vi "Strategy 5_Autotuning PID_With GUI.vi"() -> ()   [LabVIEW 2019]
doc: "This example demonstrates how to use the PID Design function to obtain PID parameters based on measured process."
uses:
  <vilib>/addons/control/pid/NI_PID_autopid.lvlib
  <vilib>/addons/control/pid/NI_PID_pid.lvlib
  <vilib>/ptbypt/NI_PtbyPt.lvlib
  <vilib>/DAQmx/create/channels.llb/DAQmx Create Channel (DO-Digital Output).vi
  <vilib>/DAQmx/write.llb/DAQmx Write (Digital 1D Bool 1Chan 1Samp).vi
  <vilib>/Instr/_visa.llb/VISA Configure Serial Port (Instr).vi
  <vilib>/addons/control/pid/autopid.llb/PID Autotuning Design (Cohen-Coon).vi
  <vilib>/addons/control/pid/autopid.llb/PID Autotuning Design (Ziegler-Nichols).vi
  <vilib>/addons/control/pid/autopid.llb/PID Autotuning Design (Chien-Hrones-Reswick).vi
  <vilib>/addons/control/pid/autopid.llb/PID Autotuning Design (Internal Model Control).vi
  <vilib>/addons/control/pid/pid.llb/PID Advanced (DBL).vi
  <vilib>/DAQmx/read.llb/DAQmx Read (Analog 1D DBL NChan 1Samp).vi
panel:
  out "Position Sensor Data 2":cluster{dbl, "x":sgl}[](graph)
  out "?":bool
  in  "Muscle Control":T1(tab)=enum."M-11"
  out "Tuned PID gains 12":T2={"proportional gain (Kc)"=1.9838195929127882, "integral time (Ti, min)"=0.01995856284686879, "derivative time (Td, min)"=0.0} {"derivative time (Td, min)" format="%#.6g"; "integral time (Ti, min)" format="%#.6g"; "proportional gain (Kc)" format="%#.6g"}
  in  "Accept gain 12":bool
  in  "Control 12":T3(tab)
  in  "Ziegler-Nichols speed 12":u16(ring) items=["Fast", "Normal", "Slow"]
  in  "Tuning specifications 12":u16(ring) items=["Regulator - 0 %", "Regulator -  20%", "Servo - 0%", "Servo - 20%"]
  in  "Multiplicative factor 12":dbl(slide)=1.0 scale=0.01..100.0
  in  "Type of controller 12":u16(ring)=2 items=["P", "PI", "PID"]
  in  "Stop 12":bool
  in  "PID Gains 12":T2={"proportional gain (Kc)"=0.1625, "integral time (Ti, min)"=1.25, "derivative time (Td, min)"=0.0} {"derivative time (Td, min)" format="%#.6g"; "integral time (Ti, min)" format="%#.6g"; "proportional gain (Kc)" format="%#.6g"}
  in  "Autotune 12":bool
  in  "Reinitialize 12":bool
  in  "Excitation 12":dbl=0.5 format="%.2f"
  in  "Automatic 12":bool=TRUE
  in  "MV: 12":dbl(slide)=20.39115328927357 scale=-100.0..100.0
  in  "Set Point 12":dbl(slide) scale=0.0..30.0
  out "PWM Output 12":bool
  out "Real time Data 12":dbl[][](graph)
  in  "Median sample length 21":i32=100
  in  "INLET 1 ON/OFF 3":bool=TRUE
  out "Tuned PID gains 11":T2={"proportional gain (Kc)"=1.9838195929127882, "integral time (Ti, min)"=0.01995856284686879, "derivative time (Td, min)"=0.0} {"derivative time (Td, min)" format="%#.6g"; "integral time (Ti, min)" format="%#.6g"; "proportional gain (Kc)" format="%#.6g"}
  in  "Accept gain 11":bool
  in  "Control 11":T3(tab)
  in  "Ziegler-Nichols speed 11":u16(ring) items=["Fast", "Normal", "Slow"]
  in  "Tuning specifications 11":u16(ring) items=["Regulator - 0 %", "Regulator -  20%", "Servo - 0%", "Servo - 20%"]
  in  "Multiplicative factor 11":dbl(slide)=1.0 scale=0.01..100.0
  in  "Type of controller 11":u16(ring)=2 items=["P", "PI", "PID"]
  in  "Excitation 11":dbl=0.5 format="%.2f"
  in  "Stop 11":bool
  in  "PID Gains 11":T2={"proportional gain (Kc)"=0.1625, "integral time (Ti, min)"=1.25, "derivative time (Td, min)"=0.0} {"derivative time (Td, min)" format="%#.6g"; "integral time (Ti, min)" format="%#.6g"; "proportional gain (Kc)" format="%#.6g"}
  in  "Autotune 11":bool
  in  "Reinitialize 11":bool
  in  "Automatic 11":bool=TRUE
  in  "MV: 11":dbl(slide)=20.39115328927357 scale=-100.0..100.0
  in  "Set Point 11":dbl(slide) scale=0.0..30.0
  out "PWM Output 11":bool
  out "Real time Data 11":dbl[][](graph)
  in  "Median sample length 20":i32=100
  in  "INLET 5 ON/OFF 3":bool=TRUE
  out "Tuned PID gains 10":T2={"proportional gain (Kc)"=1.9838195929127882, "integral time (Ti, min)"=0.01995856284686879, "derivative time (Td, min)"=0.0} {"derivative time (Td, min)" format="%#.6g"; "integral time (Ti, min)" format="%#.6g"; "proportional gain (Kc)" format="%#.6g"}
  in  "Accept gain 10":bool
  in  "Control 10":T3(tab)
  in  "Ziegler-Nichols speed 10":u16(ring) items=["Fast", "Normal", "Slow"]
  in  "Tuning specifications 10":u16(ring) items=["Regulator - 0 %", "Regulator -  20%", "Servo - 0%", "Servo - 20%"]
  in  "Multiplicative factor 10":dbl(slide)=1.0 scale=0.01..100.0
  in  "Type of controller 10":u16(ring)=2 items=["P", "PI", "PID"]
  in  "Stop 10":bool
  in  "PID Gains 10":T2={"proportional gain (Kc)"=0.1625, "integral time (Ti, min)"=1.25, "derivative time (Td, min)"=0.0} {"derivative time (Td, min)" format="%#.6g"; "integral time (Ti, min)" format="%#.6g"; "proportional gain (Kc)" format="%#.6g"}
  in  "Autotune 10":bool
  in  "Reinitialize 10":bool
  in  "Excitation 10":dbl=0.5 format="%.2f"
  in  "Automatic 10":bool=TRUE
  in  "MV: 10":dbl(slide)=20.39115328927357 scale=-100.0..100.0
  in  "Set Point 10":dbl(slide) scale=0.0..30.0
  out "PWM Output 10":bool
  out "Real time Data 10":dbl[][](graph)
  in  "Median sample length 19":i32=100
  in  "INLET 3 ON/OFF 3":bool=TRUE
  out "Tuned PID gains 9":T2={"proportional gain (Kc)"=1.9838195929127882, "integral time (Ti, min)"=0.01995856284686879, "derivative time (Td, min)"=0.0} {"derivative time (Td, min)" format="%#.6g"; "integral time (Ti, min)" format="%#.6g"; "proportional gain (Kc)" format="%#.6g"}
  in  "Accept gain 9":bool
  in  "Type of controller 9":u16(ring)=2 items=["P", "PI", "PID"]
  in  "Excitation 9":dbl=0.5 format="%.2f"
  in  "Control 9":T3(tab)
  in  "Ziegler-Nichols speed 9":u16(ring) items=["Fast", "Normal", "Slow"]
  in  "Tuning specifications 9":u16(ring) items=["Regulator - 0 %", "Regulator -  20%", "Servo - 0%", "Servo - 20%"]
  in  "Multiplicative factor 9":dbl(slide)=1.0 scale=0.01..100.0
  in  "Stop 9":bool
  in  "PID Gains 9":T2={"proportional gain (Kc)"=0.1625, "integral time (Ti, min)"=1.25, "derivative time (Td, min)"=0.0} {"derivative time (Td, min)" format="%#.6g"; "integral time (Ti, min)" format="%#.6g"; "proportional gain (Kc)" format="%#.6g"}
  in  "Autotune 9":bool
  in  "Reinitialize 9":bool
  in  "Automatic 9":bool=TRUE
  in  "MV: 9":dbl(slide)=20.39115328927357 scale=-100.0..100.0
  in  "Set Point 9":dbl(slide) scale=0.0..30.0
  out "PWM Output 9":bool
  out "Real time Data 9":dbl[][](graph)
  in  "Median sample length 18":i32=100
  in  "INLET 10 ON/OFF 2":bool=TRUE
  out "Tuned PID gains 8":T2={"proportional gain (Kc)"=1.9838195929127882, "integral time (Ti, min)"=0.01995856284686879, "derivative time (Td, min)"=0.0} {"derivative time (Td, min)" format="%#.6g"; "integral time (Ti, min)" format="%#.6g"; "proportional gain (Kc)" format="%#.6g"}
  in  "Accept gain 8":bool
  in  "Control 8":T3(tab)
  in  "Ziegler-Nichols speed 8":u16(ring) items=["Fast", "Normal", "Slow"]
  in  "Tuning specifications 8":u16(ring) items=["Regulator - 0 %", "Regulator -  20%", "Servo - 0%", "Servo - 20%"]
  in  "Multiplicative factor 8":dbl(slide)=1.0 scale=0.01..100.0
  in  "Type of controller 8":u16(ring)=2 items=["P", "PI", "PID"]
  in  "Stop 8":bool
  in  "PID Gains 8":T2={"proportional gain (Kc)"=0.1625, "integral time (Ti, min)"=1.25, "derivative time (Td, min)"=0.0} {"derivative time (Td, min)" format="%#.6g"; "integral time (Ti, min)" format="%#.6g"; "proportional gain (Kc)" format="%#.6g"}
  in  "Autotune 8":bool
  in  "Reinitialize 8":bool
  in  "Excitation 8":dbl=0.5 format="%.2f"
  in  "Automatic 8":bool=TRUE
  in  "MV: 8":dbl(slide)=20.39115328927357 scale=-100.0..100.0
  in  "Set Point 8":dbl(slide) scale=0.0..30.0
  out "PWM Output 8":bool
  out "Real time Data 8":dbl[][](graph)
  in  "Median sample length 17":i32=100
  in  "INLET 2 ON/OFF 2":bool=TRUE
  out "Tuned PID gains 7":T2={"proportional gain (Kc)"=1.9838195929127882, "integral time (Ti, min)"=0.01995856284686879, "derivative time (Td, min)"=0.0} {"derivative time (Td, min)" format="%#.6g"; "integral time (Ti, min)" format="%#.6g"; "proportional gain (Kc)" format="%#.6g"}
  in  "Accept gain 7":bool
  in  "Control 7":T3(tab)
  in  "Ziegler-Nichols speed 7":u16(ring) items=["Fast", "Normal", "Slow"]
  in  "Tuning specifications 7":u16(ring) items=["Regulator - 0 %", "Regulator -  20%", "Servo - 0%", "Servo - 20%"]
  in  "Multiplicative factor 7":dbl(slide)=1.0 scale=0.01..100.0
  in  "Type of controller 7":u16(ring)=2 items=["P", "PI", "PID"]
  in  "Stop 7":bool
  in  "PID Gains 7":T2={"proportional gain (Kc)"=0.1625, "integral time (Ti, min)"=1.25, "derivative time (Td, min)"=0.0} {"derivative time (Td, min)" format="%#.6g"; "integral time (Ti, min)" format="%#.6g"; "proportional gain (Kc)" format="%#.6g"}
  in  "Autotune 7":bool
  in  "Reinitialize 7":bool
  in  "Excitation 7":dbl=0.5 format="%.2f"
  in  "Automatic 7":bool=TRUE
  in  "MV: 7":dbl(slide)=20.39115328927357 scale=-100.0..100.0
  in  "Set Point 7":dbl(slide) scale=0.0..30.0
  out "PWM Output 7":bool
  out "Real time Data 7":dbl[][](graph)
  in  "Median sample length 16":i32=100
  in  "INLET 7 ON/OFF 2":bool=TRUE
  out "Tuned PID gains 6":T2={"proportional gain (Kc)"=1.9838195929127882, "integral time (Ti, min)"=0.01995856284686879, "derivative time (Td, min)"=0.0} {"derivative time (Td, min)" format="%#.6g"; "integral time (Ti, min)" format="%#.6g"; "proportional gain (Kc)" format="%#.6g"}
  in  "Accept gain 6":bool
  in  "Control 6":T3(tab)
  in  "Ziegler-Nichols speed 6":u16(ring) items=["Fast", "Normal", "Slow"]
  in  "Tuning specifications 6":u16(ring) items=["Regulator - 0 %", "Regulator -  20%", "Servo - 0%", "Servo - 20%"]
  in  "Multiplicative factor 6":dbl(slide)=1.0 scale=0.01..100.0
  in  "Type of controller 6":u16(ring)=2 items=["P", "PI", "PID"]
  in  "Stop 6":bool
  in  "PID Gains 6":T2={"proportional gain (Kc)"=0.1625, "integral time (Ti, min)"=1.25, "derivative time (Td, min)"=0.0} {"derivative time (Td, min)" format="%#.6g"; "integral time (Ti, min)" format="%#.6g"; "proportional gain (Kc)" format="%#.6g"}
  in  "Autotune 6":bool
  in  "Reinitialize 6":bool
  in  "Excitation 6":dbl=0.5 format="%.2f"
  in  "Automatic 6":bool=TRUE
  in  "MV: 6":dbl(slide)=20.39115328927357 scale=-100.0..100.0
  in  "Set Point 6":dbl(slide) scale=0.0..30.0
  out "PWM Output 6":bool
  out "Real time Data 6":dbl[][](graph)
  in  "Median sample length 15":i32=100
  in  "INLET 6 ON/OFF 2":bool=TRUE
  out "Tuned PID gains 5":T2={"proportional gain (Kc)"=1.9838195929127882, "integral time (Ti, min)"=0.01995856284686879, "derivative time (Td, min)"=0.0} {"derivative time (Td, min)" format="%#.6g"; "integral time (Ti, min)" format="%#.6g"; "proportional gain (Kc)" format="%#.6g"}
  in  "Accept gain 5":bool
  in  "Control 5":T3(tab)
  in  "Ziegler-Nichols speed 5":u16(ring) items=["Fast", "Normal", "Slow"]
  in  "Tuning specifications 5":u16(ring) items=["Regulator - 0 %", "Regulator -  20%", "Servo - 0%", "Servo - 20%"]
  in  "Multiplicative factor 5":dbl(slide)=1.0 scale=0.01..100.0
  in  "Type of controller 5":u16(ring)=2 items=["P", "PI", "PID"]
  in  "Stop 5":bool
  in  "PID Gains 5":T2={"proportional gain (Kc)"=0.1625, "integral time (Ti, min)"=1.25, "derivative time (Td, min)"=0.0} {"derivative time (Td, min)" format="%#.6g"; "integral time (Ti, min)" format="%#.6g"; "proportional gain (Kc)" format="%#.6g"}
  in  "Autotune 5":bool
  in  "Reinitialize 5":bool
  in  "Excitation 5":dbl=0.5 format="%.2f"
  in  "Automatic 5":bool=TRUE
  in  "MV: 5":dbl(slide)=20.39115328927357 scale=-100.0..100.0
  in  "Set Point 5":dbl(slide) scale=0.0..30.0
  out "PWM Output 5":bool
  out "Real time Data 5":dbl[][](graph)
  in  "Median sample length 14":i32=100
  in  "INLET 8 ON/OFF 2":bool=TRUE
  out "Tuned PID gains 4":T2={"proportional gain (Kc)"=1.9838195929127882, "integral time (Ti, min)"=0.01995856284686879, "derivative time (Td, min)"=0.0} {"derivative time (Td, min)" format="%#.6g"; "integral time (Ti, min)" format="%#.6g"; "proportional gain (Kc)" format="%#.6g"}
  in  "Accept gain 4":bool
  in  "Control 4":T3(tab)
  in  "Ziegler-Nichols speed 4":u16(ring) items=["Fast", "Normal", "Slow"]
  in  "Tuning specifications 4":u16(ring) items=["Regulator - 0 %", "Regulator -  20%", "Servo - 0%", "Servo - 20%"]
  in  "Multiplicative factor 4":dbl(slide)=1.0 scale=0.01..100.0
  in  "Type of controller 4":u16(ring)=2 items=["P", "PI", "PID"]
  in  "Stop 4":bool
  in  "PID Gains 4":T2={"proportional gain (Kc)"=0.1625, "integral time (Ti, min)"=1.25, "derivative time (Td, min)"=0.0} {"derivative time (Td, min)" format="%#.6g"; "integral time (Ti, min)" format="%#.6g"; "proportional gain (Kc)" format="%#.6g"}
  in  "Autotune 4":bool
  in  "Reinitialize 4":bool
  in  "Excitation 4":dbl=0.5 format="%.2f"
  in  "Automatic 4":bool=TRUE
  in  "MV: 4":dbl(slide)=20.39115328927357 scale=-100.0..100.0
  in  "Set Point 4":dbl(slide) scale=0.0..30.0
  out "PWM Output 4":bool
  out "Real time Data 4":dbl[][](graph)
  in  "Median sample length 9":i32=100
  in  "INLET 9 ON/OFF 2":bool=TRUE
  out "Tuned PID gains 3":T2={"proportional gain (Kc)"=1.9838195929127882, "integral time (Ti, min)"=0.01995856284686879, "derivative time (Td, min)"=0.0} {"derivative time (Td, min)" format="%#.6g"; "integral time (Ti, min)" format="%#.6g"; "proportional gain (Kc)" format="%#.6g"}
  in  "Accept gain 3":bool
  in  "Control 3":T3(tab)
  in  "Ziegler-Nichols speed 3":u16(ring) items=["Fast", "Normal", "Slow"]
  in  "Tuning specifications 3":u16(ring) items=["Regulator - 0 %", "Regulator -  20%", "Servo - 0%", "Servo - 20%"]
  in  "Multiplicative factor 3":dbl(slide)=1.0 scale=0.01..100.0
  in  "Type of controller 3":u16(ring)=2 items=["P", "PI", "PID"]
  in  "Stop 3":bool
  in  "PID Gains 3":T2={"proportional gain (Kc)"=0.1625, "integral time (Ti, min)"=1.25, "derivative time (Td, min)"=0.0} {"derivative time (Td, min)" format="%#.6g"; "integral time (Ti, min)" format="%#.6g"; "proportional gain (Kc)" format="%#.6g"}
  in  "Autotune 3":bool
  in  "Reinitialize 3":bool
  in  "Excitation 3":dbl=0.5 format="%.2f"
  in  "Automatic 3":bool=TRUE
  in  "MV: 3":dbl(slide)=20.39115328927357 scale=-100.0..100.0
  in  "Set Point 3":dbl(slide) scale=0.0..30.0
  out "PWM Output 3":bool
  out "Real time Data 3":dbl[][](graph)
  in  "Median sample length 13":i32=100
  in  "INLET 10 ON/OFF":bool=TRUE
  in  "INLET":bool=TRUE
  out "PWM Output":bool
  out "Real time Data":dbl[][](graph)
  in  "MV:":dbl(slide)=20.39115328927357 scale=-100.0..100.0
  in  "Set Point":dbl(slide) scale=0.0..30.0
  in  "Median sample length":i32=100
  in  "Excitation":dbl=0.5 format="%.2f"
  in  "Type of controller":u16(ring)=2 items=["P", "PI", "PID"]
  in  "Control":T3(tab)
  in  "Ziegler-Nichols speed":u16(ring) items=["Fast", "Normal", "Slow"]
  in  "Tuning specifications":u16(ring) items=["Regulator - 0 %", "Regulator -  20%", "Servo - 0%", "Servo - 20%"]
  in  "Multiplicative factor":dbl(slide)=1.0 scale=0.01..100.0
  in  "Automatic":bool=TRUE
  in  "Reinitialize":bool
  in  "Accept gain":bool
  out "Tuned PID gains":T2={"proportional gain (Kc)"=1.9838195929127882, "integral time (Ti, min)"=0.01995856284686879, "derivative time (Td, min)"=0.0} {"derivative time (Td, min)" format="%#.6g"; "integral time (Ti, min)" format="%#.6g"; "proportional gain (Kc)" format="%#.6g"}
  in  "Autotune":bool
  in  "PID Gains":T2={"proportional gain (Kc)"=0.1625, "integral time (Ti, min)"=1.25, "derivative time (Td, min)"=0.0} {"derivative time (Td, min)" format="%#.6g"; "integral time (Ti, min)" format="%#.6g"; "proportional gain (Kc)" format="%#.6g"}
  in  "Stop":bool
  out "Tuned PID gains 2":T2={"proportional gain (Kc)"=1.9838195929127882, "integral time (Ti, min)"=0.01995856284686879, "derivative time (Td, min)"=0.0} {"derivative time (Td, min)" format="%#.6g"; "integral time (Ti, min)" format="%#.6g"; "proportional gain (Kc)" format="%#.6g"}
  in  "Accept gain 2":bool
  in  "Control 2":T3(tab)
  in  "Ziegler-Nichols speed 2":u16(ring) items=["Fast", "Normal", "Slow"]
  in  "Tuning specifications 2":u16(ring) items=["Regulator - 0 %", "Regulator -  20%", "Servo - 0%", "Servo - 20%"]
  in  "Multiplicative factor 2":dbl(slide)=1.0 scale=0.01..100.0
  in  "Type of controller 2":u16(ring)=2 items=["P", "PI", "PID"]
  in  "Stop 2":bool
  in  "PID Gains 2":T2={"proportional gain (Kc)"=0.1625, "integral time (Ti, min)"=1.25, "derivative time (Td, min)"=0.0} {"derivative time (Td, min)" format="%#.6g"; "integral time (Ti, min)" format="%#.6g"; "proportional gain (Kc)" format="%#.6g"}
  in  "Autotune 2":bool
  in  "Reinitialize 2":bool
  in  "Excitation 2":dbl=0.5 format="%.2f"
  in  "Automatic 2":bool=TRUE
  in  "MV: 2":dbl(slide)=20.39115328927357 scale=-100.0..100.0
  in  "Set Point 2":dbl(slide) scale=0.0..30.0
  out "PWM Output 2":bool
  out "Real time Data 2":dbl[][](graph)
  in  "Median sample length 12":i32=100
  in  "INLET 12 ON/OFF":bool=TRUE
  in  "M-11":i32=5
  in  "M-12":i32=5
  in  "M-10":i32=5
  in  "M-9":i32=5
  in  "M-8":i32=5
  in  "M-6":i32=5
  in  "M-7":i32=5
  in  "M-2":i32=5
  in  "M-4":i32=5
  in  "M-3":i32=5
  in  "M-5":i32=5
  in  "M-1":i32=5
  out "Identified Plant Parameters":T4={"Plant Gain (K)"=1.7609511324977591, "Time Constant (T)"=1.9621978490901302, "Dead Time (L)"=0.22467425343567116}
  out "Control Output":dbl[](graph)
  out "Measurement":dbl[](graph)
  out "Stimulus operating point":dbl=20.314221540357543
  out "Response operating point":dbl=51.08345461694337
  out "Stimulus operating point 2":dbl=20.314221540357543
  out "Response operating point 2":dbl=51.08345461694337
  out "Identified Plant Parameters 2":T4={"Plant Gain (K)"=1.7609511324977591, "Time Constant (T)"=1.9621978490901302, "Dead Time (L)"=0.22467425343567116}
  out "Control Output 2":dbl[](graph)
  out "Measurement 2":dbl[](graph)
  out "Stimulus operating point 3":dbl=20.314221540357543
  out "Response operating point 3":dbl=51.08345461694337
  out "Identified Plant Parameters 3":T4={"Plant Gain (K)"=1.7609511324977591, "Time Constant (T)"=1.9621978490901302, "Dead Time (L)"=0.22467425343567116}
  out "Control Output 3":dbl[](graph)
  out "Measurement 3":dbl[](graph)
  out "Stimulus operating point 4":dbl=20.314221540357543
  out "Response operating point 4":dbl=51.08345461694337
  out "Identified Plant Parameters 4":T4={"Plant Gain (K)"=1.7609511324977591, "Time Constant (T)"=1.9621978490901302, "Dead Time (L)"=0.22467425343567116}
  out "Control Output 4":dbl[](graph)
  out "Measurement 4":dbl[](graph)
  out "Stimulus operating point 5":dbl=20.314221540357543
  out "Response operating point 5":dbl=51.08345461694337
  out "Identified Plant Parameters 5":T4={"Plant Gain (K)"=1.7609511324977591, "Time Constant (T)"=1.9621978490901302, "Dead Time (L)"=0.22467425343567116}
  out "Control Output 5":dbl[](graph)
  out "Measurement 5":dbl[](graph)
  out "Stimulus operating point 6":dbl=20.314221540357543
  out "Response operating point 6":dbl=51.08345461694337
  out "Identified Plant Parameters 6":T4={"Plant Gain (K)"=1.7609511324977591, "Time Constant (T)"=1.9621978490901302, "Dead Time (L)"=0.22467425343567116}
  out "Control Output 6":dbl[](graph)
  out "Measurement 6":dbl[](graph)
  out "Stimulus operating point 7":dbl=20.314221540357543
  out "Response operating point 7":dbl=51.08345461694337
  out "Identified Plant Parameters 7":T4={"Plant Gain (K)"=1.7609511324977591, "Time Constant (T)"=1.9621978490901302, "Dead Time (L)"=0.22467425343567116}
  out "Control Output 7":dbl[](graph)
  out "Measurement 7":dbl[](graph)
  out "Stimulus operating point 8":dbl=20.314221540357543
  out "Response operating point 8":dbl=51.08345461694337
  out "Identified Plant Parameters 8":T4={"Plant Gain (K)"=1.7609511324977591, "Time Constant (T)"=1.9621978490901302, "Dead Time (L)"=0.22467425343567116}
  out "Control Output 8":dbl[](graph)
  out "Measurement 8":dbl[](graph)
  out "Stimulus operating point 9":dbl=20.314221540357543
  out "Response operating point 9":dbl=51.08345461694337
  out "Identified Plant Parameters 9":T4={"Plant Gain (K)"=1.7609511324977591, "Time Constant (T)"=1.9621978490901302, "Dead Time (L)"=0.22467425343567116}
  out "Control Output 9":dbl[](graph)
  out "Measurement 9":dbl[](graph)
  out "Stimulus operating point 10":dbl=20.314221540357543
  out "Response operating point 10":dbl=51.08345461694337
  out "Identified Plant Parameters 10":T4={"Plant Gain (K)"=1.7609511324977591, "Time Constant (T)"=1.9621978490901302, "Dead Time (L)"=0.22467425343567116}
  out "Control Output 10":dbl[](graph)
  out "Measurement 10":dbl[](graph)
  out "Stimulus operating point 11":dbl=20.314221540357543
  out "Response operating point 11":dbl=51.08345461694337
  out "Identified Plant Parameters 11":T4={"Plant Gain (K)"=1.7609511324977591, "Time Constant (T)"=1.9621978490901302, "Dead Time (L)"=0.22467425343567116}
  out "Control Output 11":dbl[](graph)
  out "Measurement 11":dbl[](graph)
  out "Stimulus operating point 12":dbl=20.314221540357543
  out "Response operating point 12":dbl=51.08345461694337
  out "Identified Plant Parameters 12":T4={"Plant Gain (K)"=1.7609511324977591, "Time Constant (T)"=1.9621978490901302, "Dead Time (L)"=0.22467425343567116}
  out "Control Output 12":dbl[](graph)
  out "Measurement 12":dbl[](graph)
  in  "XYZAER":T5(array[cluster]) {"r" format="%1_6f"; "e" format="%1_6f"; "a" format="%1_6f"; "z" format="%1_6f"; "y" format="%1_6f"; "x" format="%1_6f"}
  out "Connected":bool
  out "Start Time Text":string
  out "Stop Time Text":string
  out "Elapsed Time Text":string
  out "HostFrameCount":u32
  out "Running":bool
  out "Loop Iter":i32
  out "PnoData":bool
  in  "stop":bool
  out "error out":errorcluster {"code" format="%.0x"}
  out "Position Sensor Data":cluster{dbl, "x":sgl}[](graph)
  out "Sensor Raw Value 2":i32
  in  "COM Port-Sensor 2":refnum<visa-resource-name>="COM5"
  in  "upper/lower infle":enum32{"Page 1", "Page 2"}(tab)
  out "Force in Kilograms":dbl(graph)
  out "Force in Newtons":dbl(graph)
  in  "lower/upper infle":enum32{"Page 1", "Page 2"}(tab)
  out "Force in Newtons 2":dbl(graph)
  out "Force in Kilograms 2":dbl(graph)
  in  "COM Port-Sensor 1":refnum<visa-resource-name>="COM4"
  out "Sensor Raw Value":i32
  in  "Tab Control":T6(tab)
  in  "Instructions":string="Overview: This example demonstrates how to use the PID Autotuning Design to obtain PID parameters based on setpoint and process variable collected in another loop.\nInstructions:\n1. Run the VI and wait until the process variable (PV) reaches near setpoint (SP).\n2.  In the PID Autotuning Design section, select the type of algorithm, type of controller and excitation amplitude for the 'open loop step response'. Then, click Autotune to start the process. Select the Identified Plant Parameter tab and see the results from the identification.\n3.  When the tuned PID gains do not change anymore, the identification is done and you have the option to accept by clicking Accept gain, which will transfer the new gain to PID Gains.\n4. Click the Autotune button again to go back to the automatic control state. You can try different options and repeat this process.\n5. Click Stop to stop the VI.\n"
  # "Pressure Alarm"
  # "Position Sensor Data"
  # "Force Sensor Data"
  # "PID Controller"
  # "PID Autotuning Design"
  # "No additional parameters"
  # "PID Controller"
  # "PID Autotuning Design"
  # "No additional parameters"
  # "PID Controller"
  # "PID Autotuning Design"
  # "No additional parameters"
  # "PID Controller"
  # "PID Autotuning Design"
  # "No additional parameters"
  # "PID Controller"
  # "PID Autotuning Design"
  # "No additional parameters"
  # "PID Controller"
  # "PID Autotuning Design"
  # "No additional parameters"
  # "PID Controller"
  # "PID Autotuning Design"
  # "No additional parameters"
  # "Muscle Control"
  # "PID Controller"
  # "PID Autotuning Design"
  # "No additional parameters"
  # "PID Controller"
  # "PID Autotuning Design"
  # "No additional parameters"
  # "PID Controller"
  # "PID Autotuning Design"
  # "No additional parameters"
  # "Muscle Control"
  # "PID Controller"
  # "PID Autotuning Design"
  # "No additional parameters"
  # "PID Controller"
  # "PID Autotuning Design"
  # "No additional parameters"
  # "Pressure Cut Off to trigger the alarm"
  # "M-11"
  # "M-12"
  # "M-10"
  # "M-9"
  # "M-8"
  # "M-6"
  # "M-7"
  # "M-2"
  # "M-4"
  # "M-3"
  # "M-5"
  # "M-1"
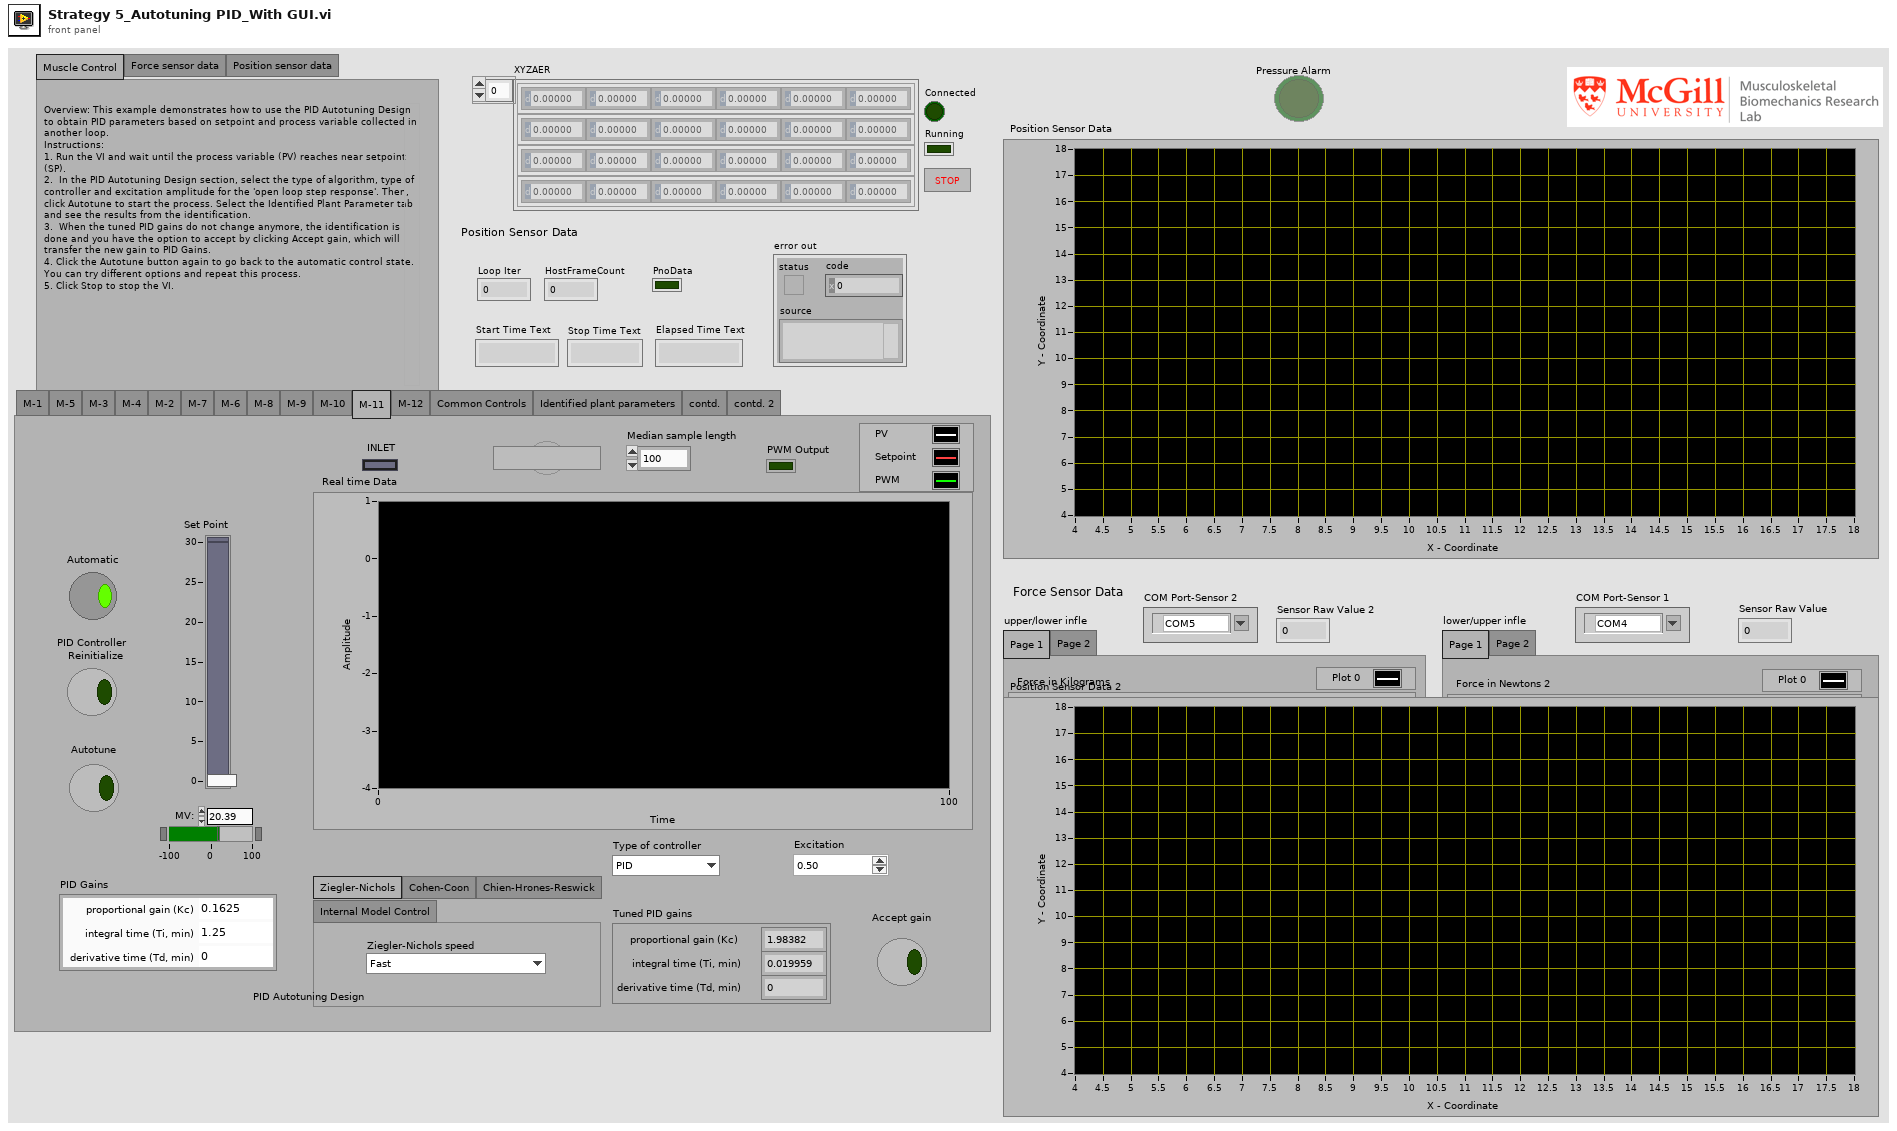
[diagram p1: front panel]
types:
  T1 = enum32{"M-1", "M-5", "M-3", "M-4", "M-2", "M-7", "M-6", "M-8", "M-9", "M-10", "M-11", "M-12", "Common Controls", "Identified plant parameters", "contd.", "contd. 2"}
  T2 = cluster{"proportional gain (Kc)":dbl, "integral time (Ti, min)":dbl, "derivative time (Td, min)":dbl}
  T3 = enum32{"Ziegler-Nichols", "Cohen-Coon", "Chien-Hrones-Reswick", "Internal Model Control"}
  T4 = cluster{"Plant Gain (K)":dbl, "Time Constant (T)":dbl, "Dead Time (L)":dbl}
  T5 = cluster{"x":sgl, "y":sgl, "z":sgl, "a":sgl, "e":sgl, "r":sgl}[]
  T6 = enum32{"Muscle Control", "Force sensor data", "Position sensor data"}
  T7 = cluster{"static gain":dbl, "lag (s)":dbl, "deadtime (s)":dbl, "load":dbl, "deadband":dbl, "sensor noise":dbl, "initial PV":dbl, "plant noise":dbl}
  T8 = cluster{"x":sgl, "y":sgl, "z":sgl, "a":sgl, "e":sgl, "r":sgl}
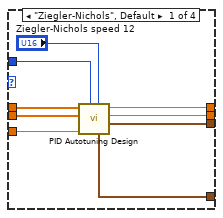
[diagram p2: hidden frame]
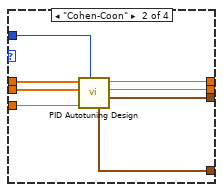
[diagram p3: hidden frame]
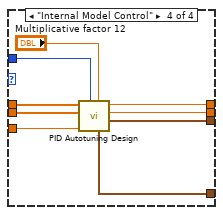
[diagram p4: hidden frame]
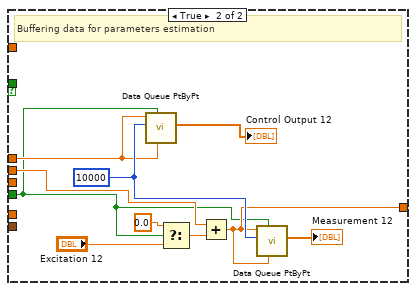
[diagram p6: hidden frame]
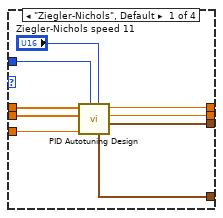
[diagram p7: hidden frame]
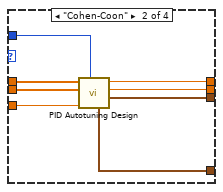
[diagram p8: hidden frame]
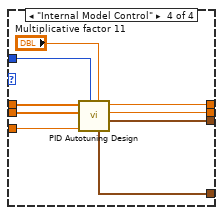
[diagram p9: hidden frame]
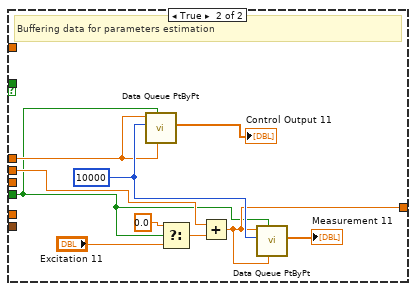
[diagram p11: hidden frame]
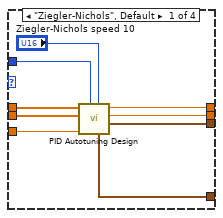
[diagram p12: hidden frame]
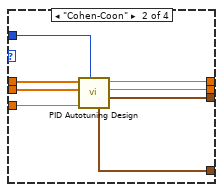
[diagram p13: hidden frame]
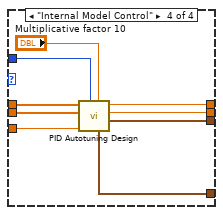
[diagram p14: hidden frame]
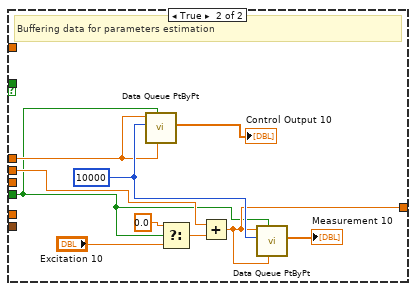
[diagram p16: hidden frame]
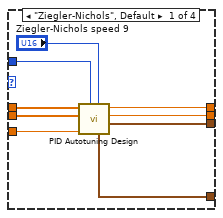
[diagram p17: hidden frame]
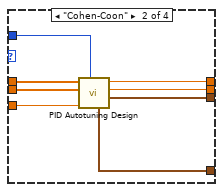
[diagram p18: hidden frame]
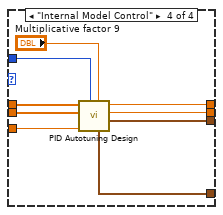
[diagram p19: hidden frame]
diagram:
  w37 = 0.0 ("output")
  w40 = FALSE ("Stop")
  w43 = 0.0 ("output")
  w46 = FALSE ("Stop")
  w49 = 0.0 ("output")
  w52 = FALSE ("Stop")
  w55 = 0.0 ("output")
  w58 = FALSE ("Stop")
  w61 = 0.0 ("output")
  w64 = FALSE ("Stop")
  w67 = 0.0 ("output")
  w70 = FALSE ("Stop")
  w73 = 0.0 ("output")
  w76 = FALSE ("Stop")
  w79 = 0.0 ("output")
  w82 = FALSE ("Stop")
  w85 = 0.0 ("output")
  w88 = FALSE ("Stop")
  w91 = 0.0 ("output")
  w94 = FALSE ("Stop")
  w97 = 0.0 ("output")
  w100 = FALSE ("Stop")
  w105 = 2400  # BufferFrameCount
  w139 = 0.0 ("output")
  w142 = FALSE ("Stop")
  # "Muscle-1 PID CONTROL LOOP (Auto Tuning)"
  # "Muscle-5 PID CONTROL LOOP (Auto Tuning)"
  # "Muscle-3 PID CONTROL LOOP (Auto Tuning)"
  # "Muscle-4 PID CONTROL LOOP (Auto Tuning)"
  # "Muscle-2 PID CONTROL LOOP (Auto Tuning)"
  # "Muscle-7 PID CONTROL LOOP (Auto Tuning)"
  # "Muscle-6 PID CONTROL LOOP (Auto Tuning)"
  # "Muscle-8 PID CONTROL LOOP (Auto Tuning)"
  # "Muscle-9 PID CONTROL LOOP (Auto Tuning)"
  # "Muscle-10 PID CONTROL LOOP (Auto Tuning)"
  # "Muscle-12 PID CONTROL LOOP (Auto Tuning)"
  # "Muscle-11 PID CONTROL LOOP (Auto Tuning)"
  # "FORCE SENSOR CONTROL LOOP"
  # "POSITION SENSOR CONTROL LOOP"
  # "Pressure Alarm"
  # "8. Close Tracker connection."
  # "3. Query Max num sensors supported by the tracker."
  # "4. Allocate raw buffer to hold 2400 frames of data."
  # "5. Start Continuous mode."
  # "7. Stop Continuous mode."
  # "6. Start the loop. Loop exits when Stop Button is hit."
  n1 = Obtain Queue(element data type=0.0) -> (queue out=w21:refnum<queue>)  [unwired: 4 in, 2 out]
  n2 = while {
    shift-left: 0.0 ("Plant Output") -> [w210]
    shift-right: [w205] -> _
    tunnel: w100 -> [_]
    shift-right: [w191] -> _
    shift-left: 0.01 -> [w189]
    shift-right: [w163] -> _
    shift-left: TRUE -> [w188]
    shift-right: [w165] -> _
    shift-left: w97 -> [w187]
    shift-right: [w190] -> _
    shift-left: w97 -> [w186]
    tunnel: [w160] -> w96
    tunnel: [w146] -> w33
    tunnel: w21 -> [w145]
    stop <- "Stop 2" stop-if-true
    w151 = 1 items=["one channel for each line", "one channel for all lines"] ("line grouping")
    w160 = 0.05 ("Sampling Time dt (s)")
    w169 = 1 items=["one channel for each line", "one channel for all lines"] ("line grouping")
    w177 = 0.5 ("x")
    w204 = T7 {"static gain"=2.5, "lag (s)"=2.5, "deadtime (s)"=0.01, "load"=0.0, "deadband"=0.0, "sensor noise"=0.0, "initial PV"=30.0, "plant noise"=0.0}  # Process parameters
    w206 = FALSE  # Integrator ?
    # "C."
    # "Inlet 11"
    # "Exhaust 12"
    # "B."
    # "A."
    # "A.Output to PWM Logic \nB. Simulated Plant\nC. Draw Chart"
    # "Main PID Loop Control"
    n3 = Multiply(x=w160, y=1000.0) -> (x*y=w203:dbl)
    n4 = Dequeue Element(queue=w145) -> (element=w144:dbl)  [unwired: 2 in, 3 out]
    n5 = Not(x="Autotune 2") -> (.not. x?=w207:bool)
    n6 = feedback #1() -> (w212:bool)  [unwired: 1 in]
    n7 = feedback-in #1("Autotune 2") -> ()
    n8 = Wait Until Next ms Multiple(millisecond multiple=w203) -> ()  [unwired: 1 out]
    n9 = Exclusive Or(1:w212, 2:"Autotune 2") -> (0:w211:bool)
    n10 = feedback #2() -> (w209:dbl)  [unwired: 1 in]
    n11 = Multiply(x=w144, y=-1000.0) -> (x*y=w193:dbl)
    n12 = call <vilib>:"Median PtByPt.vi"("sample length"="Median sample length 12", "x"=w193) -> ("median"=w192:dbl)  [unwired: 2 in, 1 out]
    n13 = Square(x=w192) -> (x^2=w200:dbl)
    n14 = Multiply(x=w192, y=-39.646) -> (x*y=w196:dbl)
    n15 = Multiply(x=w200, y=0.2324) -> (x*y=w197:dbl)
    n16 = Add(x=w196, y=w197) -> (x+y=w195:dbl)
    n17 = Add(x=1678.0, y=w195) -> (x+y=w158:dbl)
    n18 = case shown="False" "Autotune 2" {
      tunnel: w160 -> [w227 _]
      tunnel: [w216 w232] -> w165
      tunnel: w210 -> [_ w231]
      tunnel: "PID Gains 2" -> [w226 _]
      tunnel: "Reinitialize 2" -> [w223 _]
      tunnel: w211 -> [w225 w230]
      tunnel: w209 -> [_ w234]
      tunnel: w158 -> [w219 _]
      tunnel: "Set Point 2" -> [w218 _]
      frame False {
        # "This code is to have 'bumpless' transfer from autotuning"
        n19 = Not(x=w225) -> (.not. x?=w222:bool)
        n20 = And(x="Automatic 2", y=w222) -> (x .and. y?=w224:bool)
        n21 = call-poly <vilib>:"PID Advanced.vi"("setpoint"=w218, "auto? (T)"=w224, "manual control"="MV: 2", "process variable"=w219, "alpha"=10.0, "PID gains"=w226, "dt (s)"=w227, "reinitialize? (F)"=w223) -> ("output"=w216:dbl)  [unwired: 6 in, 1 out]
      }
      frame True {
        w237 = 10000 ("sample length")
        # "Buffering data for parameters estimation"
        n22 = call <vilib>:"Data Queue PtByPt.vi"("initial queue element"=w231, "initialize"=w230, "sample length"=w237, "input data point"=w231) -> ("Current Queue"=→"Control Output 2":dbl[])  [unwired: 3 in, 4 out]
        n23 = Select(t=0.0, s=w230, f="Excitation 2") -> (s? t:f=w235:dbl)
        n24 = Add(x=w234, y=w235) -> (x+y=w232:dbl)
        n25 = call <vilib>:"Data Queue PtByPt.vi"("initial queue element"=w232, "initialize"=w230, "sample length"=w237, "input data point"=w232) -> ("Current Queue"=→"Measurement 2":dbl[])  [unwired: 3 in, 4 out]
      }
    }
    n26 = feedback-in #2(w165, w207) -> ()
    n27 = Greater?(x=w158, y="M-12") -> (0:w146:bool)
    n28 = Add(x=w189, y=w177) -> (x+y=w178:dbl)
    n29 = Subtract(x=w189, y=w177) -> (x-y=w176:dbl)
    n30 = Equal?(x=w187, y=w165) -> (x = y?=w184:bool)
    n31 = Greater?(x=w165, y=w187) -> (0:w183:bool)
    n32 = Select(t=w188, s=w184, f=w183) -> (s? t:f=w163:bool)
    "PWM Output 2" <- w163
    n33 = call "Plant System.vi"("Integrator ?"=w206, "Plant Input"=w165, "dt (s)"=w160, "process parameters"=w204) -> ("Plant Output"=w205:dbl)  [unwired: 11 in]
    n34 = Increment(x="Set Point 2") -> (x+1=w182:dbl)
    n35 = Decrement(x="Set Point 2") -> (x-1=w181:dbl)
    n36 = Select(t=w178, s=w163, f=w176) -> (s? t:f=w191:dbl)
    n37 = Select(t=w182, s=w163, f=w181) -> (s? t:f=w180:dbl)
    n38 = Not(x=w163) -> (.not. x?=w162:bool)
    n39 = call-poly <vilib>:"DAQmx Create Virtual Channel.vi"("lines"=tag "cDAQ1Mod8/port0/line2", "line grouping"=w169) -> ("task out"=w171:refnum<k21>, "error out"=w170:errorcluster)  [unwired: 12 in]
    n40 = call-poly <vilib>:"DAQmx Create Virtual Channel.vi"("lines"=tag "cDAQ1Mod7/port0/line1", "line grouping"=w151) -> ("task out"=w153:refnum<k21>, "error out"=w152:errorcluster)  [unwired: 12 in]
    n41 = Build Array(w158, "Set Point 2", w180) -> (w179:dbl[])
    n42 = Initialize Array("INLET 12 ON/OFF", 1 ("dimension size")) -> (w148:bool[])
    n43 = Initialize Array(w162, 1 ("dimension size")) -> (w166:bool[])
    n44 = local write "MV: 2"(w165) -> ()
    n45 = Add(x=w186, y=w189) -> (x+y=w190:dbl)
    n46 = Build Array(w179) -> (→"Real time Data 2":dbl[][])
    n47 = call-poly <vilib>:"DAQmx Write.vi"("task/channels in"=w171, "auto start"=TRUE, "data"=w166, "error in"=w170) -> ("task out"=w173:refnum<k21>, "error out"=w174:errorcluster)  [unwired: 9 in, 1 out]
    n48 = call-poly <vilib>:"DAQmx Write.vi"("task/channels in"=w153, "auto start"=TRUE, "data"=w148, "error in"=w152) -> ("task out"=w155:refnum<k21>, "error out"=w156:errorcluster)  [unwired: 9 in, 1 out]
    n49 = call <vilib>:"DAQmx Clear Task.vi"("task in"=w173, "error in"=w174) -> ("error out"=w168:errorcluster)  [unwired: 13 in]
    n50 = call <vilib>:"DAQmx Clear Task.vi"("task in"=w155, "error in"=w156) -> ("error out"=w150:errorcluster)  [unwired: 13 in]
    n51 = call <vilib>:"Simple Error Handler.vi"("error in (no error)"=w168) -> ()  [unwired: 4 in, 5 out]
    n52 = call <vilib>:"Simple Error Handler.vi"("error in (no error)"=w150) -> ()  [unwired: 4 in, 5 out]
  }
  n53 = Obtain Queue(element data type=0.0) -> (queue out=w15:refnum<queue>)  [unwired: 4 in, 2 out]
  n54 = while {
    shift-left: 0.0 ("Plant Output") -> [w304]
    shift-right: [w299] -> _
    tunnel: w82 -> [_]
    shift-right: [w285] -> _
    shift-left: 0.01 -> [w283]
    shift-right: [w257] -> _
    shift-left: TRUE -> [w282]
    shift-right: [w259] -> _
    shift-left: w79 -> [w281]
    shift-right: [w284] -> _
    shift-left: w79 -> [w280]
    tunnel: [w254] -> w78
    tunnel: [w240] -> w30
    tunnel: w15 -> [w238]
    stop <- "Stop 5" stop-if-true
    w245 = 1 items=["one channel for each line", "one channel for all lines"] ("line grouping")
    w254 = 0.05 ("Sampling Time dt (s)")
    w263 = 1 items=["one channel for each line", "one channel for all lines"] ("line grouping")
    w271 = 0.5 ("x")
    w298 = T7 {"static gain"=2.5, "lag (s)"=2.5, "deadtime (s)"=0.01, "load"=0.0, "deadband"=0.0, "sensor noise"=0.0, "initial PV"=30.0, "plant noise"=0.0}  # Process parameters
    w300 = FALSE  # Integrator ?
    # "C."
    # "Inlet 11"
    # "Exhaust 8"
    # "B."
    # "A."
    # "A.Output to PWM Logic \nB. Simulated Plant\nC. Draw Chart"
    # "Main PID Loop Control"
    n55 = Dequeue Element(queue=w238) -> (element=w239:dbl)  [unwired: 2 in, 3 out]
    n56 = Multiply(x=w254, y=1000.0) -> (x*y=w297:dbl)
    n57 = Not(x="Autotune 5") -> (.not. x?=w301:bool)
    n58 = feedback #3() -> (w306:bool)  [unwired: 1 in]
    n59 = feedback-in #3("Autotune 5") -> ()
    n60 = Wait Until Next ms Multiple(millisecond multiple=w297) -> ()  [unwired: 1 out]
    n61 = Exclusive Or(1:w306, 2:"Autotune 5") -> (0:w305:bool)
    n62 = feedback #4() -> (w303:dbl)  [unwired: 1 in]
    n63 = Multiply(x=w239, y=-1000.0) -> (x*y=w287:dbl)
    n64 = call <vilib>:"Median PtByPt.vi"("sample length"="Median sample length 14", "x"=w287) -> ("median"=w286:dbl)  [unwired: 2 in, 1 out]
    n65 = Square(x=w286) -> (x^2=w294:dbl)
    n66 = Multiply(x=w286, y=16.572) -> (x*y=w290:dbl)
    n67 = Multiply(x=w294, y=-0.06) -> (x*y=w291:dbl)
    n68 = Add(x=w290, y=w291) -> (x+y=w289:dbl)
    n69 = Add(x=-1011.3, y=w289) -> (x+y=w252:dbl)
    n70 = case shown="False" "Autotune 5" {
      tunnel: w254 -> [w321 _]
      tunnel: [w310 w326] -> w259
      tunnel: w304 -> [_ w325]
      tunnel: "PID Gains 5" -> [w320 _]
      tunnel: "Reinitialize 5" -> [w317 _]
      tunnel: w305 -> [w319 w324]
      tunnel: w303 -> [_ w328]
      tunnel: w252 -> [w313 _]
      tunnel: "Set Point 5" -> [w312 _]
      frame False {
        # "This code is to have 'bumpless' transfer from autotuning"
        n71 = Not(x=w319) -> (.not. x?=w316:bool)
        n72 = And(x="Automatic 5", y=w316) -> (x .and. y?=w318:bool)
        n73 = call-poly <vilib>:"PID Advanced.vi"("setpoint"=w312, "auto? (T)"=w318, "manual control"="MV: 5", "process variable"=w313, "alpha"=10.0, "PID gains"=w320, "dt (s)"=w321, "reinitialize? (F)"=w317) -> ("output"=w310:dbl)  [unwired: 6 in, 1 out]
      }
      frame True {
        w331 = 10000 ("sample length")
        # "Buffering data for parameters estimation"
        n74 = call <vilib>:"Data Queue PtByPt.vi"("initial queue element"=w325, "initialize"=w324, "sample length"=w331, "input data point"=w325) -> ("Current Queue"=→"Control Output 5":dbl[])  [unwired: 3 in, 4 out]
        n75 = Select(t=0.0, s=w324, f="Excitation 5") -> (s? t:f=w329:dbl)
        n76 = Add(x=w328, y=w329) -> (x+y=w326:dbl)
        n77 = call <vilib>:"Data Queue PtByPt.vi"("initial queue element"=w326, "initialize"=w324, "sample length"=w331, "input data point"=w326) -> ("Current Queue"=→"Measurement 5":dbl[])  [unwired: 3 in, 4 out]
      }
    }
    n78 = feedback-in #4(w259, w301) -> ()
    n79 = Greater?(x=w252, y="M-8") -> (0:w240:bool)
    n80 = Add(x=w283, y=w271) -> (x+y=w272:dbl)
    n81 = Subtract(x=w283, y=w271) -> (x-y=w270:dbl)
    n82 = Equal?(x=w281, y=w259) -> (x = y?=w278:bool)
    n83 = Greater?(x=w259, y=w281) -> (0:w277:bool)
    n84 = Select(t=w282, s=w278, f=w277) -> (s? t:f=w257:bool)
    "PWM Output 5" <- w257
    n85 = call "Plant System.vi"("Integrator ?"=w300, "Plant Input"=w259, "dt (s)"=w254, "process parameters"=w298) -> ("Plant Output"=w299:dbl)  [unwired: 11 in]
    n86 = Increment(x="Set Point 5") -> (x+1=w276:dbl)
    n87 = Decrement(x="Set Point 5") -> (x-1=w275:dbl)
    n88 = Select(t=w272, s=w257, f=w270) -> (s? t:f=w285:dbl)
    n89 = Select(t=w276, s=w257, f=w275) -> (s? t:f=w274:dbl)
    n90 = Not(x=w257) -> (.not. x?=w256:bool)
    n91 = call-poly <vilib>:"DAQmx Create Virtual Channel.vi"("lines"=tag "cDAQ1Mod8/port0/line3", "line grouping"=w263) -> ("task out"=w265:refnum<k21>, "error out"=w264:errorcluster)  [unwired: 12 in]
    n92 = call-poly <vilib>:"DAQmx Create Virtual Channel.vi"("lines"=tag "cDAQ1Mod7/port0/line2", "line grouping"=w245) -> ("task out"=w247:refnum<k21>, "error out"=w246:errorcluster)  [unwired: 12 in]
    n93 = Build Array(w252, "Set Point 5", w274) -> (w273:dbl[])
    n94 = Initialize Array("INLET 8 ON/OFF 2", 1 ("dimension size")) -> (w242:bool[])
    n95 = Initialize Array(w256, 1 ("dimension size")) -> (w260:bool[])
    n96 = local write "MV: 5"(w259) -> ()
    n97 = Add(x=w280, y=w283) -> (x+y=w284:dbl)
    n98 = Build Array(w273) -> (→"Real time Data 5":dbl[][])
    n99 = call-poly <vilib>:"DAQmx Write.vi"("task/channels in"=w265, "auto start"=TRUE, "data"=w260, "error in"=w264) -> ("task out"=w267:refnum<k21>, "error out"=w268:errorcluster)  [unwired: 9 in, 1 out]
    n100 = call-poly <vilib>:"DAQmx Write.vi"("task/channels in"=w247, "auto start"=TRUE, "data"=w242, "error in"=w246) -> ("task out"=w249:refnum<k21>, "error out"=w250:errorcluster)  [unwired: 9 in, 1 out]
    n101 = call <vilib>:"DAQmx Clear Task.vi"("task in"=w267, "error in"=w268) -> ("error out"=w262:errorcluster)  [unwired: 13 in]
    n102 = call <vilib>:"DAQmx Clear Task.vi"("task in"=w249, "error in"=w250) -> ("error out"=w244:errorcluster)  [unwired: 13 in]
    n103 = call <vilib>:"Simple Error Handler.vi"("error in (no error)"=w262) -> ()  [unwired: 4 in, 5 out]
    n104 = call <vilib>:"Simple Error Handler.vi"("error in (no error)"=w244) -> ()  [unwired: 4 in, 5 out]
  }
  n105 = Obtain Queue(element data type=0.0) -> (queue out=w18:refnum<queue>)  [unwired: 4 in, 2 out]
  n106 = while {
    shift-left: 0.0 ("Plant Output") -> [w398]
    shift-right: [w393] -> _
    tunnel: w94 -> [_]
    shift-right: [w379] -> _
    shift-left: 0.01 -> [w377]
    shift-right: [w351] -> _
    shift-left: TRUE -> [w376]
    shift-right: [w353] -> _
    shift-left: w91 -> [w375]
    shift-right: [w378] -> _
    shift-left: w91 -> [w374]
    tunnel: [w348] -> w90
    tunnel: [w334] -> w32
    tunnel: w18 -> [w333]
    stop <- "Stop 3" stop-if-true
    w339 = 1 items=["one channel for each line", "one channel for all lines"] ("line grouping")
    w348 = 0.05 ("Sampling Time dt (s)")
    w357 = 1 items=["one channel for each line", "one channel for all lines"] ("line grouping")
    w365 = 0.5 ("x")
    w392 = T7 {"static gain"=2.5, "lag (s)"=2.5, "deadtime (s)"=0.01, "load"=0.0, "deadband"=0.0, "sensor noise"=0.0, "initial PV"=30.0, "plant noise"=0.0}  # Process parameters
    w394 = FALSE  # Integrator ?
    # "C."
    # "Inlet 11"
    # "Exhaust 10"
    # "B."
    # "A."
    # "A.Output to PWM Logic \nB. Simulated Plant\nC. Draw Chart"
    # "Main PID Loop Control"
    n107 = Multiply(x=w348, y=1000.0) -> (x*y=w391:dbl)
    n108 = Not(x="Autotune 3") -> (.not. x?=w395:bool)
    n109 = feedback #5() -> (w400:bool)  [unwired: 1 in]
    n110 = feedback-in #5("Autotune 3") -> ()
    n111 = Dequeue Element(queue=w333) -> (element=w332:dbl)  [unwired: 2 in, 3 out]
    n112 = Wait Until Next ms Multiple(millisecond multiple=w391) -> ()  [unwired: 1 out]
    n113 = Exclusive Or(1:w400, 2:"Autotune 3") -> (0:w399:bool)
    n114 = feedback #6() -> (w397:dbl)  [unwired: 1 in]
    n115 = Multiply(x=w332, y=-1000.0) -> (x*y=w381:dbl)
    n116 = call <vilib>:"Median PtByPt.vi"("sample length"="Median sample length 13", "x"=w381) -> ("median"=w380:dbl)  [unwired: 2 in, 1 out]
    n117 = Square(x=w380) -> (x^2=w388:dbl)
    n118 = Multiply(x=w380, y=16.572) -> (x*y=w384:dbl)
    n119 = Multiply(x=w388, y=-0.06) -> (x*y=w385:dbl)
    n120 = Add(x=w384, y=w385) -> (x+y=w383:dbl)
    n121 = Add(x=-1011.3, y=w383) -> (x+y=w346:dbl)
    n122 = case shown="False" "Autotune 3" {
      tunnel: w348 -> [w415 _]
      tunnel: [w404 w420] -> w353
      tunnel: w398 -> [_ w419]
      tunnel: "PID Gains 3" -> [w414 _]
      tunnel: "Reinitialize 3" -> [w411 _]
      tunnel: w399 -> [w413 w418]
      tunnel: w397 -> [_ w422]
      tunnel: w346 -> [w407 _]
      tunnel: "Set Point 3" -> [w406 _]
      frame False {
        # "This code is to have 'bumpless' transfer from autotuning"
        n123 = Not(x=w413) -> (.not. x?=w410:bool)
        n124 = And(x="Automatic 3", y=w410) -> (x .and. y?=w412:bool)
        n125 = call-poly <vilib>:"PID Advanced.vi"("setpoint"=w406, "auto? (T)"=w412, "manual control"="MV: 3", "process variable"=w407, "alpha"=10.0, "PID gains"=w414, "dt (s)"=w415, "reinitialize? (F)"=w411) -> ("output"=w404:dbl)  [unwired: 6 in, 1 out]
      }
      frame True {
        w425 = 10000 ("sample length")
        # "Buffering data for parameters estimation"
        n126 = call <vilib>:"Data Queue PtByPt.vi"("initial queue element"=w419, "initialize"=w418, "sample length"=w425, "input data point"=w419) -> ("Current Queue"=→"Control Output 3":dbl[])  [unwired: 3 in, 4 out]
        n127 = Select(t=0.0, s=w418, f="Excitation 3") -> (s? t:f=w423:dbl)
        n128 = Add(x=w422, y=w423) -> (x+y=w420:dbl)
        n129 = call <vilib>:"Data Queue PtByPt.vi"("initial queue element"=w420, "initialize"=w418, "sample length"=w425, "input data point"=w420) -> ("Current Queue"=→"Measurement 3":dbl[])  [unwired: 3 in, 4 out]
      }
    }
    n130 = feedback-in #6(w353, w395) -> ()
    n131 = Greater?(x=w346, y="M-10") -> (0:w334:bool)
    n132 = Add(x=w377, y=w365) -> (x+y=w366:dbl)
    n133 = Subtract(x=w377, y=w365) -> (x-y=w364:dbl)
    n134 = Equal?(x=w375, y=w353) -> (x = y?=w372:bool)
    n135 = Greater?(x=w353, y=w375) -> (0:w371:bool)
    n136 = Select(t=w376, s=w372, f=w371) -> (s? t:f=w351:bool)
    "PWM Output 3" <- w351
    n137 = call "Plant System.vi"("Integrator ?"=w394, "Plant Input"=w353, "dt (s)"=w348, "process parameters"=w392) -> ("Plant Output"=w393:dbl)  [unwired: 11 in]
    n138 = Increment(x="Set Point 3") -> (x+1=w370:dbl)
    n139 = Decrement(x="Set Point 3") -> (x-1=w369:dbl)
    n140 = Select(t=w366, s=w351, f=w364) -> (s? t:f=w379:dbl)
    n141 = Select(t=w370, s=w351, f=w369) -> (s? t:f=w368:dbl)
    n142 = Not(x=w351) -> (.not. x?=w350:bool)
    n143 = call-poly <vilib>:"DAQmx Create Virtual Channel.vi"("lines"=tag "cDAQ1Mod8/port0/line6", "line grouping"=w357) -> ("task out"=w359:refnum<k21>, "error out"=w358:errorcluster)  [unwired: 12 in]
    n144 = call-poly <vilib>:"DAQmx Create Virtual Channel.vi"("lines"=tag "cDAQ1Mod7/port0/line5", "line grouping"=w339) -> ("task out"=w341:refnum<k21>, "error out"=w340:errorcluster)  [unwired: 12 in]
    n145 = Build Array(w346, "Set Point 3", w368) -> (w367:dbl[])
    n146 = Initialize Array("INLET 10 ON/OFF", 1 ("dimension size")) -> (w336:bool[])
    n147 = Initialize Array(w350, 1 ("dimension size")) -> (w354:bool[])
    n148 = local write "MV: 3"(w353) -> ()
    n149 = Add(x=w374, y=w377) -> (x+y=w378:dbl)
    n150 = Build Array(w367) -> (→"Real time Data 3":dbl[][])
    n151 = call-poly <vilib>:"DAQmx Write.vi"("task/channels in"=w359, "auto start"=TRUE, "data"=w354, "error in"=w358) -> ("task out"=w361:refnum<k21>, "error out"=w362:errorcluster)  [unwired: 9 in, 1 out]
    n152 = call-poly <vilib>:"DAQmx Write.vi"("task/channels in"=w341, "auto start"=TRUE, "data"=w336, "error in"=w340) -> ("task out"=w343:refnum<k21>, "error out"=w344:errorcluster)  [unwired: 9 in, 1 out]
    n153 = call <vilib>:"DAQmx Clear Task.vi"("task in"=w361, "error in"=w362) -> ("error out"=w356:errorcluster)  [unwired: 13 in]
    n154 = call <vilib>:"DAQmx Clear Task.vi"("task in"=w343, "error in"=w344) -> ("error out"=w338:errorcluster)  [unwired: 13 in]
    n155 = call <vilib>:"Simple Error Handler.vi"("error in (no error)"=w356) -> ()  [unwired: 4 in, 5 out]
    n156 = call <vilib>:"Simple Error Handler.vi"("error in (no error)"=w338) -> ()  [unwired: 4 in, 5 out]
  }
  n157 = Obtain Queue(element data type=0.0) -> (queue out=w13:refnum<queue>)  [unwired: 4 in, 2 out]
  n158 = while {
    shift-left: 0.0 ("Plant Output") -> [w492]
    shift-right: [w487] -> _
    tunnel: w76 -> [_]
    shift-right: [w473] -> _
    shift-left: 0.01 -> [w471]
    shift-right: [w445] -> _
    shift-left: TRUE -> [w470]
    shift-right: [w447] -> _
    shift-left: w73 -> [w469]
    shift-right: [w472] -> _
    shift-left: w73 -> [w468]
    tunnel: [w442] -> w72
    tunnel: [w428] -> w29
    tunnel: w13 -> [w426]
    stop <- "Stop 6" stop-if-true
    w433 = 1 items=["one channel for each line", "one channel for all lines"] ("line grouping")
    w442 = 0.05 ("Sampling Time dt (s)")
    w451 = 1 items=["one channel for each line", "one channel for all lines"] ("line grouping")
    w459 = 0.5 ("x")
    w486 = T7 {"static gain"=2.5, "lag (s)"=2.5, "deadtime (s)"=0.01, "load"=0.0, "deadband"=0.0, "sensor noise"=0.0, "initial PV"=30.0, "plant noise"=0.0}  # Process parameters
    w488 = FALSE  # Integrator ?
    # "C."
    # "Inlet 11"
    # "Exhaust 6"
    # "B."
    # "A."
    # "A.Output to PWM Logic \nB. Simulated Plant\nC. Draw Chart"
    # "Main PID Loop Control"
    n159 = Dequeue Element(queue=w426) -> (element=w427:dbl)  [unwired: 2 in, 3 out]
    n160 = Multiply(x=w442, y=1000.0) -> (x*y=w485:dbl)
    n161 = Not(x="Autotune 6") -> (.not. x?=w489:bool)
    n162 = feedback #7() -> (w494:bool)  [unwired: 1 in]
    n163 = feedback-in #7("Autotune 6") -> ()
    n164 = Wait Until Next ms Multiple(millisecond multiple=w485) -> ()  [unwired: 1 out]
    n165 = Exclusive Or(1:w494, 2:"Autotune 6") -> (0:w493:bool)
    n166 = feedback #8() -> (w491:dbl)  [unwired: 1 in]
    n167 = Multiply(x=w427, y=-1000.0) -> (x*y=w475:dbl)
    n168 = call <vilib>:"Median PtByPt.vi"("sample length"="Median sample length 15", "x"=w475) -> ("median"=w474:dbl)  [unwired: 2 in, 1 out]
    n169 = Square(x=w474) -> (x^2=w482:dbl)
    n170 = Multiply(x=w474, y=16.572) -> (x*y=w478:dbl)
    n171 = Multiply(x=w482, y=-0.06) -> (x*y=w479:dbl)
    n172 = Add(x=w478, y=w479) -> (x+y=w477:dbl)
    n173 = Add(x=-1011.3, y=w477) -> (x+y=w440:dbl)
    n174 = case shown="False" "Autotune 6" {
      tunnel: w442 -> [w509 _]
      tunnel: [w498 w514] -> w447
      tunnel: w492 -> [_ w513]
      tunnel: "PID Gains 6" -> [w508 _]
      tunnel: "Reinitialize 6" -> [w505 _]
      tunnel: w493 -> [w507 w512]
      tunnel: w491 -> [_ w516]
      tunnel: w440 -> [w501 _]
      tunnel: "Set Point 6" -> [w500 _]
      frame False {
        # "This code is to have 'bumpless' transfer from autotuning"
        n175 = Not(x=w507) -> (.not. x?=w504:bool)
        n176 = And(x="Automatic 6", y=w504) -> (x .and. y?=w506:bool)
        n177 = call-poly <vilib>:"PID Advanced.vi"("setpoint"=w500, "auto? (T)"=w506, "manual control"="MV: 6", "process variable"=w501, "alpha"=10.0, "PID gains"=w508, "dt (s)"=w509, "reinitialize? (F)"=w505) -> ("output"=w498:dbl)  [unwired: 6 in, 1 out]
      }
      frame True {
        w519 = 10000 ("sample length")
        # "Buffering data for parameters estimation"
        n178 = call <vilib>:"Data Queue PtByPt.vi"("initial queue element"=w513, "initialize"=w512, "sample length"=w519, "input data point"=w513) -> ("Current Queue"=→"Control Output 6":dbl[])  [unwired: 3 in, 4 out]
        n179 = Select(t=0.0, s=w512, f="Excitation 6") -> (s? t:f=w517:dbl)
        n180 = Add(x=w516, y=w517) -> (x+y=w514:dbl)
        n181 = call <vilib>:"Data Queue PtByPt.vi"("initial queue element"=w514, "initialize"=w512, "sample length"=w519, "input data point"=w514) -> ("Current Queue"=→"Measurement 6":dbl[])  [unwired: 3 in, 4 out]
      }
    }
    n182 = feedback-in #8(w447, w489) -> ()
    n183 = Greater?(x=w440, y="M-6") -> (0:w428:bool)
    n184 = Add(x=w471, y=w459) -> (x+y=w460:dbl)
    n185 = Subtract(x=w471, y=w459) -> (x-y=w458:dbl)
    n186 = Equal?(x=w469, y=w447) -> (x = y?=w466:bool)
    n187 = Greater?(x=w447, y=w469) -> (0:w465:bool)
    n188 = Select(t=w470, s=w466, f=w465) -> (s? t:f=w445:bool)
    "PWM Output 6" <- w445
    n189 = call "Plant System.vi"("Integrator ?"=w488, "Plant Input"=w447, "dt (s)"=w442, "process parameters"=w486) -> ("Plant Output"=w487:dbl)  [unwired: 11 in]
    n190 = Increment(x="Set Point 6") -> (x+1=w464:dbl)
    n191 = Decrement(x="Set Point 6") -> (x-1=w463:dbl)
    n192 = Select(t=w460, s=w445, f=w458) -> (s? t:f=w473:dbl)
    n193 = Select(t=w464, s=w445, f=w463) -> (s? t:f=w462:dbl)
    n194 = Not(x=w445) -> (.not. x?=w444:bool)
    n195 = call-poly <vilib>:"DAQmx Create Virtual Channel.vi"("lines"=tag "cDAQ1Mod1/port0/line4", "line grouping"=w451) -> ("task out"=w453:refnum<k21>, "error out"=w452:errorcluster)  [unwired: 12 in]
    n196 = call-poly <vilib>:"DAQmx Create Virtual Channel.vi"("lines"=tag "cDAQ1Mod2/port0/line4", "line grouping"=w433) -> ("task out"=w435:refnum<k21>, "error out"=w434:errorcluster)  [unwired: 12 in]
    n197 = Build Array(w440, "Set Point 6", w462) -> (w461:dbl[])
    n198 = Initialize Array("INLET 6 ON/OFF 2", 1 ("dimension size")) -> (w430:bool[])
    n199 = Initialize Array(w444, 1 ("dimension size")) -> (w448:bool[])
    n200 = local write "MV: 6"(w447) -> ()
    n201 = Add(x=w468, y=w471) -> (x+y=w472:dbl)
    n202 = Build Array(w461) -> (→"Real time Data 6":dbl[][])
    n203 = call-poly <vilib>:"DAQmx Write.vi"("task/channels in"=w453, "auto start"=TRUE, "data"=w448, "error in"=w452) -> ("task out"=w455:refnum<k21>, "error out"=w456:errorcluster)  [unwired: 9 in, 1 out]
    n204 = call-poly <vilib>:"DAQmx Write.vi"("task/channels in"=w435, "auto start"=TRUE, "data"=w430, "error in"=w434) -> ("task out"=w437:refnum<k21>, "error out"=w438:errorcluster)  [unwired: 9 in, 1 out]
    n205 = call <vilib>:"DAQmx Clear Task.vi"("task in"=w455, "error in"=w456) -> ("error out"=w450:errorcluster)  [unwired: 13 in]
    n206 = call <vilib>:"DAQmx Clear Task.vi"("task in"=w437, "error in"=w438) -> ("error out"=w432:errorcluster)  [unwired: 13 in]
    n207 = call <vilib>:"Simple Error Handler.vi"("error in (no error)"=w450) -> ()  [unwired: 4 in, 5 out]
    n208 = call <vilib>:"Simple Error Handler.vi"("error in (no error)"=w432) -> ()  [unwired: 4 in, 5 out]
  }
  n209 = Obtain Queue(element data type=0.0) -> (queue out=w17:refnum<queue>)  [unwired: 4 in, 2 out]
  n210 = while {
    shift-left: 0.0 ("Plant Output") -> [w586]
    shift-right: [w581] -> _
    tunnel: w88 -> [_]
    shift-right: [w567] -> _
    shift-left: 0.01 -> [w565]
    shift-right: [w539] -> _
    shift-left: TRUE -> [w564]
    shift-right: [w541] -> _
    shift-left: w85 -> [w563]
    shift-right: [w566] -> _
    shift-left: w85 -> [w562]
    tunnel: [w536] -> w84
    tunnel: [w522] -> w31
    tunnel: w17 -> [w520]
    stop <- "Stop 4" stop-if-true
    w527 = 1 items=["one channel for each line", "one channel for all lines"] ("line grouping")
    w536 = 0.05 ("Sampling Time dt (s)")
    w545 = 1 items=["one channel for each line", "one channel for all lines"] ("line grouping")
    w553 = 0.5 ("x")
    w580 = T7 {"static gain"=2.5, "lag (s)"=2.5, "deadtime (s)"=0.01, "load"=0.0, "deadband"=0.0, "sensor noise"=0.0, "initial PV"=30.0, "plant noise"=0.0}  # Process parameters
    w582 = FALSE  # Integrator ?
    # "C."
    # "Inlet 11"
    # "Exhaust 9"
    # "B."
    # "A."
    # "A.Output to PWM Logic \nB. Simulated Plant\nC. Draw Chart"
    # "Main PID Loop Control"
    n211 = Dequeue Element(queue=w520) -> (element=w521:dbl)  [unwired: 2 in, 3 out]
    n212 = Multiply(x=w536, y=1000.0) -> (x*y=w579:dbl)
    n213 = Not(x="Autotune 4") -> (.not. x?=w583:bool)
    n214 = feedback #9() -> (w588:bool)  [unwired: 1 in]
    n215 = feedback-in #9("Autotune 4") -> ()
    n216 = Wait Until Next ms Multiple(millisecond multiple=w579) -> ()  [unwired: 1 out]
    n217 = Exclusive Or(1:w588, 2:"Autotune 4") -> (0:w587:bool)
    n218 = feedback #10() -> (w585:dbl)  [unwired: 1 in]
    n219 = Multiply(x=w521, y=-1000.0) -> (x*y=w569:dbl)
    n220 = call <vilib>:"Median PtByPt.vi"("sample length"="Median sample length 9", "x"=w569) -> ("median"=w568:dbl)  [unwired: 2 in, 1 out]
    n221 = Square(x=w568) -> (x^2=w576:dbl)
    n222 = Multiply(x=w568, y=16.572) -> (x*y=w572:dbl)
    n223 = Multiply(x=w576, y=-0.06) -> (x*y=w573:dbl)
    n224 = Add(x=w572, y=w573) -> (x+y=w571:dbl)
    n225 = Add(x=-1011.3, y=w571) -> (x+y=w534:dbl)
    n226 = case shown="False" "Autotune 4" {
      tunnel: w536 -> [w603 _]
      tunnel: [w592 w608] -> w541
      tunnel: w586 -> [_ w607]
      tunnel: "PID Gains 4" -> [w602 _]
      tunnel: "Reinitialize 4" -> [w599 _]
      tunnel: w587 -> [w601 w606]
      tunnel: w585 -> [_ w610]
      tunnel: w534 -> [w595 _]
      tunnel: "Set Point 4" -> [w594 _]
      frame False {
        # "This code is to have 'bumpless' transfer from autotuning"
        n227 = Not(x=w601) -> (.not. x?=w598:bool)
        n228 = And(x="Automatic 4", y=w598) -> (x .and. y?=w600:bool)
        n229 = call-poly <vilib>:"PID Advanced.vi"("setpoint"=w594, "auto? (T)"=w600, "manual control"="MV: 4", "process variable"=w595, "alpha"=10.0, "PID gains"=w602, "dt (s)"=w603, "reinitialize? (F)"=w599) -> ("output"=w592:dbl)  [unwired: 6 in, 1 out]
      }
      frame True {
        w613 = 10000 ("sample length")
        # "Buffering data for parameters estimation"
        n230 = call <vilib>:"Data Queue PtByPt.vi"("initial queue element"=w607, "initialize"=w606, "sample length"=w613, "input data point"=w607) -> ("Current Queue"=→"Control Output 4":dbl[])  [unwired: 3 in, 4 out]
        n231 = Select(t=0.0, s=w606, f="Excitation 4") -> (s? t:f=w611:dbl)
        n232 = Add(x=w610, y=w611) -> (x+y=w608:dbl)
        n233 = call <vilib>:"Data Queue PtByPt.vi"("initial queue element"=w608, "initialize"=w606, "sample length"=w613, "input data point"=w608) -> ("Current Queue"=→"Measurement 4":dbl[])  [unwired: 3 in, 4 out]
      }
    }
    n234 = feedback-in #10(w541, w583) -> ()
    n235 = Greater?(x=w534, y="M-9") -> (0:w522:bool)
    n236 = Add(x=w565, y=w553) -> (x+y=w554:dbl)
    n237 = Subtract(x=w565, y=w553) -> (x-y=w552:dbl)
    n238 = Equal?(x=w563, y=w541) -> (x = y?=w560:bool)
    n239 = Greater?(x=w541, y=w563) -> (0:w559:bool)
    n240 = Select(t=w564, s=w560, f=w559) -> (s? t:f=w539:bool)
    "PWM Output 4" <- w539
    n241 = call "Plant System.vi"("Integrator ?"=w582, "Plant Input"=w541, "dt (s)"=w536, "process parameters"=w580) -> ("Plant Output"=w581:dbl)  [unwired: 11 in]
    n242 = Increment(x="Set Point 4") -> (x+1=w558:dbl)
    n243 = Decrement(x="Set Point 4") -> (x-1=w557:dbl)
    n244 = Select(t=w554, s=w539, f=w552) -> (s? t:f=w567:dbl)
    n245 = Select(t=w558, s=w539, f=w557) -> (s? t:f=w556:dbl)
    n246 = Not(x=w539) -> (.not. x?=w538:bool)
    n247 = call-poly <vilib>:"DAQmx Create Virtual Channel.vi"("lines"=tag "cDAQ1Mod1/port0/line3", "line grouping"=w545) -> ("task out"=w547:refnum<k21>, "error out"=w546:errorcluster)  [unwired: 12 in]
    n248 = call-poly <vilib>:"DAQmx Create Virtual Channel.vi"("lines"=tag "cDAQ1Mod2/port0/line3", "line grouping"=w527) -> ("task out"=w529:refnum<k21>, "error out"=w528:errorcluster)  [unwired: 12 in]
    n249 = Build Array(w534, "Set Point 4", w556) -> (w555:dbl[])
    n250 = Initialize Array("INLET 9 ON/OFF 2", 1 ("dimension size")) -> (w524:bool[])
    n251 = Initialize Array(w538, 1 ("dimension size")) -> (w542:bool[])
    n252 = local write "MV: 4"(w541) -> ()
    n253 = Add(x=w562, y=w565) -> (x+y=w566:dbl)
    n254 = Build Array(w555) -> (→"Real time Data 4":dbl[][])
    n255 = call-poly <vilib>:"DAQmx Write.vi"("task/channels in"=w547, "auto start"=TRUE, "data"=w542, "error in"=w546) -> ("task out"=w549:refnum<k21>, "error out"=w550:errorcluster)  [unwired: 9 in, 1 out]
    n256 = call-poly <vilib>:"DAQmx Write.vi"("task/channels in"=w529, "auto start"=TRUE, "data"=w524, "error in"=w528) -> ("task out"=w531:refnum<k21>, "error out"=w532:errorcluster)  [unwired: 9 in, 1 out]
    n257 = call <vilib>:"DAQmx Clear Task.vi"("task in"=w549, "error in"=w550) -> ("error out"=w544:errorcluster)  [unwired: 13 in]
    n258 = call <vilib>:"DAQmx Clear Task.vi"("task in"=w531, "error in"=w532) -> ("error out"=w526:errorcluster)  [unwired: 13 in]
    n259 = call <vilib>:"Simple Error Handler.vi"("error in (no error)"=w544) -> ()  [unwired: 4 in, 5 out]
    n260 = call <vilib>:"Simple Error Handler.vi"("error in (no error)"=w526) -> ()  [unwired: 4 in, 5 out]
  }
  n261 = local write "Stop 6"(w76) -> ()
  n262 = local write "Stop 4"(w88) -> ()
  n263 = local write "Stop 3"(w94) -> ()
  n264 = local write "Stop 5"(w82) -> ()
  n265 = local write "Stop 2"(w100) -> ()
  n266 = local write "Stop"(w142) -> ()
  n267 = call-poly "VISA Configure Serial Port"("VISA resource name"="COM Port-Sensor 1") -> ("VISA resource name out"=w133:refnum<visa-resource-name>, "error out"=w132:errorcluster)  [unwired: 9 in, 4 out]
  n268 = call-poly "VISA Configure Serial Port"("VISA resource name"="COM Port-Sensor 2") -> ("VISA resource name out"=w128:refnum<visa-resource-name>, "error out"=w127:errorcluster)  [unwired: 9 in, 4 out]
  n269 = while {
    tunnel: w76 -> [_]
    tunnel: w72 -> [w617]
    stop <- w627 stop-if-true
    # "If dT and deadtime have similar values, the identification could evaluate deadtime as zero and this generates proportional gain equal to Inf. This code avoid gain changes in this situations."
    # "Autotuning Loop"
    n270 = local read "Control Output 6"() -> (w629:dbl[])
    n271 = local read "Measurement 6"() -> (w628:dbl[])
    n272 = case shown="\"Chien-Hrones-Reswick\"" "Control 6" {
      tunnel: w629 -> [w638 w646 w655 w664]
      tunnel: w628 -> [w637 w645 w654 w663]
      tunnel: [w636 w644 w653 w662] -> w616
      tunnel: [w635 w643 w652 w661] -> w615
      tunnel: w617 -> [w634 w642 w651 w660]
      tunnel: [w633 w641 w650 w659] -> w614
      tunnel: [w632 w640 w649 w658] -> w619
      tunnel: "Type of controller 6" -> [w631 w639 w648 w657]
      frame "Ziegler-Nichols", Default {
        n273 = call-poly <vilib>:"PID Autotuning Design.vi"("Ziegler-Nichols Speed"="Ziegler-Nichols speed 6", "Type of Controller"=w631, "dt (s)"=w634, "Response signal"=w637, "Stimulus signal"=w638) -> ("PID gains"=w632:T2, "response operating point"=w635:dbl, "stimulus operating point"=w636:dbl, "Plant Parameters"=w633:T4)  [unwired: 3 in]
      }
      frame "Cohen-Coon" {
        n274 = call-poly <vilib>:"PID Autotuning Design.vi"("Type of Controller"=w639, "dt (s)"=w642, "Response signal"=w645, "Stimulus signal"=w646) -> ("PID gains"=w640:T2, "response offset"=w643:dbl, "stimulus offset"=w644:dbl, "Plant Parameters"=w641:T4)  [unwired: 4 in]
      }
      frame "Chien-Hrones-Reswick" {
        n275 = call-poly <vilib>:"PID Autotuning Design.vi"("Tuning specifications"="Tuning specifications 6", "Type of Controller"=w648, "dt (s)"=w651, "Response signal"=w654, "Stimulus signal"=w655) -> ("PID gains"=w649:T2, "response offset"=w652:dbl, "stimulus offset"=w653:dbl, "Plant Parameters"=w650:T4)  [unwired: 3 in]
      }
      frame "Internal Model Control" {
        n276 = call-poly <vilib>:"PID Autotuning Design.vi"("Desired Time Constant (tau_c)"="Multiplicative factor 6", "Type of Controller"=w657, "dt (s)"=w660, "Response signal"=w663, "Stimulus signal"=w664) -> ("PID gains"=w658:T2, "response offset"=w661:dbl, "stimulus offset"=w662:dbl, "Plant Parameters"=w659:T4)  [unwired: 3 in]
      }
    }
    "Stimulus operating point 6" <- w616
    "Response operating point 6" <- w615
    "Identified Plant Parameters 6" <- w614
    n277 = Unbundle(w619) -> ("proportional gain (Kc)"=w622:dbl)  [unwired: 2 out]
    n278 = Equal?(x=w622, y=inf) -> (x = y?=w621:bool)
    n279 = feedback #11() -> (w620:T2)  [unwired: 1 in]
    n280 = Select(t=w620, s=w621, f=w619) -> (s? t:f=w618:T2)
    "Tuned PID gains 6" <- w618
    n281 = feedback-in #11(w618) -> ()
    n282 = case shown="True" "Accept gain 6" {
      tunnel: w618 -> [_ w665]
      frame False {
      }
      frame True {
        n283 = local write "PID Gains 6"(w665) -> ()
      }
    }
    n284 = local read "Stop 6"() -> (w627:bool)
  }
  n285 = while {
    tunnel: w88 -> [_]
    tunnel: w84 -> [w669]
    stop <- w679 stop-if-true
    # "If dT and deadtime have similar values, the identification could evaluate deadtime as zero and this generates proportional gain equal to Inf. This code avoid gain changes in this situations."
    # "Autotuning Loop"
    n286 = local read "Control Output 4"() -> (w681:dbl[])
    n287 = local read "Measurement 4"() -> (w680:dbl[])
    n288 = case shown="\"Chien-Hrones-Reswick\"" "Control 4" {
      tunnel: w681 -> [w690 w698 w707 w716]
      tunnel: w680 -> [w689 w697 w706 w715]
      tunnel: [w688 w696 w705 w714] -> w668
      tunnel: [w687 w695 w704 w713] -> w667
      tunnel: w669 -> [w686 w694 w703 w712]
      tunnel: [w685 w693 w702 w711] -> w666
      tunnel: [w684 w692 w701 w710] -> w671
      tunnel: "Type of controller 4" -> [w683 w691 w700 w709]
      frame "Ziegler-Nichols", Default {
        n289 = call-poly <vilib>:"PID Autotuning Design.vi"("Ziegler-Nichols Speed"="Ziegler-Nichols speed 4", "Type of Controller"=w683, "dt (s)"=w686, "Response signal"=w689, "Stimulus signal"=w690) -> ("PID gains"=w684:T2, "response operating point"=w687:dbl, "stimulus operating point"=w688:dbl, "Plant Parameters"=w685:T4)  [unwired: 3 in]
      }
      frame "Cohen-Coon" {
        n290 = call-poly <vilib>:"PID Autotuning Design.vi"("Type of Controller"=w691, "dt (s)"=w694, "Response signal"=w697, "Stimulus signal"=w698) -> ("PID gains"=w692:T2, "response offset"=w695:dbl, "stimulus offset"=w696:dbl, "Plant Parameters"=w693:T4)  [unwired: 4 in]
      }
      frame "Chien-Hrones-Reswick" {
        n291 = call-poly <vilib>:"PID Autotuning Design.vi"("Tuning specifications"="Tuning specifications 4", "Type of Controller"=w700, "dt (s)"=w703, "Response signal"=w706, "Stimulus signal"=w707) -> ("PID gains"=w701:T2, "response offset"=w704:dbl, "stimulus offset"=w705:dbl, "Plant Parameters"=w702:T4)  [unwired: 3 in]
      }
      frame "Internal Model Control" {
        n292 = call-poly <vilib>:"PID Autotuning Design.vi"("Desired Time Constant (tau_c)"="Multiplicative factor 4", "Type of Controller"=w709, "dt (s)"=w712, "Response signal"=w715, "Stimulus signal"=w716) -> ("PID gains"=w710:T2, "response offset"=w713:dbl, "stimulus offset"=w714:dbl, "Plant Parameters"=w711:T4)  [unwired: 3 in]
      }
    }
    "Stimulus operating point 4" <- w668
    "Response operating point 4" <- w667
    "Identified Plant Parameters 4" <- w666
    n293 = Unbundle(w671) -> ("proportional gain (Kc)"=w674:dbl)  [unwired: 2 out]
    n294 = Equal?(x=w674, y=inf) -> (x = y?=w673:bool)
    n295 = feedback #12() -> (w672:T2)  [unwired: 1 in]
    n296 = Select(t=w672, s=w673, f=w671) -> (s? t:f=w670:T2)
    "Tuned PID gains 4" <- w670
    n297 = feedback-in #12(w670) -> ()
    n298 = case shown="True" "Accept gain 4" {
      tunnel: w670 -> [_ w717]
      frame False {
      }
      frame True {
        n299 = local write "PID Gains 4"(w717) -> ()
      }
    }
    n300 = local read "Stop 4"() -> (w679:bool)
  }
  n301 = while {
    tunnel: w94 -> [_]
    tunnel: w90 -> [w721]
    stop <- w731 stop-if-true
    # "If dT and deadtime have similar values, the identification could evaluate deadtime as zero and this generates proportional gain equal to Inf. This code avoid gain changes in this situations."
    # "Autotuning Loop"
    n302 = local read "Control Output 3"() -> (w733:dbl[])
    n303 = local read "Measurement 3"() -> (w732:dbl[])
    n304 = case shown="\"Chien-Hrones-Reswick\"" "Control 3" {
      tunnel: w733 -> [w742 w750 w759 w768]
      tunnel: w732 -> [w741 w749 w758 w767]
      tunnel: [w740 w748 w757 w766] -> w720
      tunnel: [w739 w747 w756 w765] -> w719
      tunnel: w721 -> [w738 w746 w755 w764]
      tunnel: [w737 w745 w754 w763] -> w718
      tunnel: [w736 w744 w753 w762] -> w723
      tunnel: "Type of controller 3" -> [w735 w743 w752 w761]
      frame "Ziegler-Nichols", Default {
        n305 = call-poly <vilib>:"PID Autotuning Design.vi"("Ziegler-Nichols Speed"="Ziegler-Nichols speed 3", "Type of Controller"=w735, "dt (s)"=w738, "Response signal"=w741, "Stimulus signal"=w742) -> ("PID gains"=w736:T2, "response operating point"=w739:dbl, "stimulus operating point"=w740:dbl, "Plant Parameters"=w737:T4)  [unwired: 3 in]
      }
      frame "Cohen-Coon" {
        n306 = call-poly <vilib>:"PID Autotuning Design.vi"("Type of Controller"=w743, "dt (s)"=w746, "Response signal"=w749, "Stimulus signal"=w750) -> ("PID gains"=w744:T2, "response offset"=w747:dbl, "stimulus offset"=w748:dbl, "Plant Parameters"=w745:T4)  [unwired: 4 in]
      }
      frame "Chien-Hrones-Reswick" {
        n307 = call-poly <vilib>:"PID Autotuning Design.vi"("Tuning specifications"="Tuning specifications 3", "Type of Controller"=w752, "dt (s)"=w755, "Response signal"=w758, "Stimulus signal"=w759) -> ("PID gains"=w753:T2, "response offset"=w756:dbl, "stimulus offset"=w757:dbl, "Plant Parameters"=w754:T4)  [unwired: 3 in]
      }
      frame "Internal Model Control" {
        n308 = call-poly <vilib>:"PID Autotuning Design.vi"("Desired Time Constant (tau_c)"="Multiplicative factor 3", "Type of Controller"=w761, "dt (s)"=w764, "Response signal"=w767, "Stimulus signal"=w768) -> ("PID gains"=w762:T2, "response offset"=w765:dbl, "stimulus offset"=w766:dbl, "Plant Parameters"=w763:T4)  [unwired: 3 in]
      }
    }
    "Stimulus operating point 3" <- w720
    "Response operating point 3" <- w719
    "Identified Plant Parameters 3" <- w718
    n309 = Unbundle(w723) -> ("proportional gain (Kc)"=w726:dbl)  [unwired: 2 out]
    n310 = Equal?(x=w726, y=inf) -> (x = y?=w725:bool)
    n311 = feedback #13() -> (w724:T2)  [unwired: 1 in]
    n312 = Select(t=w724, s=w725, f=w723) -> (s? t:f=w722:T2)
    "Tuned PID gains 3" <- w722
    n313 = feedback-in #13(w722) -> ()
    n314 = case shown="True" "Accept gain 3" {
      tunnel: w722 -> [_ w769]
      frame False {
      }
      frame True {
        n315 = local write "PID Gains 3"(w769) -> ()
      }
    }
    n316 = local read "Stop 3"() -> (w731:bool)
  }
  n317 = while {
    tunnel: w82 -> [_]
    tunnel: w78 -> [w773]
    stop <- w783 stop-if-true
    # "If dT and deadtime have similar values, the identification could evaluate deadtime as zero and this generates proportional gain equal to Inf. This code avoid gain changes in this situations."
    # "Autotuning Loop"
    n318 = local read "Control Output 5"() -> (w785:dbl[])
    n319 = local read "Measurement 5"() -> (w784:dbl[])
    n320 = case shown="\"Chien-Hrones-Reswick\"" "Control 5" {
      tunnel: w785 -> [w794 w802 w811 w820]
      tunnel: w784 -> [w793 w801 w810 w819]
      tunnel: [w792 w800 w809 w818] -> w772
      tunnel: [w791 w799 w808 w817] -> w771
      tunnel: w773 -> [w790 w798 w807 w816]
      tunnel: [w789 w797 w806 w815] -> w770
      tunnel: [w788 w796 w805 w814] -> w775
      tunnel: "Type of controller 5" -> [w787 w795 w804 w813]
      frame "Ziegler-Nichols", Default {
        n321 = call-poly <vilib>:"PID Autotuning Design.vi"("Ziegler-Nichols Speed"="Ziegler-Nichols speed 5", "Type of Controller"=w787, "dt (s)"=w790, "Response signal"=w793, "Stimulus signal"=w794) -> ("PID gains"=w788:T2, "response operating point"=w791:dbl, "stimulus operating point"=w792:dbl, "Plant Parameters"=w789:T4)  [unwired: 3 in]
      }
      frame "Cohen-Coon" {
        n322 = call-poly <vilib>:"PID Autotuning Design.vi"("Type of Controller"=w795, "dt (s)"=w798, "Response signal"=w801, "Stimulus signal"=w802) -> ("PID gains"=w796:T2, "response offset"=w799:dbl, "stimulus offset"=w800:dbl, "Plant Parameters"=w797:T4)  [unwired: 4 in]
      }
      frame "Chien-Hrones-Reswick" {
        n323 = call-poly <vilib>:"PID Autotuning Design.vi"("Tuning specifications"="Tuning specifications 5", "Type of Controller"=w804, "dt (s)"=w807, "Response signal"=w810, "Stimulus signal"=w811) -> ("PID gains"=w805:T2, "response offset"=w808:dbl, "stimulus offset"=w809:dbl, "Plant Parameters"=w806:T4)  [unwired: 3 in]
      }
      frame "Internal Model Control" {
        n324 = call-poly <vilib>:"PID Autotuning Design.vi"("Desired Time Constant (tau_c)"="Multiplicative factor 5", "Type of Controller"=w813, "dt (s)"=w816, "Response signal"=w819, "Stimulus signal"=w820) -> ("PID gains"=w814:T2, "response offset"=w817:dbl, "stimulus offset"=w818:dbl, "Plant Parameters"=w815:T4)  [unwired: 3 in]
      }
    }
    "Stimulus operating point 5" <- w772
    "Response operating point 5" <- w771
    "Identified Plant Parameters 5" <- w770
    n325 = Unbundle(w775) -> ("proportional gain (Kc)"=w778:dbl)  [unwired: 2 out]
    n326 = Equal?(x=w778, y=inf) -> (x = y?=w777:bool)
    n327 = feedback #14() -> (w776:T2)  [unwired: 1 in]
    n328 = Select(t=w776, s=w777, f=w775) -> (s? t:f=w774:T2)
    "Tuned PID gains 5" <- w774
    n329 = feedback-in #14(w774) -> ()
    n330 = case shown="True" "Accept gain 5" {
      tunnel: w774 -> [_ w821]
      frame False {
      }
      frame True {
        n331 = local write "PID Gains 5"(w821) -> ()
      }
    }
    n332 = local read "Stop 5"() -> (w783:bool)
  }
  n333 = while {
    tunnel: w100 -> [_]
    tunnel: w96 -> [w825]
    stop <- w835 stop-if-true
    # "If dT and deadtime have similar values, the identification could evaluate deadtime as zero and this generates proportional gain equal to Inf. This code avoid gain changes in this situations."
    # "Autotuning Loop"
    n334 = local read "Control Output 2"() -> (w837:dbl[])
    n335 = local read "Measurement 2"() -> (w836:dbl[])
    n336 = case shown="\"Chien-Hrones-Reswick\"" "Control 2" {
      tunnel: w837 -> [w846 w854 w863 w872]
      tunnel: w836 -> [w845 w853 w862 w871]
      tunnel: [w844 w852 w861 w870] -> w824
      tunnel: [w843 w851 w860 w869] -> w823
      tunnel: w825 -> [w842 w850 w859 w868]
      tunnel: [w841 w849 w858 w867] -> w822
      tunnel: [w840 w848 w857 w866] -> w827
      tunnel: "Type of controller 2" -> [w839 w847 w856 w865]
      frame "Ziegler-Nichols", Default {
        n337 = call-poly <vilib>:"PID Autotuning Design.vi"("Ziegler-Nichols Speed"="Ziegler-Nichols speed 2", "Type of Controller"=w839, "dt (s)"=w842, "Response signal"=w845, "Stimulus signal"=w846) -> ("PID gains"=w840:T2, "response operating point"=w843:dbl, "stimulus operating point"=w844:dbl, "Plant Parameters"=w841:T4)  [unwired: 3 in]
      }
      frame "Cohen-Coon" {
        n338 = call-poly <vilib>:"PID Autotuning Design.vi"("Type of Controller"=w847, "dt (s)"=w850, "Response signal"=w853, "Stimulus signal"=w854) -> ("PID gains"=w848:T2, "response offset"=w851:dbl, "stimulus offset"=w852:dbl, "Plant Parameters"=w849:T4)  [unwired: 4 in]
      }
      frame "Chien-Hrones-Reswick" {
        n339 = call-poly <vilib>:"PID Autotuning Design.vi"("Tuning specifications"="Tuning specifications 2", "Type of Controller"=w856, "dt (s)"=w859, "Response signal"=w862, "Stimulus signal"=w863) -> ("PID gains"=w857:T2, "response offset"=w860:dbl, "stimulus offset"=w861:dbl, "Plant Parameters"=w858:T4)  [unwired: 3 in]
      }
      frame "Internal Model Control" {
        n340 = call-poly <vilib>:"PID Autotuning Design.vi"("Desired Time Constant (tau_c)"="Multiplicative factor 2", "Type of Controller"=w865, "dt (s)"=w868, "Response signal"=w871, "Stimulus signal"=w872) -> ("PID gains"=w866:T2, "response offset"=w869:dbl, "stimulus offset"=w870:dbl, "Plant Parameters"=w867:T4)  [unwired: 3 in]
      }
    }
    "Stimulus operating point 2" <- w824
    "Response operating point 2" <- w823
    "Identified Plant Parameters 2" <- w822
    n341 = Unbundle(w827) -> ("proportional gain (Kc)"=w830:dbl)  [unwired: 2 out]
    n342 = Equal?(x=w830, y=inf) -> (x = y?=w829:bool)
    n343 = feedback #15() -> (w828:T2)  [unwired: 1 in]
    n344 = Select(t=w828, s=w829, f=w827) -> (s? t:f=w826:T2)
    "Tuned PID gains 2" <- w826
    n345 = feedback-in #15(w826) -> ()
    n346 = case shown="True" "Accept gain 2" {
      tunnel: w826 -> [_ w873]
      frame False {
      }
      frame True {
        n347 = local write "PID Gains 2"(w873) -> ()
      }
    }
    n348 = local read "Stop 2"() -> (w835:bool)
  }
  n349 = while {
    shift-right: [w881] -> w134
    shift-left: w133 -> [w877]
    tunnel: w132 -> [w876]
    tunnel: [w878] -> w135
    stop <- w879 stop-if-true
    # "Serial Read Loop"
    n350 = case shown="True" TRUE {
      tunnel: [w893 w897] -> w881
      tunnel: w877 -> [w895 w897]
      tunnel: [w892 w896] -> w878
      tunnel: w876 -> [w894 w896]
      frame True {
        n351 = VISA Read(VISA resource name=w895, byte count=u32 1000, error in (no error)=w894) -> (VISA resource name out=w893:refnum<visa-resource-name>, read buffer=w890:string, error out=w892:errorcluster)  [unwired: 1 out]
        n352 = Decimal String To Number(string=w890) -> (number=w888:i32)  [unwired: 2 in, 1 out]
        "Sensor Raw Value" <- w888
        n353 = call <vilib>:"Median PtByPt.vi"("sample length"=20, "x"=w888) -> ("median"=w886:dbl)  [unwired: 2 in, 1 out]
        n354 = To Double Precision Float(number=w886) -> (double precision float=w882:dbl)
        n355 = Multiply(x=w882, y=0.0292) -> (x*y=w885:dbl)
        "Force in Kilograms 2" <- w885
        n356 = Multiply(x=w885, y=9.81) -> (x*y=→"Force in Newtons 2":dbl)
      }
      frame False {
      }
    }
    n357 = Wait (ms)(milliseconds to wait=u32 5) -> ()  [unwired: 1 out]
    n358 = Or(x=w878, y=FALSE) -> (x .or. y?=w879:bool)
  }
  n359 = while {
    shift-right: [w905] -> w102
    shift-left: w128 -> [w901]
    tunnel: w127 -> [w900]
    tunnel: [w902] -> w129
    stop <- w903 stop-if-true
    # "Serial Read Loop"
    n360 = case shown="True" TRUE {
      tunnel: [w917 w921] -> w905
      tunnel: w901 -> [w919 w921]
      tunnel: [w916 w920] -> w902
      tunnel: w900 -> [w918 w920]
      frame True {
        n361 = VISA Read(VISA resource name=w919, byte count=u32 1000, error in (no error)=w918) -> (VISA resource name out=w917:refnum<visa-resource-name>, read buffer=w914:string, error out=w916:errorcluster)  [unwired: 1 out]
        n362 = Decimal String To Number(string=w914) -> (number=w910:i32)  [unwired: 2 in, 1 out]
        "Sensor Raw Value 2" <- w910
        n363 = call <vilib>:"Median PtByPt.vi"("sample length"=20, "x"=w910) -> ("median"=w911:dbl)  [unwired: 2 in, 1 out]
        n364 = To Double Precision Float(number=w911) -> (double precision float=w907:dbl)
        n365 = Multiply(x=w907, y=0.0238) -> (x*y=w906:dbl)
        "Force in Kilograms" <- w906
        n366 = Multiply(x=w906, y=9.81) -> (x*y=→"Force in Newtons":dbl)
      }
      frame False {
      }
    }
    n367 = Or(x=w902, y=FALSE) -> (x .or. y?=w903:bool)
    n368 = Wait (ms)(milliseconds to wait=u32 5) -> ()  [unwired: 1 out]
  }
  n369 = VISA Close(VISA resource name=w134, error in (no error)=w135) -> (error out=w136:errorcluster)
  n370 = call <vilib>:"Simple Error Handler.vi"("error in (no error)"=w136) -> ()  [unwired: 1 in, 8 out]
  n371 = VISA Close(VISA resource name=w102, error in (no error)=w129) -> (error out=w130:errorcluster)
  n372 = call <vilib>:"Simple Error Handler.vi"("error in (no error)"=w130) -> ()  [unwired: 1 in, 8 out]
  n373 = stacked-sequence {
    tunnel: [_ w927] -> w109
    tunnel: [_ w926] -> w108
    frame #0 {
      w922 = 0
      w923 = FALSE
      w924 = ""
      # "Initialize Indicators"
      "Connected" <- w923
      "Start Time Text" <- w924
      "Stop Time Text" <- w924
      "Elapsed Time Text" <- w924
      "HostFrameCount" <- w922
      "Running" <- w923
      "Loop Iter" <- w922
      "PnoData" <- w923
    }
    frame #1 {
      # "Connect To Tracker"
      # "2. Initialize Tracker Connection"
      n374 = call <instrlib>:"PDI initialize.vi"() -> ("error out"=w926:errorcluster, "Connected"=w925:bool, "pDev"=w927:u32)  [unwired: 1 in, 4 out]
      n375 = local write "Connected"(w925) -> ()
    }
  }
  n376 = while {
    stop <- FALSE stop-if-true
    # "TRACKER 4"
    # "TRACKER 3"
    # "TRACKER 2"
    # "TRACKER 1"
    n377 = Index Array(array="XYZAER", index #1=0 ("index"), index #2=1 ("index"), index #3=2 ("index"), index #4=3 ("index")) -> (element #1=w952:T8, element #2=w951:T8, element #3=w950:T8, element #4=w949:T8)
    n378 = Unbundle By Name(w952) -> ("x"=w939:sgl, "y"=w938:sgl)  [unwired: 1 out]
    n379 = Unbundle By Name(w951) -> ("x"=w936:sgl, "y"=w935:sgl)  [unwired: 1 out]
    n380 = Multiply(x=w938, y=sgl -1.0) -> (x*y=w937:sgl)
    n381 = Multiply(x=w935, y=-1.0) -> (x*y=w934:dbl)
    n382 = Bundle(w934, "x"=w936) -> (w947:cluster{dbl, "x":sgl})  [unwired: 1 in]
    n383 = Bundle(w937, "x"=w939) -> (w948:cluster{sgl, "x":sgl})  [unwired: 1 in]
    n384 = Unbundle By Name(w950) -> ("x"=w933:sgl, "y"=w932:sgl)  [unwired: 1 out]
    n385 = Unbundle By Name(w949) -> ("x"=w930:sgl, "y"=w929:sgl)  [unwired: 1 out]
    n386 = Multiply(x=w932, y=-1.0) -> (x*y=w931:dbl)
    n387 = Multiply(x=w929, y=-1.0) -> (x*y=w928:dbl)
    n388 = Bundle(w931, "x"=w933) -> (w946:cluster{dbl, "x":sgl})  [unwired: 1 in]
    n389 = Bundle(w928, "x"=w930) -> (w945:cluster{dbl, "x":sgl})  [unwired: 1 in]
    n390 = Build Array(w948, w947, w946, w945) -> (→"Position Sensor Data":cluster{dbl, "x":sgl}[])
  }
  n391 = call <instrlib>:"PDI util stationcount.vi"("error in (no error)"=w108, "pDev"=w109) -> ("error out"=w107:errorcluster, "dup pDev"=w106:u32, "MaxCount"=w104:i32)  [unwired: 7 out]
  n392 = call <instrlib>:"PDI config setbuffer.vi"("error in (no error)"=w107, "Max sensors"=w104, "FrameCount"=w105, "pDev"=w106) -> ("error out"=w116:errorcluster, "dup pDev"=w117:u32)  [unwired: 6 out]
  n393 = flat-sequence {
    tunnel: w122 -> [_]
    tunnel: [w959] -> w118
    frame #0 {
      # "Get Start Time"
      n394 = Get Date/Time In Seconds() -> (seconds since 1Jan1904=w960:timestamp)
      n395 = Format Date/Time String(seconds (now)=w960) -> (date/time string=w961:string)  [unwired: 2 out]
      n396 = local write "Start Time Text"(w961) -> ()
      n397 = To Double Precision Float(number=w960) -> (double precision float=w959:dbl)
    }
  }
  n398 = call <instrlib>:"PDI action startcont.vi"("error in (no error)"=w116, "pDev"=w117) -> ("error out"=w123:errorcluster, "Running"=w115:bool, "dup pDev"=w122:u32)  [unwired: 7 out]
  n399 = control-ref of="HostFrameCount"() -> (w113:refnum<vi>)
  n400 = local write "Running"(w115) -> ()
  n401 = Obtain Queue(element data type=0.0) -> (queue out=w5:refnum<queue>)  [unwired: 4 in, 2 out]
  n402 = while {
    shift-left: 0.0 ("Plant Output") -> [w1028]
    shift-right: [w1023] -> _
    tunnel: w58 -> [_]
    shift-right: [w1009] -> _
    shift-left: 0.01 -> [w1007]
    shift-right: [w981] -> _
    shift-left: TRUE -> [w1006]
    shift-right: [w983] -> _
    shift-left: w55 -> [w1005]
    shift-right: [w1008] -> _
    shift-left: w55 -> [w1004]
    tunnel: [w978] -> w54
    tunnel: [w964] -> w25
    tunnel: w5 -> [w962]
    stop <- "Stop 9" stop-if-true
    w969 = 1 items=["one channel for each line", "one channel for all lines"] ("line grouping")
    w978 = 0.05 ("Sampling Time dt (s)")
    w987 = 1 items=["one channel for each line", "one channel for all lines"] ("line grouping")
    w995 = 0.5 ("x")
    w1022 = T7 {"static gain"=2.5, "lag (s)"=2.5, "deadtime (s)"=0.01, "load"=0.0, "deadband"=0.0, "sensor noise"=0.0, "initial PV"=30.0, "plant noise"=0.0}  # Process parameters
    w1024 = FALSE  # Integrator ?
    # "C."
    # "Inlet 11"
    # "Exhaust 4"
    # "B."
    # "A."
    # "A.Output to PWM Logic \nB. Simulated Plant\nC. Draw Chart"
    # "Main PID Loop Control"
    n403 = Dequeue Element(queue=w962) -> (element=w963:dbl)  [unwired: 2 in, 3 out]
    n404 = Multiply(x=w978, y=1000.0) -> (x*y=w1021:dbl)
    n405 = Not(x="Autotune 9") -> (.not. x?=w1025:bool)
    n406 = feedback #16() -> (w1030:bool)  [unwired: 1 in]
    n407 = feedback-in #16("Autotune 9") -> ()
    n408 = Wait Until Next ms Multiple(millisecond multiple=w1021) -> ()  [unwired: 1 out]
    n409 = Exclusive Or(1:w1030, 2:"Autotune 9") -> (0:w1029:bool)
    n410 = feedback #17() -> (w1027:dbl)  [unwired: 1 in]
    n411 = Multiply(x=w963, y=-1000.0) -> (x*y=w1011:dbl)
    n412 = call <vilib>:"Median PtByPt.vi"("sample length"="Median sample length 18", "x"=w1011) -> ("median"=w1010:dbl)  [unwired: 2 in, 1 out]
    n413 = Square(x=w1010) -> (x^2=w1018:dbl)
    n414 = Multiply(x=w1010, y=0.1121) -> (x*y=w1014:dbl)
    n415 = Multiply(x=w1018, y=0.0243) -> (x*y=w1015:dbl)
    n416 = Add(x=w1014, y=w1015) -> (x+y=w1013:dbl)
    n417 = Add(x=-235.77, y=w1013) -> (x+y=w976:dbl)
    n418 = case shown="False" "Autotune 9" {
      tunnel: w978 -> [w1045 _]
      tunnel: [w1034 w1050] -> w983
      tunnel: w1028 -> [_ w1049]
      tunnel: "PID Gains 9" -> [w1044 _]
      tunnel: "Reinitialize 9" -> [w1041 _]
      tunnel: w1029 -> [w1043 w1048]
      tunnel: w1027 -> [_ w1052]
      tunnel: w976 -> [w1037 _]
      tunnel: "Set Point 9" -> [w1036 _]
      frame False {
        # "This code is to have 'bumpless' transfer from autotuning"
        n419 = Not(x=w1043) -> (.not. x?=w1040:bool)
        n420 = And(x="Automatic 9", y=w1040) -> (x .and. y?=w1042:bool)
        n421 = call-poly <vilib>:"PID Advanced.vi"("setpoint"=w1036, "auto? (T)"=w1042, "manual control"="MV: 9", "process variable"=w1037, "alpha"=10.0, "PID gains"=w1044, "dt (s)"=w1045, "reinitialize? (F)"=w1041) -> ("output"=w1034:dbl)  [unwired: 6 in, 1 out]
      }
      frame True {
        w1055 = 10000 ("sample length")
        # "Buffering data for parameters estimation"
        n422 = call <vilib>:"Data Queue PtByPt.vi"("initial queue element"=w1049, "initialize"=w1048, "sample length"=w1055, "input data point"=w1049) -> ("Current Queue"=→"Control Output 9":dbl[])  [unwired: 3 in, 4 out]
        n423 = Select(t=0.0, s=w1048, f="Excitation 9") -> (s? t:f=w1053:dbl)
        n424 = Add(x=w1052, y=w1053) -> (x+y=w1050:dbl)
        n425 = call <vilib>:"Data Queue PtByPt.vi"("initial queue element"=w1050, "initialize"=w1048, "sample length"=w1055, "input data point"=w1050) -> ("Current Queue"=→"Measurement 9":dbl[])  [unwired: 3 in, 4 out]
      }
    }
    n426 = feedback-in #17(w983, w1025) -> ()
    n427 = Greater?(x=w976, y="M-4") -> (0:w964:bool)
    n428 = Add(x=w1007, y=w995) -> (x+y=w996:dbl)
    n429 = Subtract(x=w1007, y=w995) -> (x-y=w994:dbl)
    n430 = Equal?(x=w1005, y=w983) -> (x = y?=w1002:bool)
    n431 = Greater?(x=w983, y=w1005) -> (0:w1001:bool)
    n432 = Select(t=w1006, s=w1002, f=w1001) -> (s? t:f=w981:bool)
    "PWM Output 9" <- w981
    n433 = call "Plant System.vi"("Integrator ?"=w1024, "Plant Input"=w983, "dt (s)"=w978, "process parameters"=w1022) -> ("Plant Output"=w1023:dbl)  [unwired: 11 in]
    n434 = Increment(x="Set Point 9") -> (x+1=w1000:dbl)
    n435 = Decrement(x="Set Point 9") -> (x-1=w999:dbl)
    n436 = Select(t=w996, s=w981, f=w994) -> (s? t:f=w1009:dbl)
    n437 = Select(t=w1000, s=w981, f=w999) -> (s? t:f=w998:dbl)
    n438 = Not(x=w981) -> (.not. x?=w980:bool)
    n439 = call-poly <vilib>:"DAQmx Create Virtual Channel.vi"("lines"=tag "cDAQ1Mod8/port0/line5", "line grouping"=w987) -> ("task out"=w989:refnum<k21>, "error out"=w988:errorcluster)  [unwired: 12 in]
    n440 = call-poly <vilib>:"DAQmx Create Virtual Channel.vi"("lines"=tag "cDAQ1Mod7/port0/line4", "line grouping"=w969) -> ("task out"=w971:refnum<k21>, "error out"=w970:errorcluster)  [unwired: 12 in]
    n441 = Build Array(w976, "Set Point 9", w998) -> (w997:dbl[])
    n442 = Initialize Array("INLET 10 ON/OFF 2", 1 ("dimension size")) -> (w966:bool[])
    n443 = Initialize Array(w980, 1 ("dimension size")) -> (w984:bool[])
    n444 = local write "MV: 9"(w983) -> ()
    n445 = Add(x=w1004, y=w1007) -> (x+y=w1008:dbl)
    n446 = Build Array(w997) -> (→"Real time Data 9":dbl[][])
    n447 = call-poly <vilib>:"DAQmx Write.vi"("task/channels in"=w989, "auto start"=TRUE, "data"=w984, "error in"=w988) -> ("task out"=w991:refnum<k21>, "error out"=w992:errorcluster)  [unwired: 9 in, 1 out]
    n448 = call-poly <vilib>:"DAQmx Write.vi"("task/channels in"=w971, "auto start"=TRUE, "data"=w966, "error in"=w970) -> ("task out"=w973:refnum<k21>, "error out"=w974:errorcluster)  [unwired: 9 in, 1 out]
    n449 = call <vilib>:"DAQmx Clear Task.vi"("task in"=w991, "error in"=w992) -> ("error out"=w986:errorcluster)  [unwired: 13 in]
    n450 = call <vilib>:"DAQmx Clear Task.vi"("task in"=w973, "error in"=w974) -> ("error out"=w968:errorcluster)  [unwired: 13 in]
    n451 = call <vilib>:"Simple Error Handler.vi"("error in (no error)"=w986) -> ()  [unwired: 4 in, 5 out]
    n452 = call <vilib>:"Simple Error Handler.vi"("error in (no error)"=w968) -> ()  [unwired: 4 in, 5 out]
  }
  n453 = control-ref of="stop"() -> (w121:refnum<vi>)
  n454 = control-ref of="XYZAER"() -> (w112:refnum<vi>)
  n455 = Obtain Queue(element data type=0.0) -> (queue out=w2:refnum<queue>)  [unwired: 4 in, 2 out]
  n456 = while {
    shift-left: 0.0 ("Plant Output") -> [w1122]
    shift-right: [w1117] -> _
    tunnel: w64 -> [_]
    shift-right: [w1103] -> _
    shift-left: 0.01 -> [w1101]
    shift-right: [w1075] -> _
    shift-left: TRUE -> [w1100]
    shift-right: [w1077] -> _
    shift-left: w61 -> [w1099]
    shift-right: [w1102] -> _
    shift-left: w61 -> [w1098]
    tunnel: [w1072] -> w60
    tunnel: [w1058] -> w24
    tunnel: w2 -> [w1056]
    stop <- "Stop 8" stop-if-true
    w1063 = 1 items=["one channel for each line", "one channel for all lines"] ("line grouping")
    w1072 = 0.05 ("Sampling Time dt (s)")
    w1081 = 1 items=["one channel for each line", "one channel for all lines"] ("line grouping")
    w1089 = 0.5 ("x")
    w1116 = T7 {"static gain"=2.5, "lag (s)"=2.5, "deadtime (s)"=0.01, "load"=0.0, "deadband"=0.0, "sensor noise"=0.0, "initial PV"=30.0, "plant noise"=0.0}  # Process parameters
    w1118 = FALSE  # Integrator ?
    # "C."
    # "Inlet 11"
    # "Exhaust 2"
    # "B."
    # "A."
    # "A.Output to PWM Logic \nB. Simulated Plant\nC. Draw Chart"
    # "Main PID Loop Control"
    n457 = Dequeue Element(queue=w1056) -> (element=w1057:dbl)  [unwired: 2 in, 3 out]
    n458 = Multiply(x=w1072, y=1000.0) -> (x*y=w1115:dbl)
    n459 = Not(x="Autotune 8") -> (.not. x?=w1119:bool)
    n460 = feedback #18() -> (w1124:bool)  [unwired: 1 in]
    n461 = feedback-in #18("Autotune 8") -> ()
    n462 = Wait Until Next ms Multiple(millisecond multiple=w1115) -> ()  [unwired: 1 out]
    n463 = Exclusive Or(1:w1124, 2:"Autotune 8") -> (0:w1123:bool)
    n464 = feedback #19() -> (w1121:dbl)  [unwired: 1 in]
    n465 = Multiply(x=w1057, y=-1000.0) -> (x*y=w1105:dbl)
    n466 = call <vilib>:"Median PtByPt.vi"("sample length"="Median sample length 17", "x"=w1105) -> ("median"=w1104:dbl)  [unwired: 2 in, 1 out]
    n467 = Square(x=w1104) -> (x^2=w1112:dbl)
    n468 = Multiply(x=w1104, y=-7.5945) -> (x*y=w1108:dbl)
    n469 = Multiply(x=w1112, y=0.0612) -> (x*y=w1109:dbl)
    n470 = Add(x=w1108, y=w1109) -> (x+y=w1107:dbl)
    n471 = Add(x=143.72, y=w1107) -> (x+y=w1070:dbl)
    n472 = case shown="False" "Autotune 8" {
      tunnel: w1072 -> [w1139 _]
      tunnel: [w1128 w1144] -> w1077
      tunnel: w1122 -> [_ w1143]
      tunnel: "PID Gains 8" -> [w1138 _]
      tunnel: "Reinitialize 8" -> [w1135 _]
      tunnel: w1123 -> [w1137 w1142]
      tunnel: w1121 -> [_ w1146]
      tunnel: w1070 -> [w1131 _]
      tunnel: "Set Point 8" -> [w1130 _]
      frame False {
        # "This code is to have 'bumpless' transfer from autotuning"
        n473 = Not(x=w1137) -> (.not. x?=w1134:bool)
        n474 = And(x="Automatic 8", y=w1134) -> (x .and. y?=w1136:bool)
        n475 = call-poly <vilib>:"PID Advanced.vi"("setpoint"=w1130, "auto? (T)"=w1136, "manual control"="MV: 8", "process variable"=w1131, "alpha"=10.0, "PID gains"=w1138, "dt (s)"=w1139, "reinitialize? (F)"=w1135) -> ("output"=w1128:dbl)  [unwired: 6 in, 1 out]
      }
      frame True {
        w1149 = 10000 ("sample length")
        # "Buffering data for parameters estimation"
        n476 = call <vilib>:"Data Queue PtByPt.vi"("initial queue element"=w1143, "initialize"=w1142, "sample length"=w1149, "input data point"=w1143) -> ("Current Queue"=→"Control Output 8":dbl[])  [unwired: 3 in, 4 out]
        n477 = Select(t=0.0, s=w1142, f="Excitation 8") -> (s? t:f=w1147:dbl)
        n478 = Add(x=w1146, y=w1147) -> (x+y=w1144:dbl)
        n479 = call <vilib>:"Data Queue PtByPt.vi"("initial queue element"=w1144, "initialize"=w1142, "sample length"=w1149, "input data point"=w1144) -> ("Current Queue"=→"Measurement 8":dbl[])  [unwired: 3 in, 4 out]
      }
    }
    n480 = feedback-in #19(w1077, w1119) -> ()
    n481 = Greater?(x=w1070, y="M-2") -> (0:w1058:bool)
    n482 = Add(x=w1101, y=w1089) -> (x+y=w1090:dbl)
    n483 = Subtract(x=w1101, y=w1089) -> (x-y=w1088:dbl)
    n484 = Equal?(x=w1099, y=w1077) -> (x = y?=w1096:bool)
    n485 = Greater?(x=w1077, y=w1099) -> (0:w1095:bool)
    n486 = Select(t=w1100, s=w1096, f=w1095) -> (s? t:f=w1075:bool)
    "PWM Output 8" <- w1075
    n487 = call "Plant System.vi"("Integrator ?"=w1118, "Plant Input"=w1077, "dt (s)"=w1072, "process parameters"=w1116) -> ("Plant Output"=w1117:dbl)  [unwired: 11 in]
    n488 = Increment(x="Set Point 8") -> (x+1=w1094:dbl)
    n489 = Decrement(x="Set Point 8") -> (x-1=w1093:dbl)
    n490 = Select(t=w1090, s=w1075, f=w1088) -> (s? t:f=w1103:dbl)
    n491 = Select(t=w1094, s=w1075, f=w1093) -> (s? t:f=w1092:dbl)
    n492 = Not(x=w1075) -> (.not. x?=w1074:bool)
    n493 = call-poly <vilib>:"DAQmx Create Virtual Channel.vi"("lines"=tag "cDAQ1Mod1/port0/line6", "line grouping"=w1081) -> ("task out"=w1083:refnum<k21>, "error out"=w1082:errorcluster)  [unwired: 12 in]
    n494 = call-poly <vilib>:"DAQmx Create Virtual Channel.vi"("lines"=tag "cDAQ1Mod2/port0/line6", "line grouping"=w1063) -> ("task out"=w1065:refnum<k21>, "error out"=w1064:errorcluster)  [unwired: 12 in]
    n495 = Build Array(w1070, "Set Point 8", w1092) -> (w1091:dbl[])
    n496 = Initialize Array("INLET 2 ON/OFF 2", 1 ("dimension size")) -> (w1060:bool[])
    n497 = Initialize Array(w1074, 1 ("dimension size")) -> (w1078:bool[])
    n498 = local write "MV: 8"(w1077) -> ()
    n499 = Add(x=w1098, y=w1101) -> (x+y=w1102:dbl)
    n500 = Build Array(w1091) -> (→"Real time Data 8":dbl[][])
    n501 = call-poly <vilib>:"DAQmx Write.vi"("task/channels in"=w1083, "auto start"=TRUE, "data"=w1078, "error in"=w1082) -> ("task out"=w1085:refnum<k21>, "error out"=w1086:errorcluster)  [unwired: 9 in, 1 out]
    n502 = call-poly <vilib>:"DAQmx Write.vi"("task/channels in"=w1065, "auto start"=TRUE, "data"=w1060, "error in"=w1064) -> ("task out"=w1067:refnum<k21>, "error out"=w1068:errorcluster)  [unwired: 9 in, 1 out]
    n503 = call <vilib>:"DAQmx Clear Task.vi"("task in"=w1085, "error in"=w1086) -> ("error out"=w1080:errorcluster)  [unwired: 13 in]
    n504 = call <vilib>:"DAQmx Clear Task.vi"("task in"=w1067, "error in"=w1068) -> ("error out"=w1062:errorcluster)  [unwired: 13 in]
    n505 = call <vilib>:"Simple Error Handler.vi"("error in (no error)"=w1080) -> ()  [unwired: 4 in, 5 out]
    n506 = call <vilib>:"Simple Error Handler.vi"("error in (no error)"=w1062) -> ()  [unwired: 4 in, 5 out]
  }
  n507 = Obtain Queue(element data type=0.0) -> (queue out=w10:refnum<queue>)  [unwired: 4 in, 2 out]
  n508 = while {
    shift-left: 0.0 ("Plant Output") -> [w1216]
    shift-right: [w1211] -> _
    tunnel: w46 -> [_]
    shift-right: [w1197] -> _
    shift-left: 0.01 -> [w1195]
    shift-right: [w1169] -> _
    shift-left: TRUE -> [w1194]
    shift-right: [w1171] -> _
    shift-left: w43 -> [w1193]
    shift-right: [w1196] -> _
    shift-left: w43 -> [w1192]
    tunnel: [w1166] -> w42
    tunnel: [w1152] -> w27
    tunnel: w10 -> [w1150]
    stop <- "Stop 11" stop-if-true
    w1157 = 1 items=["one channel for each line", "one channel for all lines"] ("line grouping")
    w1166 = 0.05 ("Sampling Time dt (s)")
    w1175 = 1 items=["one channel for each line", "one channel for all lines"] ("line grouping")
    w1183 = 0.5 ("x")
    w1210 = T7 {"static gain"=2.5, "lag (s)"=2.5, "deadtime (s)"=0.01, "load"=0.0, "deadband"=0.0, "sensor noise"=0.0, "initial PV"=30.0, "plant noise"=0.0}  # Process parameters
    w1212 = FALSE  # Integrator ?
    # "C."
    # "Inlet 11"
    # "Exhaust 5"
    # "B."
    # "A."
    # "A.Output to PWM Logic \nB. Simulated Plant\nC. Draw Chart"
    # "Main PID Loop Control"
    n509 = Dequeue Element(queue=w1150) -> (element=w1151:dbl)  [unwired: 2 in, 3 out]
    n510 = Multiply(x=w1166, y=1000.0) -> (x*y=w1209:dbl)
    n511 = Not(x="Autotune 11") -> (.not. x?=w1213:bool)
    n512 = feedback #20() -> (w1218:bool)  [unwired: 1 in]
    n513 = feedback-in #20("Autotune 11") -> ()
    n514 = Wait Until Next ms Multiple(millisecond multiple=w1209) -> ()  [unwired: 1 out]
    n515 = Exclusive Or(1:w1218, 2:"Autotune 11") -> (0:w1217:bool)
    n516 = feedback #21() -> (w1215:dbl)  [unwired: 1 in]
    n517 = Multiply(x=w1151, y=-1000.0) -> (x*y=w1199:dbl)
    n518 = call <vilib>:"Median PtByPt.vi"("sample length"="Median sample length 20", "x"=w1199) -> ("median"=w1198:dbl)  [unwired: 2 in, 1 out]
    n519 = Square(x=w1198) -> (x^2=w1206:dbl)
    n520 = Multiply(x=w1198, y=2.7367) -> (x*y=w1202:dbl)
    n521 = Multiply(x=w1206, y=0.0108) -> (x*y=w1203:dbl)
    n522 = Add(x=w1202, y=w1203) -> (x+y=w1201:dbl)
    n523 = Add(x=-331.61, y=w1201) -> (x+y=w1164:dbl)
    n524 = case shown="False" "Autotune 11" {
      tunnel: w1166 -> [w1233 _]
      tunnel: [w1222 w1238] -> w1171
      tunnel: w1216 -> [_ w1237]
      tunnel: "PID Gains 11" -> [w1232 _]
      tunnel: "Reinitialize 11" -> [w1229 _]
      tunnel: w1217 -> [w1231 w1236]
      tunnel: w1215 -> [_ w1240]
      tunnel: w1164 -> [w1225 _]
      tunnel: "Set Point 11" -> [w1224 _]
      frame False {
        # "This code is to have 'bumpless' transfer from autotuning"
        n525 = Not(x=w1231) -> (.not. x?=w1228:bool)
        n526 = And(x="Automatic 11", y=w1228) -> (x .and. y?=w1230:bool)
        n527 = call-poly <vilib>:"PID Advanced.vi"("setpoint"=w1224, "auto? (T)"=w1230, "manual control"="MV: 11", "process variable"=w1225, "alpha"=10.0, "PID gains"=w1232, "dt (s)"=w1233, "reinitialize? (F)"=w1229) -> ("output"=w1222:dbl)  [unwired: 6 in, 1 out]
      }
      frame True {
        w1243 = 10000 ("sample length")
        # "Buffering data for parameters estimation"
        n528 = call <vilib>:"Data Queue PtByPt.vi"("initial queue element"=w1237, "initialize"=w1236, "sample length"=w1243, "input data point"=w1237) -> ("Current Queue"=→"Control Output 11":dbl[])  [unwired: 3 in, 4 out]
        n529 = Select(t=0.0, s=w1236, f="Excitation 11") -> (s? t:f=w1241:dbl)
        n530 = Add(x=w1240, y=w1241) -> (x+y=w1238:dbl)
        n531 = call <vilib>:"Data Queue PtByPt.vi"("initial queue element"=w1238, "initialize"=w1236, "sample length"=w1243, "input data point"=w1238) -> ("Current Queue"=→"Measurement 11":dbl[])  [unwired: 3 in, 4 out]
      }
    }
    n532 = feedback-in #21(w1171, w1213) -> ()
    n533 = Greater?(x=w1164, y="M-5") -> (0:w1152:bool)
    n534 = Add(x=w1195, y=w1183) -> (x+y=w1184:dbl)
    n535 = Subtract(x=w1195, y=w1183) -> (x-y=w1182:dbl)
    n536 = Equal?(x=w1193, y=w1171) -> (x = y?=w1190:bool)
    n537 = Greater?(x=w1171, y=w1193) -> (0:w1189:bool)
    n538 = Select(t=w1194, s=w1190, f=w1189) -> (s? t:f=w1169:bool)
    "PWM Output 11" <- w1169
    n539 = call "Plant System.vi"("Integrator ?"=w1212, "Plant Input"=w1171, "dt (s)"=w1166, "process parameters"=w1210) -> ("Plant Output"=w1211:dbl)  [unwired: 11 in]
    n540 = Increment(x="Set Point 11") -> (x+1=w1188:dbl)
    n541 = Decrement(x="Set Point 11") -> (x-1=w1187:dbl)
    n542 = Select(t=w1184, s=w1169, f=w1182) -> (s? t:f=w1197:dbl)
    n543 = Select(t=w1188, s=w1169, f=w1187) -> (s? t:f=w1186:dbl)
    n544 = Not(x=w1169) -> (.not. x?=w1168:bool)
    n545 = call-poly <vilib>:"DAQmx Create Virtual Channel.vi"("lines"=tag "cDAQ1Mod1/port0/line5", "line grouping"=w1175) -> ("task out"=w1177:refnum<k21>, "error out"=w1176:errorcluster)  [unwired: 12 in]
    n546 = call-poly <vilib>:"DAQmx Create Virtual Channel.vi"("lines"=tag "cDAQ1Mod2/port0/line5", "line grouping"=w1157) -> ("task out"=w1159:refnum<k21>, "error out"=w1158:errorcluster)  [unwired: 12 in]
    n547 = Build Array(w1164, "Set Point 11", w1186) -> (w1185:dbl[])
    n548 = Initialize Array("INLET 5 ON/OFF 3", 1 ("dimension size")) -> (w1154:bool[])
    n549 = Initialize Array(w1168, 1 ("dimension size")) -> (w1172:bool[])
    n550 = local write "MV: 11"(w1171) -> ()
    n551 = Add(x=w1192, y=w1195) -> (x+y=w1196:dbl)
    n552 = Build Array(w1185) -> (→"Real time Data 11":dbl[][])
    n553 = call-poly <vilib>:"DAQmx Write.vi"("task/channels in"=w1177, "auto start"=TRUE, "data"=w1172, "error in"=w1176) -> ("task out"=w1179:refnum<k21>, "error out"=w1180:errorcluster)  [unwired: 9 in, 1 out]
    n554 = call-poly <vilib>:"DAQmx Write.vi"("task/channels in"=w1159, "auto start"=TRUE, "data"=w1154, "error in"=w1158) -> ("task out"=w1161:refnum<k21>, "error out"=w1162:errorcluster)  [unwired: 9 in, 1 out]
    n555 = call <vilib>:"DAQmx Clear Task.vi"("task in"=w1179, "error in"=w1180) -> ("error out"=w1174:errorcluster)  [unwired: 13 in]
    n556 = call <vilib>:"DAQmx Clear Task.vi"("task in"=w1161, "error in"=w1162) -> ("error out"=w1156:errorcluster)  [unwired: 13 in]
    n557 = call <vilib>:"Simple Error Handler.vi"("error in (no error)"=w1174) -> ()  [unwired: 4 in, 5 out]
    n558 = call <vilib>:"Simple Error Handler.vi"("error in (no error)"=w1156) -> ()  [unwired: 4 in, 5 out]
  }
  n559 = Obtain Queue(element data type=0.0) -> (queue out=w7:refnum<queue>)  [unwired: 4 in, 2 out]
  n560 = while {
    shift-left: 0.0 ("Plant Output") -> [w1310]
    shift-right: [w1305] -> _
    tunnel: w52 -> [_]
    shift-right: [w1291] -> _
    shift-left: 0.01 -> [w1289]
    shift-right: [w1263] -> _
    shift-left: TRUE -> [w1288]
    shift-right: [w1265] -> _
    shift-left: w49 -> [w1287]
    shift-right: [w1290] -> _
    shift-left: w49 -> [w1286]
    tunnel: [w1260] -> w48
    tunnel: [w1246] -> w26
    tunnel: w7 -> [w1244]
    stop <- "Stop 10" stop-if-true
    w1251 = 1 items=["one channel for each line", "one channel for all lines"] ("line grouping")
    w1260 = 0.05 ("Sampling Time dt (s)")
    w1269 = 1 items=["one channel for each line", "one channel for all lines"] ("line grouping")
    w1277 = 0.5 ("x")
    w1304 = T7 {"static gain"=2.5, "lag (s)"=2.5, "deadtime (s)"=0.01, "load"=0.0, "deadband"=0.0, "sensor noise"=0.0, "initial PV"=30.0, "plant noise"=0.0}  # Process parameters
    w1306 = FALSE  # Integrator ?
    # "C."
    # "Inlet 11"
    # "Exhaust 3"
    # "B."
    # "A."
    # "A.Output to PWM Logic \nB. Simulated Plant\nC. Draw Chart"
    # "Main PID Loop Control"
    n561 = Multiply(x=w1260, y=1000.0) -> (x*y=w1303:dbl)
    n562 = Dequeue Element(queue=w1244) -> (element=w1245:dbl)  [unwired: 2 in, 3 out]
    n563 = Not(x="Autotune 10") -> (.not. x?=w1307:bool)
    n564 = feedback #22() -> (w1312:bool)  [unwired: 1 in]
    n565 = feedback-in #22("Autotune 10") -> ()
    n566 = Wait Until Next ms Multiple(millisecond multiple=w1303) -> ()  [unwired: 1 out]
    n567 = Exclusive Or(1:w1312, 2:"Autotune 10") -> (0:w1311:bool)
    n568 = feedback #23() -> (w1309:dbl)  [unwired: 1 in]
    n569 = Multiply(x=w1245, y=-1000.0) -> (x*y=w1293:dbl)
    n570 = call <vilib>:"Median PtByPt.vi"("sample length"="Median sample length 19", "x"=w1293) -> ("median"=w1292:dbl)  [unwired: 2 in, 1 out]
    n571 = Square(x=w1292) -> (x^2=w1300:dbl)
    n572 = Multiply(x=w1292, y=0.1121) -> (x*y=w1296:dbl)
    n573 = Multiply(x=w1300, y=0.0243) -> (x*y=w1297:dbl)
    n574 = Add(x=w1296, y=w1297) -> (x+y=w1295:dbl)
    n575 = Add(x=-235.77, y=w1295) -> (x+y=w1258:dbl)
    n576 = case shown="False" "Autotune 10" {
      tunnel: w1260 -> [w1327 _]
      tunnel: [w1316 w1332] -> w1265
      tunnel: w1310 -> [_ w1331]
      tunnel: "PID Gains 10" -> [w1326 _]
      tunnel: "Reinitialize 10" -> [w1323 _]
      tunnel: w1311 -> [w1325 w1330]
      tunnel: w1309 -> [_ w1334]
      tunnel: w1258 -> [w1319 _]
      tunnel: "Set Point 10" -> [w1318 _]
      frame False {
        # "This code is to have 'bumpless' transfer from autotuning"
        n577 = Not(x=w1325) -> (.not. x?=w1322:bool)
        n578 = And(x="Automatic 10", y=w1322) -> (x .and. y?=w1324:bool)
        n579 = call-poly <vilib>:"PID Advanced.vi"("setpoint"=w1318, "auto? (T)"=w1324, "manual control"="MV: 10", "process variable"=w1319, "alpha"=10.0, "PID gains"=w1326, "dt (s)"=w1327, "reinitialize? (F)"=w1323) -> ("output"=w1316:dbl)  [unwired: 6 in, 1 out]
      }
      frame True {
        w1337 = 10000 ("sample length")
        # "Buffering data for parameters estimation"
        n580 = call <vilib>:"Data Queue PtByPt.vi"("initial queue element"=w1331, "initialize"=w1330, "sample length"=w1337, "input data point"=w1331) -> ("Current Queue"=→"Control Output 10":dbl[])  [unwired: 3 in, 4 out]
        n581 = Select(t=0.0, s=w1330, f="Excitation 10") -> (s? t:f=w1335:dbl)
        n582 = Add(x=w1334, y=w1335) -> (x+y=w1332:dbl)
        n583 = call <vilib>:"Data Queue PtByPt.vi"("initial queue element"=w1332, "initialize"=w1330, "sample length"=w1337, "input data point"=w1332) -> ("Current Queue"=→"Measurement 10":dbl[])  [unwired: 3 in, 4 out]
      }
    }
    n584 = feedback-in #23(w1265, w1307) -> ()
    n585 = Greater?(x=w1258, y="M-3") -> (0:w1246:bool)
    n586 = Add(x=w1289, y=w1277) -> (x+y=w1278:dbl)
    n587 = Subtract(x=w1289, y=w1277) -> (x-y=w1276:dbl)
    n588 = Equal?(x=w1287, y=w1265) -> (x = y?=w1284:bool)
    n589 = Greater?(x=w1265, y=w1287) -> (0:w1283:bool)
    n590 = Select(t=w1288, s=w1284, f=w1283) -> (s? t:f=w1263:bool)
    "PWM Output 10" <- w1263
    n591 = call "Plant System.vi"("Integrator ?"=w1306, "Plant Input"=w1265, "dt (s)"=w1260, "process parameters"=w1304) -> ("Plant Output"=w1305:dbl)  [unwired: 11 in]
    n592 = Increment(x="Set Point 10") -> (x+1=w1282:dbl)
    n593 = Decrement(x="Set Point 10") -> (x-1=w1281:dbl)
    n594 = Select(t=w1278, s=w1263, f=w1276) -> (s? t:f=w1291:dbl)
    n595 = Select(t=w1282, s=w1263, f=w1281) -> (s? t:f=w1280:dbl)
    n596 = Not(x=w1263) -> (.not. x?=w1262:bool)
    n597 = call-poly <vilib>:"DAQmx Create Virtual Channel.vi"("lines"=tag "cDAQ1Mod8/port0/line7", "line grouping"=w1269) -> ("task out"=w1271:refnum<k21>, "error out"=w1270:errorcluster)  [unwired: 12 in]
    n598 = call-poly <vilib>:"DAQmx Create Virtual Channel.vi"("lines"=tag "cDAQ1Mod7/port0/line6", "line grouping"=w1251) -> ("task out"=w1253:refnum<k21>, "error out"=w1252:errorcluster)  [unwired: 12 in]
    n599 = Build Array(w1258, "Set Point 10", w1280) -> (w1279:dbl[])
    n600 = Initialize Array("INLET 3 ON/OFF 3", 1 ("dimension size")) -> (w1248:bool[])
    n601 = Initialize Array(w1262, 1 ("dimension size")) -> (w1266:bool[])
    n602 = local write "MV: 10"(w1265) -> ()
    n603 = Add(x=w1286, y=w1289) -> (x+y=w1290:dbl)
    n604 = Build Array(w1279) -> (→"Real time Data 10":dbl[][])
    n605 = call-poly <vilib>:"DAQmx Write.vi"("task/channels in"=w1271, "auto start"=TRUE, "data"=w1266, "error in"=w1270) -> ("task out"=w1273:refnum<k21>, "error out"=w1274:errorcluster)  [unwired: 9 in, 1 out]
    n606 = call-poly <vilib>:"DAQmx Write.vi"("task/channels in"=w1253, "auto start"=TRUE, "data"=w1248, "error in"=w1252) -> ("task out"=w1255:refnum<k21>, "error out"=w1256:errorcluster)  [unwired: 9 in, 1 out]
    n607 = call <vilib>:"DAQmx Clear Task.vi"("task in"=w1273, "error in"=w1274) -> ("error out"=w1268:errorcluster)  [unwired: 13 in]
    n608 = call <vilib>:"DAQmx Clear Task.vi"("task in"=w1255, "error in"=w1256) -> ("error out"=w1250:errorcluster)  [unwired: 13 in]
    n609 = call <vilib>:"Simple Error Handler.vi"("error in (no error)"=w1268) -> ()  [unwired: 4 in, 5 out]
    n610 = call <vilib>:"Simple Error Handler.vi"("error in (no error)"=w1250) -> ()  [unwired: 4 in, 5 out]
  }
  n611 = Obtain Queue(element data type=0.0) -> (queue out=w1:refnum<queue>)  [unwired: 4 in, 2 out]
  n612 = while {
    shift-left: 0.0 ("Plant Output") -> [w1404]
    shift-right: [w1399] -> _
    tunnel: w70 -> [_]
    shift-right: [w1385] -> _
    shift-left: 0.01 -> [w1383]
    shift-right: [w1357] -> _
    shift-left: TRUE -> [w1382]
    shift-right: [w1359] -> _
    shift-left: w67 -> [w1381]
    shift-right: [w1384] -> _
    shift-left: w67 -> [w1380]
    tunnel: [w1354] -> w66
    tunnel: [w1340] -> w23
    tunnel: w1 -> [w1338]
    stop <- "Stop 7" stop-if-true
    w1345 = 1 items=["one channel for each line", "one channel for all lines"] ("line grouping")
    w1354 = 0.05 ("Sampling Time dt (s)")
    w1363 = 1 items=["one channel for each line", "one channel for all lines"] ("line grouping")
    w1371 = 0.5 ("x")
    w1398 = T7 {"static gain"=2.5, "lag (s)"=2.5, "deadtime (s)"=0.01, "load"=0.0, "deadband"=0.0, "sensor noise"=0.0, "initial PV"=30.0, "plant noise"=0.0}  # Process parameters
    w1400 = FALSE  # Integrator ?
    # "C."
    # "Inlet 11"
    # "Exhaust 7"
    # "B."
    # "A."
    # "A.Output to PWM Logic \nB. Simulated Plant\nC. Draw Chart"
    # "Main PID Loop Control"
    n613 = Dequeue Element(queue=w1338) -> (element=w1339:dbl)  [unwired: 2 in, 3 out]
    n614 = Multiply(x=w1354, y=1000.0) -> (x*y=w1397:dbl)
    n615 = Not(x="Autotune 7") -> (.not. x?=w1401:bool)
    n616 = feedback #24() -> (w1406:bool)  [unwired: 1 in]
    n617 = feedback-in #24("Autotune 7") -> ()
    n618 = Wait Until Next ms Multiple(millisecond multiple=w1397) -> ()  [unwired: 1 out]
    n619 = Exclusive Or(1:w1406, 2:"Autotune 7") -> (0:w1405:bool)
    n620 = feedback #25() -> (w1403:dbl)  [unwired: 1 in]
    n621 = Multiply(x=w1339, y=-1000.0) -> (x*y=w1387:dbl)
    n622 = call <vilib>:"Median PtByPt.vi"("sample length"="Median sample length 16", "x"=w1387) -> ("median"=w1386:dbl)  [unwired: 2 in, 1 out]
    n623 = Square(x=w1386) -> (x^2=w1394:dbl)
    n624 = Multiply(x=w1386, y=-0.6707) -> (x*y=w1390:dbl)
    n625 = Multiply(x=w1394, y=0.0015) -> (x*y=w1391:dbl)
    n626 = Add(x=w1390, y=w1391) -> (x+y=w1389:dbl)
    n627 = Add(x=-0.8771, y=w1389) -> (x+y=w1352:dbl)
    n628 = case shown="False" "Autotune 7" {
      tunnel: w1354 -> [w1421 _]
      tunnel: [w1410 w1426] -> w1359
      tunnel: w1404 -> [_ w1425]
      tunnel: "PID Gains 7" -> [w1420 _]
      tunnel: "Reinitialize 7" -> [w1417 _]
      tunnel: w1405 -> [w1419 w1424]
      tunnel: w1403 -> [_ w1428]
      tunnel: w1352 -> [w1413 _]
      tunnel: "Set Point 7" -> [w1412 _]
      frame False {
        # "This code is to have 'bumpless' transfer from autotuning"
        n629 = Not(x=w1419) -> (.not. x?=w1416:bool)
        n630 = And(x="Automatic 7", y=w1416) -> (x .and. y?=w1418:bool)
        n631 = call-poly <vilib>:"PID Advanced.vi"("setpoint"=w1412, "auto? (T)"=w1418, "manual control"="MV: 7", "process variable"=w1413, "alpha"=10.0, "PID gains"=w1420, "dt (s)"=w1421, "reinitialize? (F)"=w1417) -> ("output"=w1410:dbl)  [unwired: 6 in, 1 out]
      }
      frame True {
        w1431 = 10000 ("sample length")
        # "Buffering data for parameters estimation"
        n632 = call <vilib>:"Data Queue PtByPt.vi"("initial queue element"=w1425, "initialize"=w1424, "sample length"=w1431, "input data point"=w1425) -> ("Current Queue"=→"Control Output 7":dbl[])  [unwired: 3 in, 4 out]
        n633 = Select(t=0.0, s=w1424, f="Excitation 7") -> (s? t:f=w1429:dbl)
        n634 = Add(x=w1428, y=w1429) -> (x+y=w1426:dbl)
        n635 = call <vilib>:"Data Queue PtByPt.vi"("initial queue element"=w1426, "initialize"=w1424, "sample length"=w1431, "input data point"=w1426) -> ("Current Queue"=→"Measurement 7":dbl[])  [unwired: 3 in, 4 out]
      }
    }
    n636 = feedback-in #25(w1359, w1401) -> ()
    n637 = Greater?(x=w1352, y="M-7") -> (0:w1340:bool)
    n638 = Add(x=w1383, y=w1371) -> (x+y=w1372:dbl)
    n639 = Subtract(x=w1383, y=w1371) -> (x-y=w1370:dbl)
    n640 = Equal?(x=w1381, y=w1359) -> (x = y?=w1378:bool)
    n641 = Greater?(x=w1359, y=w1381) -> (0:w1377:bool)
    n642 = Select(t=w1382, s=w1378, f=w1377) -> (s? t:f=w1357:bool)
    "PWM Output 7" <- w1357
    n643 = call "Plant System.vi"("Integrator ?"=w1400, "Plant Input"=w1359, "dt (s)"=w1354, "process parameters"=w1398) -> ("Plant Output"=w1399:dbl)  [unwired: 11 in]
    n644 = Increment(x="Set Point 7") -> (x+1=w1376:dbl)
    n645 = Decrement(x="Set Point 7") -> (x-1=w1375:dbl)
    n646 = Select(t=w1372, s=w1357, f=w1370) -> (s? t:f=w1385:dbl)
    n647 = Select(t=w1376, s=w1357, f=w1375) -> (s? t:f=w1374:dbl)
    n648 = Not(x=w1357) -> (.not. x?=w1356:bool)
    n649 = call-poly <vilib>:"DAQmx Create Virtual Channel.vi"("lines"=tag "cDAQ1Mod8/port0/line4", "line grouping"=w1363) -> ("task out"=w1365:refnum<k21>, "error out"=w1364:errorcluster)  [unwired: 12 in]
    n650 = call-poly <vilib>:"DAQmx Create Virtual Channel.vi"("lines"=tag "cDAQ1Mod7/port0/line3", "line grouping"=w1345) -> ("task out"=w1347:refnum<k21>, "error out"=w1346:errorcluster)  [unwired: 12 in]
    n651 = Build Array(w1352, "Set Point 7", w1374) -> (w1373:dbl[])
    n652 = Initialize Array("INLET 7 ON/OFF 2", 1 ("dimension size")) -> (w1342:bool[])
    n653 = Initialize Array(w1356, 1 ("dimension size")) -> (w1360:bool[])
    n654 = local write "MV: 7"(w1359) -> ()
    n655 = Add(x=w1380, y=w1383) -> (x+y=w1384:dbl)
    n656 = Build Array(w1373) -> (→"Real time Data 7":dbl[][])
    n657 = call-poly <vilib>:"DAQmx Write.vi"("task/channels in"=w1365, "auto start"=TRUE, "data"=w1360, "error in"=w1364) -> ("task out"=w1367:refnum<k21>, "error out"=w1368:errorcluster)  [unwired: 9 in, 1 out]
    n658 = call-poly <vilib>:"DAQmx Write.vi"("task/channels in"=w1347, "auto start"=TRUE, "data"=w1342, "error in"=w1346) -> ("task out"=w1349:refnum<k21>, "error out"=w1350:errorcluster)  [unwired: 9 in, 1 out]
    n659 = call <vilib>:"DAQmx Clear Task.vi"("task in"=w1367, "error in"=w1368) -> ("error out"=w1362:errorcluster)  [unwired: 13 in]
    n660 = call <vilib>:"DAQmx Clear Task.vi"("task in"=w1349, "error in"=w1350) -> ("error out"=w1344:errorcluster)  [unwired: 13 in]
    n661 = call <vilib>:"Simple Error Handler.vi"("error in (no error)"=w1362) -> ()  [unwired: 4 in, 5 out]
    n662 = call <vilib>:"Simple Error Handler.vi"("error in (no error)"=w1344) -> ()  [unwired: 4 in, 5 out]
  }
  n663 = Obtain Queue(element data type=0.0) -> (queue out=w11:refnum<queue>)  [unwired: 4 in, 2 out]
  n664 = while {
    shift-left: 0.0 ("Plant Output") -> [w1521]
    shift-right: [w1516] -> _
    tunnel: w142 -> [_]
    shift-right: [w1502] -> _
    shift-left: 0.01 -> [w1500]
    shift-right: [w1474] -> _
    shift-left: TRUE -> [w1499]
    shift-right: [w1476] -> _
    shift-left: w139 -> [w1498]
    shift-right: [w1501] -> _
    shift-left: w139 -> [w1497]
    tunnel: [w1471] -> w138
    tunnel: [w1468] -> w35
    tunnel: w21 -> [w1444]
    tunnel: w18 -> [w1443]
    tunnel: w17 -> [w1442]
    tunnel: w15 -> [w1441]
    tunnel: w13 -> [w1440]
    tunnel: w11 -> [w1439]
    tunnel: w10 -> [w1438]
    tunnel: w7 -> [w1437]
    tunnel: w5 -> [w1436]
    tunnel: w2 -> [w1433]
    tunnel: w1 -> [w1432]
    stop <- "Stop" stop-if-true
    w1461 = 1 items=["one channel for each line", "one channel for all lines"] ("line grouping")
    w1471 = 0.05 ("Sampling Time dt (s)")
    w1480 = 1 items=["one channel for each line", "one channel for all lines"] ("line grouping")
    w1488 = 0.5 ("x")
    w1515 = T7 {"static gain"=2.5, "lag (s)"=2.5, "deadtime (s)"=0.01, "load"=0.0, "deadband"=0.0, "sensor noise"=0.0, "initial PV"=30.0, "plant noise"=0.0}  # Process parameters
    w1517 = FALSE  # Integrator ?
    # "C."
    # "Inlet 11"
    # "Exhaust 11"
    # "B."
    # "A."
    # "A.Output to PWM Logic \nB. Simulated Plant\nC. Draw Chart"
    # "Main PID Loop Control"
    n665 = call-poly <vilib>:"DAQmx Read.vi"("task/channels in"=refnum<k21> "1_4_2_7_6_5") -> ("data"=w1450:dbl[])  [unwired: 12 in, 2 out]
    n666 = Index Array(array=w1450, index=0) -> (element=w1445:dbl)
    n667 = Index Array(array=w1450, index=1) -> (element=w1446:dbl)
    n668 = Index Array(array=w1450, index=2) -> (element=w1435:dbl)
    n669 = Index Array(array=w1450, index=5) -> (element=w1448:dbl)
    n670 = Index Array(array=w1450, index=4) -> (element=w1447:dbl)
    n671 = Index Array(array=w1450, index=3) -> (element=w1434:dbl)
    n672 = Enqueue Element(queue=w1439, element=w1445) -> ()  [unwired: 2 in, 3 out]
    n673 = Enqueue Element(queue=w1443, element=w1447) -> ()  [unwired: 2 in, 3 out]
    n674 = Enqueue Element(queue=w1437, element=w1446) -> ()  [unwired: 2 in, 3 out]
    n675 = Enqueue Element(queue=w1433, element=w1435) -> ()  [unwired: 2 in, 3 out]
    n676 = Enqueue Element(queue=w1444, element=w1448) -> ()  [unwired: 2 in, 3 out]
    n677 = Multiply(x=w1471, y=1000.0) -> (x*y=w1514:dbl)
    n678 = Enqueue Element(queue=w1438, element=w1445) -> ()  [unwired: 2 in, 3 out]
    n679 = Enqueue Element(queue=w1442, element=w1447) -> ()  [unwired: 2 in, 3 out]
    n680 = Enqueue Element(queue=w1436, element=w1446) -> ()  [unwired: 2 in, 3 out]
    n681 = Not(x="Autotune") -> (.not. x?=w1518:bool)
    n682 = feedback #26() -> (w1523:bool)  [unwired: 1 in]
    n683 = feedback-in #26("Autotune") -> ()
    n684 = Enqueue Element(queue=w1432, element=w1434) -> ()  [unwired: 2 in, 3 out]
    n685 = Wait Until Next ms Multiple(millisecond multiple=w1514) -> ()  [unwired: 1 out]
    n686 = Enqueue Element(queue=w1441, element=w1447) -> ()  [unwired: 2 in, 3 out]
    n687 = Exclusive Or(1:w1523, 2:"Autotune") -> (0:w1522:bool)
    n688 = feedback #27() -> (w1520:dbl)  [unwired: 1 in]
    n689 = Enqueue Element(queue=w1440, element=w1447) -> ()  [unwired: 2 in, 3 out]
    n690 = Multiply(x=w1448, y=-1000.0) -> (x*y=w1504:dbl)
    n691 = call <vilib>:"Median PtByPt.vi"("sample length"="Median sample length", "x"=w1504) -> ("median"=w1503:dbl)  [unwired: 2 in, 1 out]
    n692 = Square(x=w1503) -> (x^2=w1511:dbl)
    n693 = Multiply(x=w1503, y=-39.646) -> (x*y=w1507:dbl)
    n694 = Multiply(x=w1511, y=0.2324) -> (x*y=w1508:dbl)
    n695 = Add(x=w1507, y=w1508) -> (x+y=w1506:dbl)
    n696 = Add(x=1678.0, y=w1506) -> (x+y=w1469:dbl)
    n697 = case shown="False" "Autotune" {
      tunnel: w1471 -> [w1538 _]
      tunnel: [w1527 w1543] -> w1476
      tunnel: w1521 -> [_ w1542]
      tunnel: "PID Gains" -> [w1537 _]
      tunnel: "Reinitialize" -> [w1534 _]
      tunnel: w1522 -> [w1536 w1541]
      tunnel: w1520 -> [_ w1545]
      tunnel: w1469 -> [w1530 _]
      tunnel: "Set Point" -> [w1529 _]
      frame False {
        # "This code is to have 'bumpless' transfer from autotuning"
        n698 = Not(x=w1536) -> (.not. x?=w1533:bool)
        n699 = And(x="Automatic", y=w1533) -> (x .and. y?=w1535:bool)
        n700 = call-poly <vilib>:"PID Advanced.vi"("setpoint"=w1529, "auto? (T)"=w1535, "manual control"="MV:", "process variable"=w1530, "alpha"=10.0, "PID gains"=w1537, "dt (s)"=w1538, "reinitialize? (F)"=w1534) -> ("output"=w1527:dbl)  [unwired: 6 in, 1 out]
      }
      frame True {
        w1548 = 10000 ("sample length")
        # "Buffering data for parameters estimation"
        n701 = call <vilib>:"Data Queue PtByPt.vi"("initial queue element"=w1542, "initialize"=w1541, "sample length"=w1548, "input data point"=w1542) -> ("Current Queue"=→"Control Output":dbl[])  [unwired: 3 in, 4 out]
        n702 = Select(t=0.0, s=w1541, f="Excitation") -> (s? t:f=w1546:dbl)
        n703 = Add(x=w1545, y=w1546) -> (x+y=w1543:dbl)
        n704 = call <vilib>:"Data Queue PtByPt.vi"("initial queue element"=w1543, "initialize"=w1541, "sample length"=w1548, "input data point"=w1543) -> ("Current Queue"=→"Measurement":dbl[])  [unwired: 3 in, 4 out]
      }
    }
    n705 = feedback-in #27(w1476, w1518) -> ()
    n706 = Greater?(x=w1469, y="M-11") -> (0:w1468:bool)
    n707 = Add(x=w1500, y=w1488) -> (x+y=w1489:dbl)
    n708 = Subtract(x=w1500, y=w1488) -> (x-y=w1487:dbl)
    n709 = Equal?(x=w1498, y=w1476) -> (x = y?=w1495:bool)
    n710 = Greater?(x=w1476, y=w1498) -> (0:w1494:bool)
    n711 = Select(t=w1499, s=w1495, f=w1494) -> (s? t:f=w1474:bool)
    "PWM Output" <- w1474
    n712 = call "Plant System.vi"("Integrator ?"=w1517, "Plant Input"=w1476, "dt (s)"=w1471, "process parameters"=w1515) -> ("Plant Output"=w1516:dbl)  [unwired: 11 in]
    n713 = Increment(x="Set Point") -> (x+1=w1493:dbl)
    n714 = Decrement(x="Set Point") -> (x-1=w1492:dbl)
    n715 = Select(t=w1489, s=w1474, f=w1487) -> (s? t:f=w1502:dbl)
    n716 = Select(t=w1493, s=w1474, f=w1492) -> (s? t:f=w1491:dbl)
    n717 = Not(x=w1474) -> (.not. x?=w1473:bool)
    n718 = call-poly <vilib>:"DAQmx Create Virtual Channel.vi"("lines"=tag "cDAQ1Mod1/port0/line2", "line grouping"=w1480) -> ("task out"=w1482:refnum<k21>, "error out"=w1481:errorcluster)  [unwired: 12 in]
    n719 = call-poly <vilib>:"DAQmx Create Virtual Channel.vi"("lines"=tag "cDAQ1Mod2/port0/line2", "line grouping"=w1461) -> ("task out"=w1463:refnum<k21>, "error out"=w1462:errorcluster)  [unwired: 12 in]
    n720 = Build Array(w1469, "Set Point", w1491) -> (w1490:dbl[])
    n721 = Initialize Array("INLET", 1 ("dimension size")) -> (w1458:bool[])
    n722 = Initialize Array(w1473, 1 ("dimension size")) -> (w1477:bool[])
    n723 = local write "MV:"(w1476) -> ()
    n724 = Add(x=w1497, y=w1500) -> (x+y=w1501:dbl)
    n725 = Build Array(w1490) -> (→"Real time Data":dbl[][])
    n726 = call-poly <vilib>:"DAQmx Write.vi"("task/channels in"=w1482, "auto start"=TRUE, "data"=w1477, "error in"=w1481) -> ("task out"=w1484:refnum<k21>, "error out"=w1485:errorcluster)  [unwired: 9 in, 1 out]
    n727 = call-poly <vilib>:"DAQmx Write.vi"("task/channels in"=w1463, "auto start"=TRUE, "data"=w1458, "error in"=w1462) -> ("task out"=w1465:refnum<k21>, "error out"=w1466:errorcluster)  [unwired: 9 in, 1 out]
    n728 = call <vilib>:"DAQmx Clear Task.vi"("task in"=w1484, "error in"=w1485) -> ("error out"=w1479:errorcluster)  [unwired: 13 in]
    n729 = call <vilib>:"DAQmx Clear Task.vi"("task in"=w1465, "error in"=w1466) -> ("error out"=w1460:errorcluster)  [unwired: 13 in]
    n730 = call <vilib>:"Simple Error Handler.vi"("error in (no error)"=w1479) -> ()  [unwired: 4 in, 5 out]
    n731 = call <vilib>:"Simple Error Handler.vi"("error in (no error)"=w1460) -> ()  [unwired: 4 in, 5 out]
  }
  n732 = while {
    tunnel: w142 -> [_]
    tunnel: w138 -> [w1552]
    stop <- w1562 stop-if-true
    # "If dT and deadtime have similar values, the identification could evaluate deadtime as zero and this generates proportional gain equal to Inf. This code avoid gain changes in this situations."
    # "Autotuning Loop"
    n733 = local read "Control Output"() -> (w1564:dbl[])
    n734 = local read "Measurement"() -> (w1563:dbl[])
    n735 = case shown="\"Chien-Hrones-Reswick\"" "Control" {
      tunnel: w1564 -> [w1573 w1581 w1590 w1599]
      tunnel: w1563 -> [w1572 w1580 w1589 w1598]
      tunnel: [w1571 w1579 w1588 w1597] -> w1551
      tunnel: [w1570 w1578 w1587 w1596] -> w1550
      tunnel: w1552 -> [w1569 w1577 w1586 w1595]
      tunnel: [w1568 w1576 w1585 w1594] -> w1549
      tunnel: [w1567 w1575 w1584 w1593] -> w1554
      tunnel: "Type of controller" -> [w1566 w1574 w1583 w1592]
      frame "Ziegler-Nichols", Default {
        n736 = call-poly <vilib>:"PID Autotuning Design.vi"("Ziegler-Nichols Speed"="Ziegler-Nichols speed", "Type of Controller"=w1566, "dt (s)"=w1569, "Response signal"=w1572, "Stimulus signal"=w1573) -> ("PID gains"=w1567:T2, "response operating point"=w1570:dbl, "stimulus operating point"=w1571:dbl, "Plant Parameters"=w1568:T4)  [unwired: 3 in]
      }
      frame "Cohen-Coon" {
        n737 = call-poly <vilib>:"PID Autotuning Design.vi"("Type of Controller"=w1574, "dt (s)"=w1577, "Response signal"=w1580, "Stimulus signal"=w1581) -> ("PID gains"=w1575:T2, "response offset"=w1578:dbl, "stimulus offset"=w1579:dbl, "Plant Parameters"=w1576:T4)  [unwired: 4 in]
      }
      frame "Chien-Hrones-Reswick" {
        n738 = call-poly <vilib>:"PID Autotuning Design.vi"("Tuning specifications"="Tuning specifications", "Type of Controller"=w1583, "dt (s)"=w1586, "Response signal"=w1589, "Stimulus signal"=w1590) -> ("PID gains"=w1584:T2, "response offset"=w1587:dbl, "stimulus offset"=w1588:dbl, "Plant Parameters"=w1585:T4)  [unwired: 3 in]
      }
      frame "Internal Model Control" {
        n739 = call-poly <vilib>:"PID Autotuning Design.vi"("Desired Time Constant (tau_c)"="Multiplicative factor", "Type of Controller"=w1592, "dt (s)"=w1595, "Response signal"=w1598, "Stimulus signal"=w1599) -> ("PID gains"=w1593:T2, "response offset"=w1596:dbl, "stimulus offset"=w1597:dbl, "Plant Parameters"=w1594:T4)  [unwired: 3 in]
      }
    }
    "Stimulus operating point" <- w1551
    "Response operating point" <- w1550
    "Identified Plant Parameters" <- w1549
    n740 = Unbundle(w1554) -> ("proportional gain (Kc)"=w1557:dbl)  [unwired: 2 out]
    n741 = Equal?(x=w1557, y=inf) -> (x = y?=w1556:bool)
    n742 = feedback #28() -> (w1555:T2)  [unwired: 1 in]
    n743 = Select(t=w1555, s=w1556, f=w1554) -> (s? t:f=w1553:T2)
    "Tuned PID gains" <- w1553
    n744 = feedback-in #28(w1553) -> ()
    n745 = case shown="True" "Accept gain" {
      tunnel: w1553 -> [_ w1600]
      frame False {
      }
      frame True {
        n746 = local write "PID Gains"(w1600) -> ()
      }
    }
    n747 = local read "Stop"() -> (w1562:bool)
  }
  n748 = while {
    shift-left: 0.0 ("Plant Output") -> [w1667]
    shift-right: [w1662] -> _
    tunnel: w40 -> [_]
    shift-right: [w1648] -> _
    shift-left: 0.01 -> [w1646]
    shift-right: [w1620] -> _
    shift-left: TRUE -> [w1645]
    shift-right: [w1622] -> _
    shift-left: w37 -> [w1644]
    shift-right: [w1647] -> _
    shift-left: w37 -> [w1643]
    tunnel: [w1617] -> w36
    tunnel: [w1603] -> w28
    tunnel: w11 -> [w1601]
    stop <- "Stop 12" stop-if-true
    w1608 = 1 items=["one channel for each line", "one channel for all lines"] ("line grouping")
    w1617 = 0.05 ("Sampling Time dt (s)")
    w1626 = 1 items=["one channel for each line", "one channel for all lines"] ("line grouping")
    w1634 = 0.5 ("x")
    w1661 = T7 {"static gain"=2.5, "lag (s)"=2.5, "deadtime (s)"=0.01, "load"=0.0, "deadband"=0.0, "sensor noise"=0.0, "initial PV"=30.0, "plant noise"=0.0}  # Process parameters
    w1663 = FALSE  # Integrator ?
    # "C."
    # "Inlet 11"
    # "Exhaust 1"
    # "B."
    # "A."
    # "A.Output to PWM Logic \nB. Simulated Plant\nC. Draw Chart"
    # "Main PID Loop Control"
    n749 = Dequeue Element(queue=w1601) -> (element=w1602:dbl)  [unwired: 2 in, 3 out]
    n750 = Multiply(x=w1617, y=1000.0) -> (x*y=w1660:dbl)
    n751 = Not(x="Autotune 12") -> (.not. x?=w1664:bool)
    n752 = feedback #29() -> (w1669:bool)  [unwired: 1 in]
    n753 = feedback-in #29("Autotune 12") -> ()
    n754 = Wait Until Next ms Multiple(millisecond multiple=w1660) -> ()  [unwired: 1 out]
    n755 = Exclusive Or(1:w1669, 2:"Autotune 12") -> (0:w1668:bool)
    n756 = feedback #30() -> (w1666:dbl)  [unwired: 1 in]
    n757 = Multiply(x=w1602, y=-1000.0) -> (x*y=w1650:dbl)
    n758 = call <vilib>:"Median PtByPt.vi"("sample length"="Median sample length 21", "x"=w1650) -> ("median"=w1649:dbl)  [unwired: 2 in, 1 out]
    n759 = Square(x=w1649) -> (x^2=w1657:dbl)
    n760 = Multiply(x=w1649, y=2.7367) -> (x*y=w1653:dbl)
    n761 = Multiply(x=w1657, y=0.0108) -> (x*y=w1654:dbl)
    n762 = Add(x=w1653, y=w1654) -> (x+y=w1652:dbl)
    n763 = Add(x=-331.61, y=w1652) -> (x+y=w1615:dbl)
    n764 = case shown="False" "Autotune 12" {
      tunnel: w1617 -> [w1684 _]
      tunnel: [w1673 w1689] -> w1622
      tunnel: w1667 -> [_ w1688]
      tunnel: "PID Gains 12" -> [w1683 _]
      tunnel: "Reinitialize 12" -> [w1680 _]
      tunnel: w1668 -> [w1682 w1687]
      tunnel: w1666 -> [_ w1691]
      tunnel: w1615 -> [w1676 _]
      tunnel: "Set Point 12" -> [w1675 _]
      frame False {
        # "This code is to have 'bumpless' transfer from autotuning"
        n765 = Not(x=w1682) -> (.not. x?=w1679:bool)
        n766 = And(x="Automatic 12", y=w1679) -> (x .and. y?=w1681:bool)
        n767 = call-poly <vilib>:"PID Advanced.vi"("setpoint"=w1675, "auto? (T)"=w1681, "manual control"="MV: 12", "process variable"=w1676, "alpha"=10.0, "PID gains"=w1683, "dt (s)"=w1684, "reinitialize? (F)"=w1680) -> ("output"=w1673:dbl)  [unwired: 6 in, 1 out]
      }
      frame True {
        w1694 = 10000 ("sample length")
        # "Buffering data for parameters estimation"
        n768 = call <vilib>:"Data Queue PtByPt.vi"("initial queue element"=w1688, "initialize"=w1687, "sample length"=w1694, "input data point"=w1688) -> ("Current Queue"=→"Control Output 12":dbl[])  [unwired: 3 in, 4 out]
        n769 = Select(t=0.0, s=w1687, f="Excitation 12") -> (s? t:f=w1692:dbl)
        n770 = Add(x=w1691, y=w1692) -> (x+y=w1689:dbl)
        n771 = call <vilib>:"Data Queue PtByPt.vi"("initial queue element"=w1689, "initialize"=w1687, "sample length"=w1694, "input data point"=w1689) -> ("Current Queue"=→"Measurement 12":dbl[])  [unwired: 3 in, 4 out]
      }
    }
    n772 = feedback-in #30(w1622, w1664) -> ()
    n773 = Greater?(x=w1615, y="M-1") -> (0:w1603:bool)
    n774 = Add(x=w1646, y=w1634) -> (x+y=w1635:dbl)
    n775 = Subtract(x=w1646, y=w1634) -> (x-y=w1633:dbl)
    n776 = Equal?(x=w1644, y=w1622) -> (x = y?=w1641:bool)
    n777 = Greater?(x=w1622, y=w1644) -> (0:w1640:bool)
    n778 = Select(t=w1645, s=w1641, f=w1640) -> (s? t:f=w1620:bool)
    "PWM Output 12" <- w1620
    n779 = call "Plant System.vi"("Integrator ?"=w1663, "Plant Input"=w1622, "dt (s)"=w1617, "process parameters"=w1661) -> ("Plant Output"=w1662:dbl)  [unwired: 11 in]
    n780 = Increment(x="Set Point 12") -> (x+1=w1639:dbl)
    n781 = Decrement(x="Set Point 12") -> (x-1=w1638:dbl)
    n782 = Select(t=w1635, s=w1620, f=w1633) -> (s? t:f=w1648:dbl)
    n783 = Select(t=w1639, s=w1620, f=w1638) -> (s? t:f=w1637:dbl)
    n784 = Not(x=w1620) -> (.not. x?=w1619:bool)
    n785 = call-poly <vilib>:"DAQmx Create Virtual Channel.vi"("lines"=tag "cDAQ1Mod1/port0/line7", "line grouping"=w1626) -> ("task out"=w1628:refnum<k21>, "error out"=w1627:errorcluster)  [unwired: 12 in]
    n786 = call-poly <vilib>:"DAQmx Create Virtual Channel.vi"("lines"=tag "cDAQ1Mod2/port0/line7", "line grouping"=w1608) -> ("task out"=w1610:refnum<k21>, "error out"=w1609:errorcluster)  [unwired: 12 in]
    n787 = Build Array(w1615, "Set Point 12", w1637) -> (w1636:dbl[])
    n788 = Initialize Array("INLET 1 ON/OFF 3", 1 ("dimension size")) -> (w1605:bool[])
    n789 = Initialize Array(w1619, 1 ("dimension size")) -> (w1623:bool[])
    n790 = local write "MV: 12"(w1622) -> ()
    n791 = Add(x=w1643, y=w1646) -> (x+y=w1647:dbl)
    n792 = Build Array(w1636) -> (→"Real time Data 12":dbl[][])
    n793 = call-poly <vilib>:"DAQmx Write.vi"("task/channels in"=w1628, "auto start"=TRUE, "data"=w1623, "error in"=w1627) -> ("task out"=w1630:refnum<k21>, "error out"=w1631:errorcluster)  [unwired: 9 in, 1 out]
    n794 = call-poly <vilib>:"DAQmx Write.vi"("task/channels in"=w1610, "auto start"=TRUE, "data"=w1605, "error in"=w1609) -> ("task out"=w1612:refnum<k21>, "error out"=w1613:errorcluster)  [unwired: 9 in, 1 out]
    n795 = call <vilib>:"DAQmx Clear Task.vi"("task in"=w1630, "error in"=w1631) -> ("error out"=w1625:errorcluster)  [unwired: 13 in]
    n796 = call <vilib>:"DAQmx Clear Task.vi"("task in"=w1612, "error in"=w1613) -> ("error out"=w1607:errorcluster)  [unwired: 13 in]
    n797 = call <vilib>:"Simple Error Handler.vi"("error in (no error)"=w1625) -> ()  [unwired: 4 in, 5 out]
    n798 = call <vilib>:"Simple Error Handler.vi"("error in (no error)"=w1607) -> ()  [unwired: 4 in, 5 out]
  }
  n799 = Compound Arithmetic op=OR(w33, w35, w32, w31, w30, w29, w28, w27, w26, w25, w24, w23) -> (w34:bool)
  "?" <- w34
  n800 = case shown="True" w34 {
    frame False {
    }
    frame True {
      n801 = call <vilib>:"Beep.vi"("use system alert? (T)"=FALSE, "duration (msec)"=u32 2000, "frequency (Hz)"=u32 15000) -> ()  [unwired: 9 in]
    }
  }
  n802 = control-ref of="PnoData"() -> (w103:refnum<vi>)
  n803 = call <instrlib>:"PDI data xyzaer loop.vi"("Data Ready Refnum"=w103, "FrameCount Ctl Ref"=w113, "error in (no error)"=w123, "xyzaer array\nRefnum"=w112, "Stop Ctl Ref"=w121, "pDev"=w122) -> ("error out"=w110:errorcluster, "Loop Iter"=w114:i32, "dup pDev"=w111:u32)  [unwired: 3 out]
  n804 = local write "Loop Iter"(w114) -> ()
  n805 = local write "Stop 11"(w46) -> ()
  n806 = local write "Stop 12"(w40) -> ()
  n807 = local write "Stop 10"(w52) -> ()
  n808 = local write "Stop 9"(w58) -> ()
  n809 = call <instrlib>:"PDI action stopcont.vi"("error in (no error)"=w110, "pDev"=w111) -> ("error out"=w119:errorcluster, "Running"=w124:bool, "dup pDev"=w125:u32)  [unwired: 7 out]
  n810 = local write "Stop 8"(w64) -> ()
  n811 = local write "Stop 7"(w70) -> ()
  n812 = local write "Running"(w124) -> ()
  n813 = case shown="No Error" w110 {
    tunnel: w118 -> [w1698 _]
    frame No Error {
      # "Success up to here"
      n814 = call "Elapsed Time"("Set Start Time (s)"=w1698) -> ("Present Text"=w1700:string, "Elapsed Time Text"=w1699:string)  [unwired: 4 in, 13 out]
      n815 = local write "Stop Time Text"(w1700) -> ()
      n816 = local write "Elapsed Time Text"(w1699) -> ()
    }
    frame Error {
      # "Error somewhere;\nStop Time is irrelevant"
    }
  }
  n817 = while {
    tunnel: w46 -> [_]
    tunnel: w42 -> [w1704]
    stop <- w1714 stop-if-true
    # "If dT and deadtime have similar values, the identification could evaluate deadtime as zero and this generates proportional gain equal to Inf. This code avoid gain changes in this situations."
    # "Autotuning Loop"
    n818 = local read "Control Output 11"() -> (w1716:dbl[])
    n819 = local read "Measurement 11"() -> (w1715:dbl[])
    n820 = case shown="\"Chien-Hrones-Reswick\"" "Control 11" {
      tunnel: w1716 -> [w1725 w1733 w1742 w1751]
      tunnel: w1715 -> [w1724 w1732 w1741 w1750]
      tunnel: [w1723 w1731 w1740 w1749] -> w1703
      tunnel: [w1722 w1730 w1739 w1748] -> w1702
      tunnel: w1704 -> [w1721 w1729 w1738 w1747]
      tunnel: [w1720 w1728 w1737 w1746] -> w1701
      tunnel: [w1719 w1727 w1736 w1745] -> w1706
      tunnel: "Type of controller 11" -> [w1718 w1726 w1735 w1744]
      frame "Ziegler-Nichols", Default {
        n821 = call-poly <vilib>:"PID Autotuning Design.vi"("Ziegler-Nichols Speed"="Ziegler-Nichols speed 11", "Type of Controller"=w1718, "dt (s)"=w1721, "Response signal"=w1724, "Stimulus signal"=w1725) -> ("PID gains"=w1719:T2, "response operating point"=w1722:dbl, "stimulus operating point"=w1723:dbl, "Plant Parameters"=w1720:T4)  [unwired: 3 in]
      }
      frame "Cohen-Coon" {
        n822 = call-poly <vilib>:"PID Autotuning Design.vi"("Type of Controller"=w1726, "dt (s)"=w1729, "Response signal"=w1732, "Stimulus signal"=w1733) -> ("PID gains"=w1727:T2, "response offset"=w1730:dbl, "stimulus offset"=w1731:dbl, "Plant Parameters"=w1728:T4)  [unwired: 4 in]
      }
      frame "Chien-Hrones-Reswick" {
        n823 = call-poly <vilib>:"PID Autotuning Design.vi"("Tuning specifications"="Tuning specifications 11", "Type of Controller"=w1735, "dt (s)"=w1738, "Response signal"=w1741, "Stimulus signal"=w1742) -> ("PID gains"=w1736:T2, "response offset"=w1739:dbl, "stimulus offset"=w1740:dbl, "Plant Parameters"=w1737:T4)  [unwired: 3 in]
      }
      frame "Internal Model Control" {
        n824 = call-poly <vilib>:"PID Autotuning Design.vi"("Desired Time Constant (tau_c)"="Multiplicative factor 11", "Type of Controller"=w1744, "dt (s)"=w1747, "Response signal"=w1750, "Stimulus signal"=w1751) -> ("PID gains"=w1745:T2, "response offset"=w1748:dbl, "stimulus offset"=w1749:dbl, "Plant Parameters"=w1746:T4)  [unwired: 3 in]
      }
    }
    "Stimulus operating point 11" <- w1703
    "Response operating point 11" <- w1702
    "Identified Plant Parameters 11" <- w1701
    n825 = Unbundle(w1706) -> ("proportional gain (Kc)"=w1709:dbl)  [unwired: 2 out]
    n826 = Equal?(x=w1709, y=inf) -> (x = y?=w1708:bool)
    n827 = feedback #31() -> (w1707:T2)  [unwired: 1 in]
    n828 = Select(t=w1707, s=w1708, f=w1706) -> (s? t:f=w1705:T2)
    "Tuned PID gains 11" <- w1705
    n829 = feedback-in #31(w1705) -> ()
    n830 = case shown="True" "Accept gain 11" {
      tunnel: w1705 -> [_ w1752]
      frame False {
      }
      frame True {
        n831 = local write "PID Gains 11"(w1752) -> ()
      }
    }
    n832 = local read "Stop 11"() -> (w1714:bool)
  }
  n833 = while {
    tunnel: w40 -> [_]
    tunnel: w36 -> [w1756]
    stop <- w1766 stop-if-true
    # "If dT and deadtime have similar values, the identification could evaluate deadtime as zero and this generates proportional gain equal to Inf. This code avoid gain changes in this situations."
    # "Autotuning Loop"
    n834 = local read "Control Output 12"() -> (w1768:dbl[])
    n835 = local read "Measurement 12"() -> (w1767:dbl[])
    n836 = case shown="\"Chien-Hrones-Reswick\"" "Control 12" {
      tunnel: w1768 -> [w1777 w1785 w1794 w1803]
      tunnel: w1767 -> [w1776 w1784 w1793 w1802]
      tunnel: [w1775 w1783 w1792 w1801] -> w1755
      tunnel: [w1774 w1782 w1791 w1800] -> w1754
      tunnel: w1756 -> [w1773 w1781 w1790 w1799]
      tunnel: [w1772 w1780 w1789 w1798] -> w1753
      tunnel: [w1771 w1779 w1788 w1797] -> w1758
      tunnel: "Type of controller 12" -> [w1770 w1778 w1787 w1796]
      frame "Ziegler-Nichols", Default {
        n837 = call-poly <vilib>:"PID Autotuning Design.vi"("Ziegler-Nichols Speed"="Ziegler-Nichols speed 12", "Type of Controller"=w1770, "dt (s)"=w1773, "Response signal"=w1776, "Stimulus signal"=w1777) -> ("PID gains"=w1771:T2, "response operating point"=w1774:dbl, "stimulus operating point"=w1775:dbl, "Plant Parameters"=w1772:T4)  [unwired: 3 in]
      }
      frame "Cohen-Coon" {
        n838 = call-poly <vilib>:"PID Autotuning Design.vi"("Type of Controller"=w1778, "dt (s)"=w1781, "Response signal"=w1784, "Stimulus signal"=w1785) -> ("PID gains"=w1779:T2, "response offset"=w1782:dbl, "stimulus offset"=w1783:dbl, "Plant Parameters"=w1780:T4)  [unwired: 4 in]
      }
      frame "Chien-Hrones-Reswick" {
        n839 = call-poly <vilib>:"PID Autotuning Design.vi"("Tuning specifications"="Tuning specifications 12", "Type of Controller"=w1787, "dt (s)"=w1790, "Response signal"=w1793, "Stimulus signal"=w1794) -> ("PID gains"=w1788:T2, "response offset"=w1791:dbl, "stimulus offset"=w1792:dbl, "Plant Parameters"=w1789:T4)  [unwired: 3 in]
      }
      frame "Internal Model Control" {
        n840 = call-poly <vilib>:"PID Autotuning Design.vi"("Desired Time Constant (tau_c)"="Multiplicative factor 12", "Type of Controller"=w1796, "dt (s)"=w1799, "Response signal"=w1802, "Stimulus signal"=w1803) -> ("PID gains"=w1797:T2, "response offset"=w1800:dbl, "stimulus offset"=w1801:dbl, "Plant Parameters"=w1798:T4)  [unwired: 3 in]
      }
    }
    "Stimulus operating point 12" <- w1755
    "Response operating point 12" <- w1754
    "Identified Plant Parameters 12" <- w1753
    n841 = Unbundle(w1758) -> ("proportional gain (Kc)"=w1761:dbl)  [unwired: 2 out]
    n842 = Equal?(x=w1761, y=inf) -> (x = y?=w1760:bool)
    n843 = feedback #32() -> (w1759:T2)  [unwired: 1 in]
    n844 = Select(t=w1759, s=w1760, f=w1758) -> (s? t:f=w1757:T2)
    "Tuned PID gains 12" <- w1757
    n845 = feedback-in #32(w1757) -> ()
    n846 = case shown="True" "Accept gain 12" {
      tunnel: w1757 -> [_ w1804]
      frame False {
      }
      frame True {
        n847 = local write "PID Gains 12"(w1804) -> ()
      }
    }
    n848 = local read "Stop 12"() -> (w1766:bool)
  }
  n849 = while {
    tunnel: w52 -> [_]
    tunnel: w48 -> [w1808]
    stop <- w1818 stop-if-true
    # "If dT and deadtime have similar values, the identification could evaluate deadtime as zero and this generates proportional gain equal to Inf. This code avoid gain changes in this situations."
    # "Autotuning Loop"
    n850 = local read "Control Output 10"() -> (w1820:dbl[])
    n851 = local read "Measurement 10"() -> (w1819:dbl[])
    n852 = case shown="\"Chien-Hrones-Reswick\"" "Control 10" {
      tunnel: w1820 -> [w1829 w1837 w1846 w1855]
      tunnel: w1819 -> [w1828 w1836 w1845 w1854]
      tunnel: [w1827 w1835 w1844 w1853] -> w1807
      tunnel: [w1826 w1834 w1843 w1852] -> w1806
      tunnel: w1808 -> [w1825 w1833 w1842 w1851]
      tunnel: [w1824 w1832 w1841 w1850] -> w1805
      tunnel: [w1823 w1831 w1840 w1849] -> w1810
      tunnel: "Type of controller 10" -> [w1822 w1830 w1839 w1848]
      frame "Ziegler-Nichols", Default {
        n853 = call-poly <vilib>:"PID Autotuning Design.vi"("Ziegler-Nichols Speed"="Ziegler-Nichols speed 10", "Type of Controller"=w1822, "dt (s)"=w1825, "Response signal"=w1828, "Stimulus signal"=w1829) -> ("PID gains"=w1823:T2, "response operating point"=w1826:dbl, "stimulus operating point"=w1827:dbl, "Plant Parameters"=w1824:T4)  [unwired: 3 in]
      }
      frame "Cohen-Coon" {
        n854 = call-poly <vilib>:"PID Autotuning Design.vi"("Type of Controller"=w1830, "dt (s)"=w1833, "Response signal"=w1836, "Stimulus signal"=w1837) -> ("PID gains"=w1831:T2, "response offset"=w1834:dbl, "stimulus offset"=w1835:dbl, "Plant Parameters"=w1832:T4)  [unwired: 4 in]
      }
      frame "Chien-Hrones-Reswick" {
        n855 = call-poly <vilib>:"PID Autotuning Design.vi"("Tuning specifications"="Tuning specifications 10", "Type of Controller"=w1839, "dt (s)"=w1842, "Response signal"=w1845, "Stimulus signal"=w1846) -> ("PID gains"=w1840:T2, "response offset"=w1843:dbl, "stimulus offset"=w1844:dbl, "Plant Parameters"=w1841:T4)  [unwired: 3 in]
      }
      frame "Internal Model Control" {
        n856 = call-poly <vilib>:"PID Autotuning Design.vi"("Desired Time Constant (tau_c)"="Multiplicative factor 10", "Type of Controller"=w1848, "dt (s)"=w1851, "Response signal"=w1854, "Stimulus signal"=w1855) -> ("PID gains"=w1849:T2, "response offset"=w1852:dbl, "stimulus offset"=w1853:dbl, "Plant Parameters"=w1850:T4)  [unwired: 3 in]
      }
    }
    "Stimulus operating point 10" <- w1807
    "Response operating point 10" <- w1806
    "Identified Plant Parameters 10" <- w1805
    n857 = Unbundle(w1810) -> ("proportional gain (Kc)"=w1813:dbl)  [unwired: 2 out]
    n858 = Equal?(x=w1813, y=inf) -> (x = y?=w1812:bool)
    n859 = feedback #33() -> (w1811:T2)  [unwired: 1 in]
    n860 = Select(t=w1811, s=w1812, f=w1810) -> (s? t:f=w1809:T2)
    "Tuned PID gains 10" <- w1809
    n861 = feedback-in #33(w1809) -> ()
    n862 = case shown="True" "Accept gain 10" {
      tunnel: w1809 -> [_ w1856]
      frame False {
      }
      frame True {
        n863 = local write "PID Gains 10"(w1856) -> ()
      }
    }
    n864 = local read "Stop 10"() -> (w1818:bool)
  }
  n865 = while {
    tunnel: w58 -> [_]
    tunnel: w54 -> [w1860]
    stop <- w1870 stop-if-true
    # "If dT and deadtime have similar values, the identification could evaluate deadtime as zero and this generates proportional gain equal to Inf. This code avoid gain changes in this situations."
    # "Autotuning Loop"
    n866 = local read "Control Output 9"() -> (w1872:dbl[])
    n867 = local read "Measurement 9"() -> (w1871:dbl[])
    n868 = case shown="\"Chien-Hrones-Reswick\"" "Control 9" {
      tunnel: w1872 -> [w1881 w1889 w1898 w1907]
      tunnel: w1871 -> [w1880 w1888 w1897 w1906]
      tunnel: [w1879 w1887 w1896 w1905] -> w1859
      tunnel: [w1878 w1886 w1895 w1904] -> w1858
      tunnel: w1860 -> [w1877 w1885 w1894 w1903]
      tunnel: [w1876 w1884 w1893 w1902] -> w1857
      tunnel: [w1875 w1883 w1892 w1901] -> w1862
      tunnel: "Type of controller 9" -> [w1874 w1882 w1891 w1900]
      frame "Ziegler-Nichols", Default {
        n869 = call-poly <vilib>:"PID Autotuning Design.vi"("Ziegler-Nichols Speed"="Ziegler-Nichols speed 9", "Type of Controller"=w1874, "dt (s)"=w1877, "Response signal"=w1880, "Stimulus signal"=w1881) -> ("PID gains"=w1875:T2, "response operating point"=w1878:dbl, "stimulus operating point"=w1879:dbl, "Plant Parameters"=w1876:T4)  [unwired: 3 in]
      }
      frame "Cohen-Coon" {
        n870 = call-poly <vilib>:"PID Autotuning Design.vi"("Type of Controller"=w1882, "dt (s)"=w1885, "Response signal"=w1888, "Stimulus signal"=w1889) -> ("PID gains"=w1883:T2, "response offset"=w1886:dbl, "stimulus offset"=w1887:dbl, "Plant Parameters"=w1884:T4)  [unwired: 4 in]
      }
      frame "Chien-Hrones-Reswick" {
        n871 = call-poly <vilib>:"PID Autotuning Design.vi"("Tuning specifications"="Tuning specifications 9", "Type of Controller"=w1891, "dt (s)"=w1894, "Response signal"=w1897, "Stimulus signal"=w1898) -> ("PID gains"=w1892:T2, "response offset"=w1895:dbl, "stimulus offset"=w1896:dbl, "Plant Parameters"=w1893:T4)  [unwired: 3 in]
      }
      frame "Internal Model Control" {
        n872 = call-poly <vilib>:"PID Autotuning Design.vi"("Desired Time Constant (tau_c)"="Multiplicative factor 9", "Type of Controller"=w1900, "dt (s)"=w1903, "Response signal"=w1906, "Stimulus signal"=w1907) -> ("PID gains"=w1901:T2, "response offset"=w1904:dbl, "stimulus offset"=w1905:dbl, "Plant Parameters"=w1902:T4)  [unwired: 3 in]
      }
    }
    "Stimulus operating point 9" <- w1859
    "Response operating point 9" <- w1858
    "Identified Plant Parameters 9" <- w1857
    n873 = Unbundle(w1862) -> ("proportional gain (Kc)"=w1865:dbl)  [unwired: 2 out]
    n874 = Equal?(x=w1865, y=inf) -> (x = y?=w1864:bool)
    n875 = feedback #34() -> (w1863:T2)  [unwired: 1 in]
    n876 = Select(t=w1863, s=w1864, f=w1862) -> (s? t:f=w1861:T2)
    "Tuned PID gains 9" <- w1861
    n877 = feedback-in #34(w1861) -> ()
    n878 = case shown="True" "Accept gain 9" {
      tunnel: w1861 -> [_ w1908]
      frame False {
      }
      frame True {
        n879 = local write "PID Gains 9"(w1908) -> ()
      }
    }
    n880 = local read "Stop 9"() -> (w1870:bool)
  }
  n881 = while {
    tunnel: w64 -> [_]
    tunnel: w60 -> [w1912]
    stop <- w1922 stop-if-true
    # "If dT and deadtime have similar values, the identification could evaluate deadtime as zero and this generates proportional gain equal to Inf. This code avoid gain changes in this situations."
    # "Autotuning Loop"
    n882 = local read "Control Output 8"() -> (w1924:dbl[])
    n883 = local read "Measurement 8"() -> (w1923:dbl[])
    n884 = case shown="\"Chien-Hrones-Reswick\"" "Control 8" {
      tunnel: w1924 -> [w1933 w1941 w1950 w1959]
      tunnel: w1923 -> [w1932 w1940 w1949 w1958]
      tunnel: [w1931 w1939 w1948 w1957] -> w1911
      tunnel: [w1930 w1938 w1947 w1956] -> w1910
      tunnel: w1912 -> [w1929 w1937 w1946 w1955]
      tunnel: [w1928 w1936 w1945 w1954] -> w1909
      tunnel: [w1927 w1935 w1944 w1953] -> w1914
      tunnel: "Type of controller 8" -> [w1926 w1934 w1943 w1952]
      frame "Ziegler-Nichols", Default {
        n885 = call-poly <vilib>:"PID Autotuning Design.vi"("Ziegler-Nichols Speed"="Ziegler-Nichols speed 8", "Type of Controller"=w1926, "dt (s)"=w1929, "Response signal"=w1932, "Stimulus signal"=w1933) -> ("PID gains"=w1927:T2, "response operating point"=w1930:dbl, "stimulus operating point"=w1931:dbl, "Plant Parameters"=w1928:T4)  [unwired: 3 in]
      }
      frame "Cohen-Coon" {
        n886 = call-poly <vilib>:"PID Autotuning Design.vi"("Type of Controller"=w1934, "dt (s)"=w1937, "Response signal"=w1940, "Stimulus signal"=w1941) -> ("PID gains"=w1935:T2, "response offset"=w1938:dbl, "stimulus offset"=w1939:dbl, "Plant Parameters"=w1936:T4)  [unwired: 4 in]
      }
      frame "Chien-Hrones-Reswick" {
        n887 = call-poly <vilib>:"PID Autotuning Design.vi"("Tuning specifications"="Tuning specifications 8", "Type of Controller"=w1943, "dt (s)"=w1946, "Response signal"=w1949, "Stimulus signal"=w1950) -> ("PID gains"=w1944:T2, "response offset"=w1947:dbl, "stimulus offset"=w1948:dbl, "Plant Parameters"=w1945:T4)  [unwired: 3 in]
      }
      frame "Internal Model Control" {
        n888 = call-poly <vilib>:"PID Autotuning Design.vi"("Desired Time Constant (tau_c)"="Multiplicative factor 8", "Type of Controller"=w1952, "dt (s)"=w1955, "Response signal"=w1958, "Stimulus signal"=w1959) -> ("PID gains"=w1953:T2, "response offset"=w1956:dbl, "stimulus offset"=w1957:dbl, "Plant Parameters"=w1954:T4)  [unwired: 3 in]
      }
    }
    "Stimulus operating point 8" <- w1911
    "Response operating point 8" <- w1910
    "Identified Plant Parameters 8" <- w1909
    n889 = Unbundle(w1914) -> ("proportional gain (Kc)"=w1917:dbl)  [unwired: 2 out]
    n890 = Equal?(x=w1917, y=inf) -> (x = y?=w1916:bool)
    n891 = feedback #35() -> (w1915:T2)  [unwired: 1 in]
    n892 = Select(t=w1915, s=w1916, f=w1914) -> (s? t:f=w1913:T2)
    "Tuned PID gains 8" <- w1913
    n893 = feedback-in #35(w1913) -> ()
    n894 = case shown="True" "Accept gain 8" {
      tunnel: w1913 -> [_ w1960]
      frame False {
      }
      frame True {
        n895 = local write "PID Gains 8"(w1960) -> ()
      }
    }
    n896 = local read "Stop 8"() -> (w1922:bool)
  }
  n897 = while {
    tunnel: w70 -> [_]
    tunnel: w66 -> [w1964]
    stop <- w1974 stop-if-true
    # "If dT and deadtime have similar values, the identification could evaluate deadtime as zero and this generates proportional gain equal to Inf. This code avoid gain changes in this situations."
    # "Autotuning Loop"
    n898 = local read "Control Output 7"() -> (w1976:dbl[])
    n899 = local read "Measurement 7"() -> (w1975:dbl[])
    n900 = case shown="\"Chien-Hrones-Reswick\"" "Control 7" {
      tunnel: w1976 -> [w1985 w1993 w2002 w2011]
      tunnel: w1975 -> [w1984 w1992 w2001 w2010]
      tunnel: [w1983 w1991 w2000 w2009] -> w1963
      tunnel: [w1982 w1990 w1999 w2008] -> w1962
      tunnel: w1964 -> [w1981 w1989 w1998 w2007]
      tunnel: [w1980 w1988 w1997 w2006] -> w1961
      tunnel: [w1979 w1987 w1996 w2005] -> w1966
      tunnel: "Type of controller 7" -> [w1978 w1986 w1995 w2004]
      frame "Ziegler-Nichols", Default {
        n901 = call-poly <vilib>:"PID Autotuning Design.vi"("Ziegler-Nichols Speed"="Ziegler-Nichols speed 7", "Type of Controller"=w1978, "dt (s)"=w1981, "Response signal"=w1984, "Stimulus signal"=w1985) -> ("PID gains"=w1979:T2, "response operating point"=w1982:dbl, "stimulus operating point"=w1983:dbl, "Plant Parameters"=w1980:T4)  [unwired: 3 in]
      }
      frame "Cohen-Coon" {
        n902 = call-poly <vilib>:"PID Autotuning Design.vi"("Type of Controller"=w1986, "dt (s)"=w1989, "Response signal"=w1992, "Stimulus signal"=w1993) -> ("PID gains"=w1987:T2, "response offset"=w1990:dbl, "stimulus offset"=w1991:dbl, "Plant Parameters"=w1988:T4)  [unwired: 4 in]
      }
      frame "Chien-Hrones-Reswick" {
        n903 = call-poly <vilib>:"PID Autotuning Design.vi"("Tuning specifications"="Tuning specifications 7", "Type of Controller"=w1995, "dt (s)"=w1998, "Response signal"=w2001, "Stimulus signal"=w2002) -> ("PID gains"=w1996:T2, "response offset"=w1999:dbl, "stimulus offset"=w2000:dbl, "Plant Parameters"=w1997:T4)  [unwired: 3 in]
      }
      frame "Internal Model Control" {
        n904 = call-poly <vilib>:"PID Autotuning Design.vi"("Desired Time Constant (tau_c)"="Multiplicative factor 7", "Type of Controller"=w2004, "dt (s)"=w2007, "Response signal"=w2010, "Stimulus signal"=w2011) -> ("PID gains"=w2005:T2, "response offset"=w2008:dbl, "stimulus offset"=w2009:dbl, "Plant Parameters"=w2006:T4)  [unwired: 3 in]
      }
    }
    "Stimulus operating point 7" <- w1963
    "Response operating point 7" <- w1962
    "Identified Plant Parameters 7" <- w1961
    n905 = Unbundle(w1966) -> ("proportional gain (Kc)"=w1969:dbl)  [unwired: 2 out]
    n906 = Equal?(x=w1969, y=inf) -> (x = y?=w1968:bool)
    n907 = feedback #36() -> (w1967:T2)  [unwired: 1 in]
    n908 = Select(t=w1967, s=w1968, f=w1966) -> (s? t:f=w1965:T2)
    "Tuned PID gains 7" <- w1965
    n909 = feedback-in #36(w1965) -> ()
    n910 = case shown="True" "Accept gain 7" {
      tunnel: w1965 -> [_ w2012]
      frame False {
      }
      frame True {
        n911 = local write "PID Gains 7"(w2012) -> ()
      }
    }
    n912 = local read "Stop 7"() -> (w1974:bool)
  }
  n913 = call <instrlib>:"PDI close.vi"("error in (no error)"=w119, "pDev"=w125) -> ("error out"=→"error out":errorcluster, "connected"=w120:bool)  [unwired: 8 out]
  n914 = local write "Connected"(w120) -> ()
